vi "Omniax_mDrive_XYZR_MM_BR_RES_2_NC.vi"() -> ()   [LabVIEW 2009]
uses:
  <vilib>/Instr/_visa.llb/VISA Configure Serial Port (Instr).vi
panel:
  out "X Scan Duration":dbl
  out "Y Scan Duration":dbl
  out "Z Scan Duration":dbl
  out "R Scan Duration":dbl
  out "R Backlash steps/sec":i32
  out "R Backlash":i32
  out "R Holding Current %":i32
  out "R Run Current %":i32
  out "R offset deg":dbl
  out "R deg/rev":dbl
  out "R steps/rev":u32
  out "R velocity PV step/sec":i32
  out "R MINPOS":i32=-94296
  out "R MAXPOS":i32=-34296
  out "R COM PORT":refnum<visa-resource-name>="COM5"
  in  "R Scan set":bool
  in  "R Scan Velocity SP deg/sec":dbl
  in  "R Scan Length SP deg":dbl
  in  "R Move Set":bool
  out "Reset R Motor Steps":i32
  in  "Reset R Position deg":dbl
  out "R Velocity MVdeg/sec":dbl
  in  "R Velocity SP deg/sec":dbl
  in  "R Position SP deg":dbl
  out "R Position MV deg":dbl
  out "R Scan velocity MV deg/sec":dbl format="%#_6f"
  out "R Scan length MV deg":dbl
  in  "R Scan Length SP steps":i32 min=0 max=6144000 step=100
  in  "R Scan OK":bool
  in  "R Velocity SP step/sec":i32 min=1 max=102400
  in  "R Scan Velocity SP steps/sec":i32=1 min=1 max=102400 step=1
  in  "R Go":bool
  in  "R Step SP":i32=-20000 min=0 max=6144000 step=500
  out "R Position deg PV":dbl
  out "R Step PV":i32 max=2000
  out "R Backlash corr":bool
  out "R in Motion":bool
  out "R Scan":bool
  out "R in Range":bool
  out "Z COM PORT":refnum<visa-resource-name>="COM5"
  out "Z Backlash steps/sec":i32
  out "Z Backlash":i32
  out "Z Holding Current %":i32
  out "Z Run Current %":i32
  out "Z offset mm":dbl
  out "Z mm/rev":dbl
  out "Z steps/rev":u32
  out "Z  velocity PV step/sec":i32
  out "Z MINPOS":i32=-94296
  out "Z MAXPOS":i32=-34296
  in  "Z Scan set":bool
  in  "Z Scan Velocity SP mm/sec":dbl
  in  "Z Scan Length SP mm":dbl
  in  "Z Move Set":bool
  out "Reset Z Motor Steps":i32
  in  "Reset Z Position mm":dbl
  out "Z Velocity MV mm/sec":dbl
  in  "Z Velocity SP mm/sec":dbl
  in  "Z Position SP mm":dbl
  out "Z Position MV mm":dbl
  out "Z Scan velocity MV mm/sec":dbl format="%#_6f"
  out "Z Scan length MV mm":dbl
  in  "Z Scan Length SP steps":i32 min=0 max=2048000 step=100
  in  "Z Scan OK":bool
  in  "Z Velocity SP step/sec":i32 min=1 max=102400
  in  "Z Scan Velocity SP steps/sec":i32=1 min=1 max=102400 step=1
  in  "Z Go":bool
  in  "Z Step SP":i32=-20000 min=0 max=2048000 step=500
  out "Z Position mm PV":dbl
  out "Z Step PV":i32 max=2000
  out "Z Backlash corr":bool
  out "Z in Motion":bool
  out "Z Scan":bool
  out "Z in Range":bool
  out "Reset X Motor Steps":i32
  in  "Reset X Position mm":dbl
  out "X Backlash corr":bool
  out "X  in Motion":bool
  out "X Scan":bool
  out "X  in Range":bool
  out "X Step PV":i32 max=2000
  out "X Position mm PV":dbl
  out "X velocity PV step/sec":i32
  in  "X Scan set":bool
  in  "X Scan Velocity SP mm/sec":dbl
  in  "X Scan Length SP mm":dbl
  in  "X Move Set":bool
  out "X Velocity MV mm/sec":dbl
  in  "X Velocity SP mm/sec":dbl
  in  "X Position SP mm":dbl
  out "X Position MV mm":dbl
  out "X Scan velocity MV mm/sec":dbl format="%#_6f"
  out "X Scan length MV mm":dbl
  in  "X Scan Length SP steps":i32 min=-460800 max=460800 step=100
  in  "X Scan OK":bool
  in  "X Velocity SP step/sec":i32 min=1 max=102400
  in  "X Scan Velocity SP steps/sec":i32=1 min=1 max=102400 step=1
  in  "X Go":bool
  in  "X Step SP":i32=-20000 min=-460800 max=460800 step=500
  out "X Backlash steps/sec":i32
  out "X Backlash":i32
  out "X Holding Current %":i32
  out "X Run Current %":i32
  out "X offset mm":dbl
  out "X mm/rev":dbl
  out "X steps/rev":u32
  out "X MAXPOS":i32=-34296
  out "X MINPOS":i32=-94296
  out "X COM PORT":refnum<visa-resource-name>="COM5"
  out "Y Backlash corr":bool
  in  "Y Scan set":bool
  in  "Y Scan Velocity SP mm/sec":dbl
  in  "Y Scan Length SP mm":dbl
  in  "Y Move Set":bool
  out "Y Backlash steps/sec":i32
  out "Y Backlash":i32
  out "Y in Motion":bool
  in  "Reset":bool
  out "Reset Y Motor Steps":i32
  in  "Reset Y Position mm":dbl
  out "Y Velocity MV mm/sec":dbl
  in  "Y Velocity SP mm/sec":dbl
  in  "Y Position SP mm":dbl
  out "Y Position MV mm":dbl
  out "Y Holding Current %":i32
  out "Y Run Current %":i32
  out "Y Scan velocity MV mm/sec":dbl format="%#_6f"
  out "Y Scan length MV mm":dbl
  in  "Scan Cancel":bool
  out "Y Position mm PV":dbl
  out "Y offset mm":dbl
  out "Y mm/rev":dbl
  out "Y steps/rev":u32
  out "Y velocity PV step/sec":i32
  in  "Y Scan Length SP steps":i32 min=-460800 max=460800 step=100
  out "Y Scan":bool
  in  "Y Scan OK":bool
  in  "Scan Go":bool
  in  "Y Velocity SP step/sec":i32 min=1 max=102400
  in  "Y Scan Velocity SP steps/sec":i32=1 min=1 max=102400 step=1
  in  "Stop":bool
  out "Y in Range":bool
  out "Y Step PV":i32 max=2000
  in  "Y Go":bool
  in  "Y Step SP":i32=-20000 min=-460800 max=460800 step=500
  out "Y MINPOS":i32=-94296
  out "Y MAXPOS":i32=-34296
  out "Y COM PORT":refnum<visa-resource-name>="COM5"
  # "L"
  # "M"
  # "B"
  # "S"
  # "MX"
  # "MY"
  # "MZ"
  # "MR"
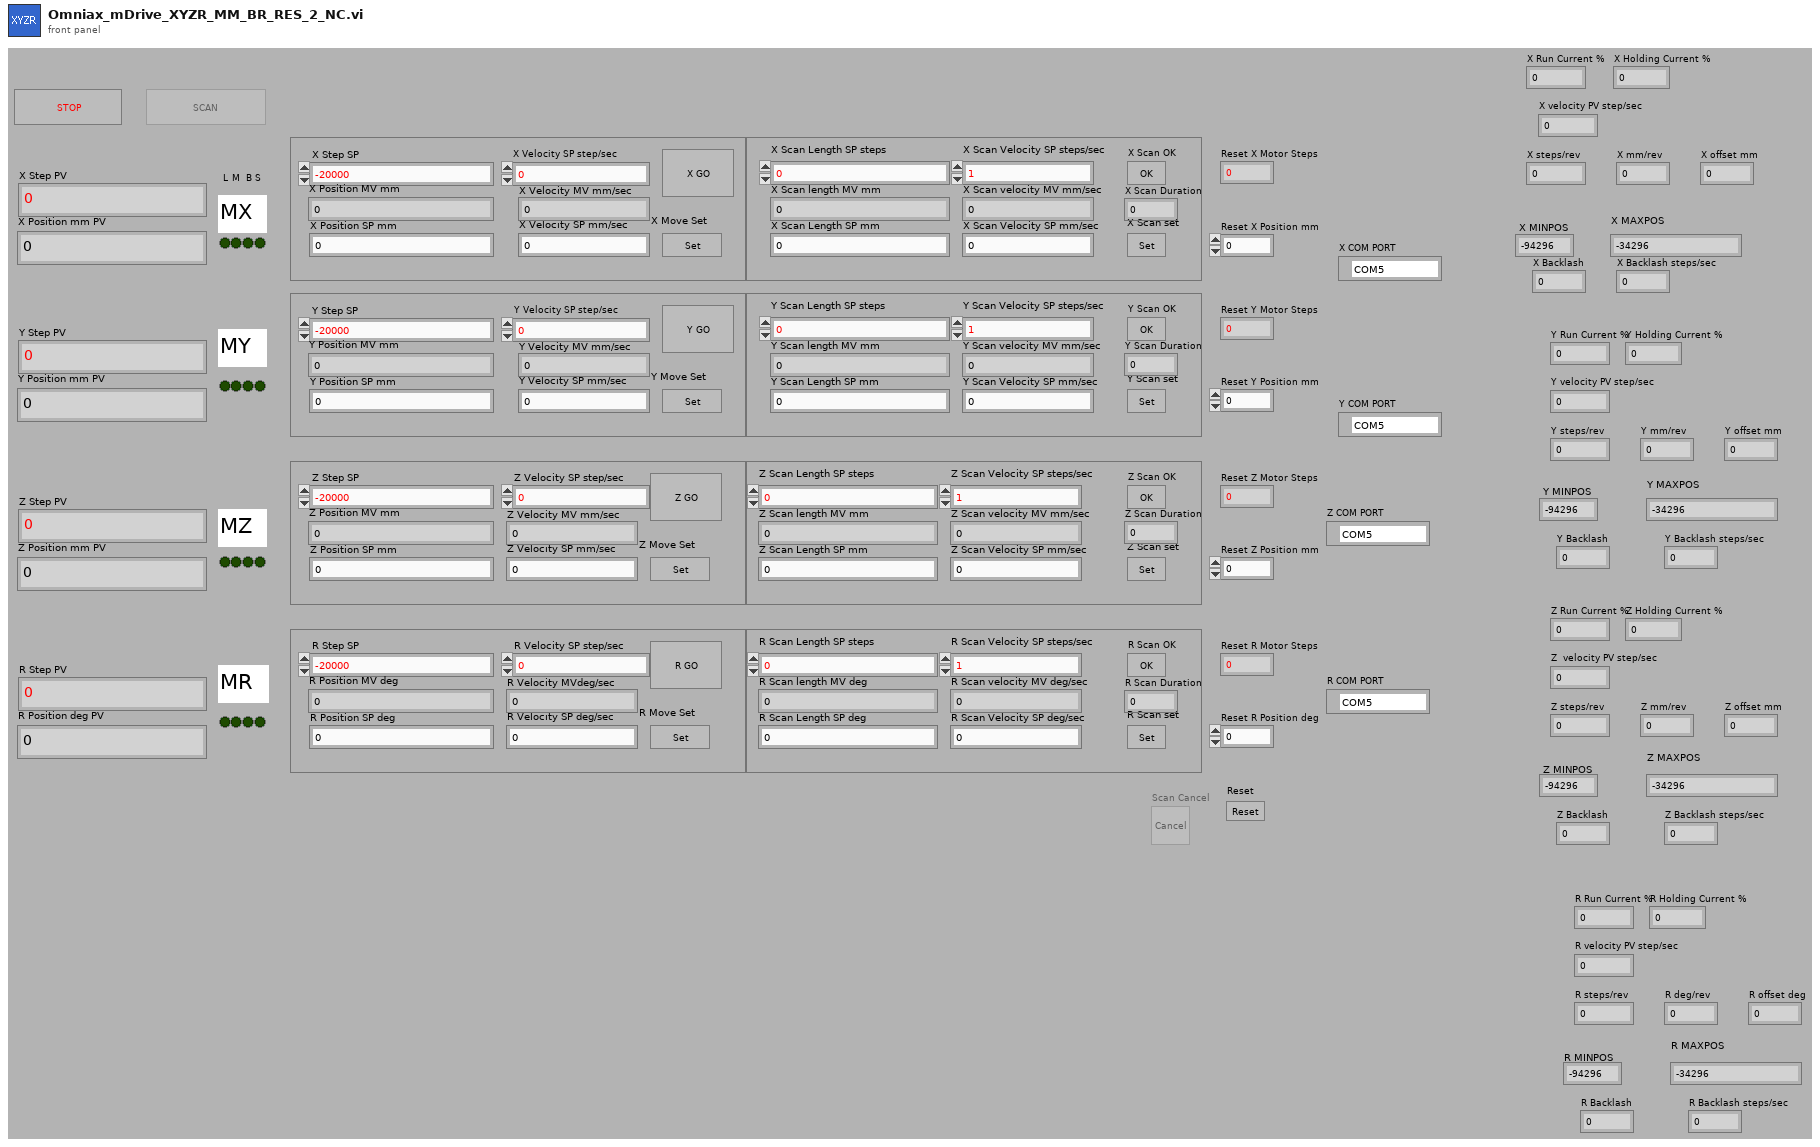
[diagram p1: front panel]
types:
  T1 = enum8{"Enabled", "Disabled", "Disabled and Grayed Out"}
  T2 = enum16{"Stop", "Reset", "Run Current", "Holding Current", "Accel Rate", "Decel Rate", "Move to Relative Position", "Move to Absolute Position", "Echo Mode", "Print Parameter", "Send String", "Microstep Resolution", "Set Current Position", "Max Velocity"}
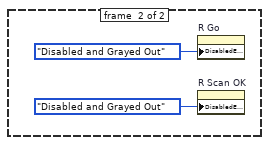
[diagram p2: hidden frame]
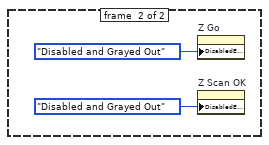
[diagram p5: hidden frame]
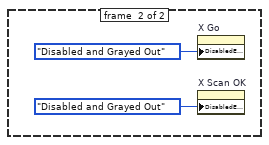
[diagram p8: hidden frame]
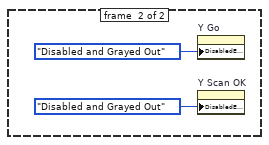
[diagram p11: hidden frame]
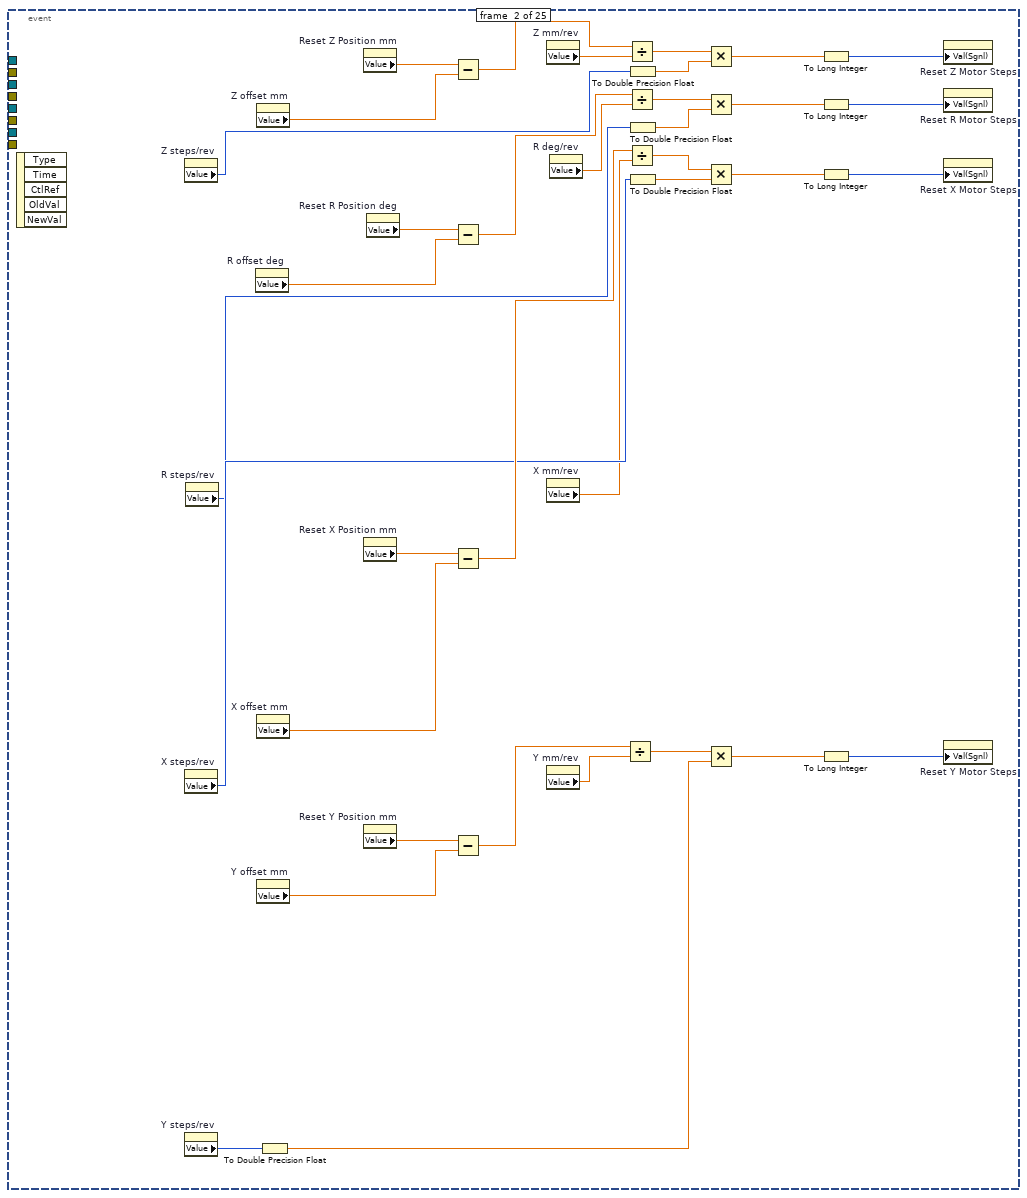
[diagram p14: hidden frame]
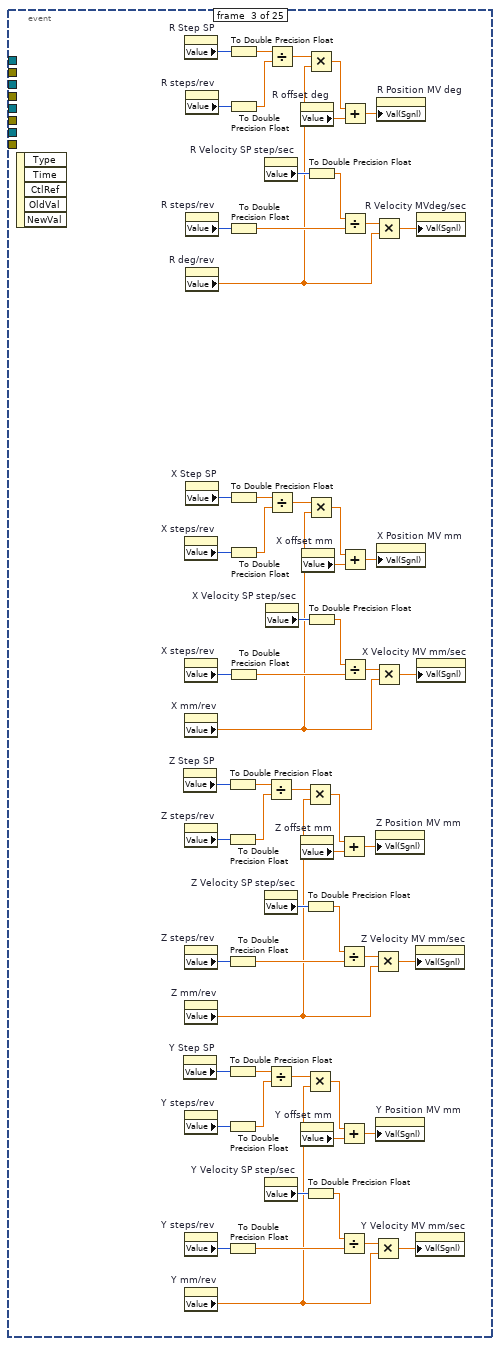
[diagram p15: hidden frame]
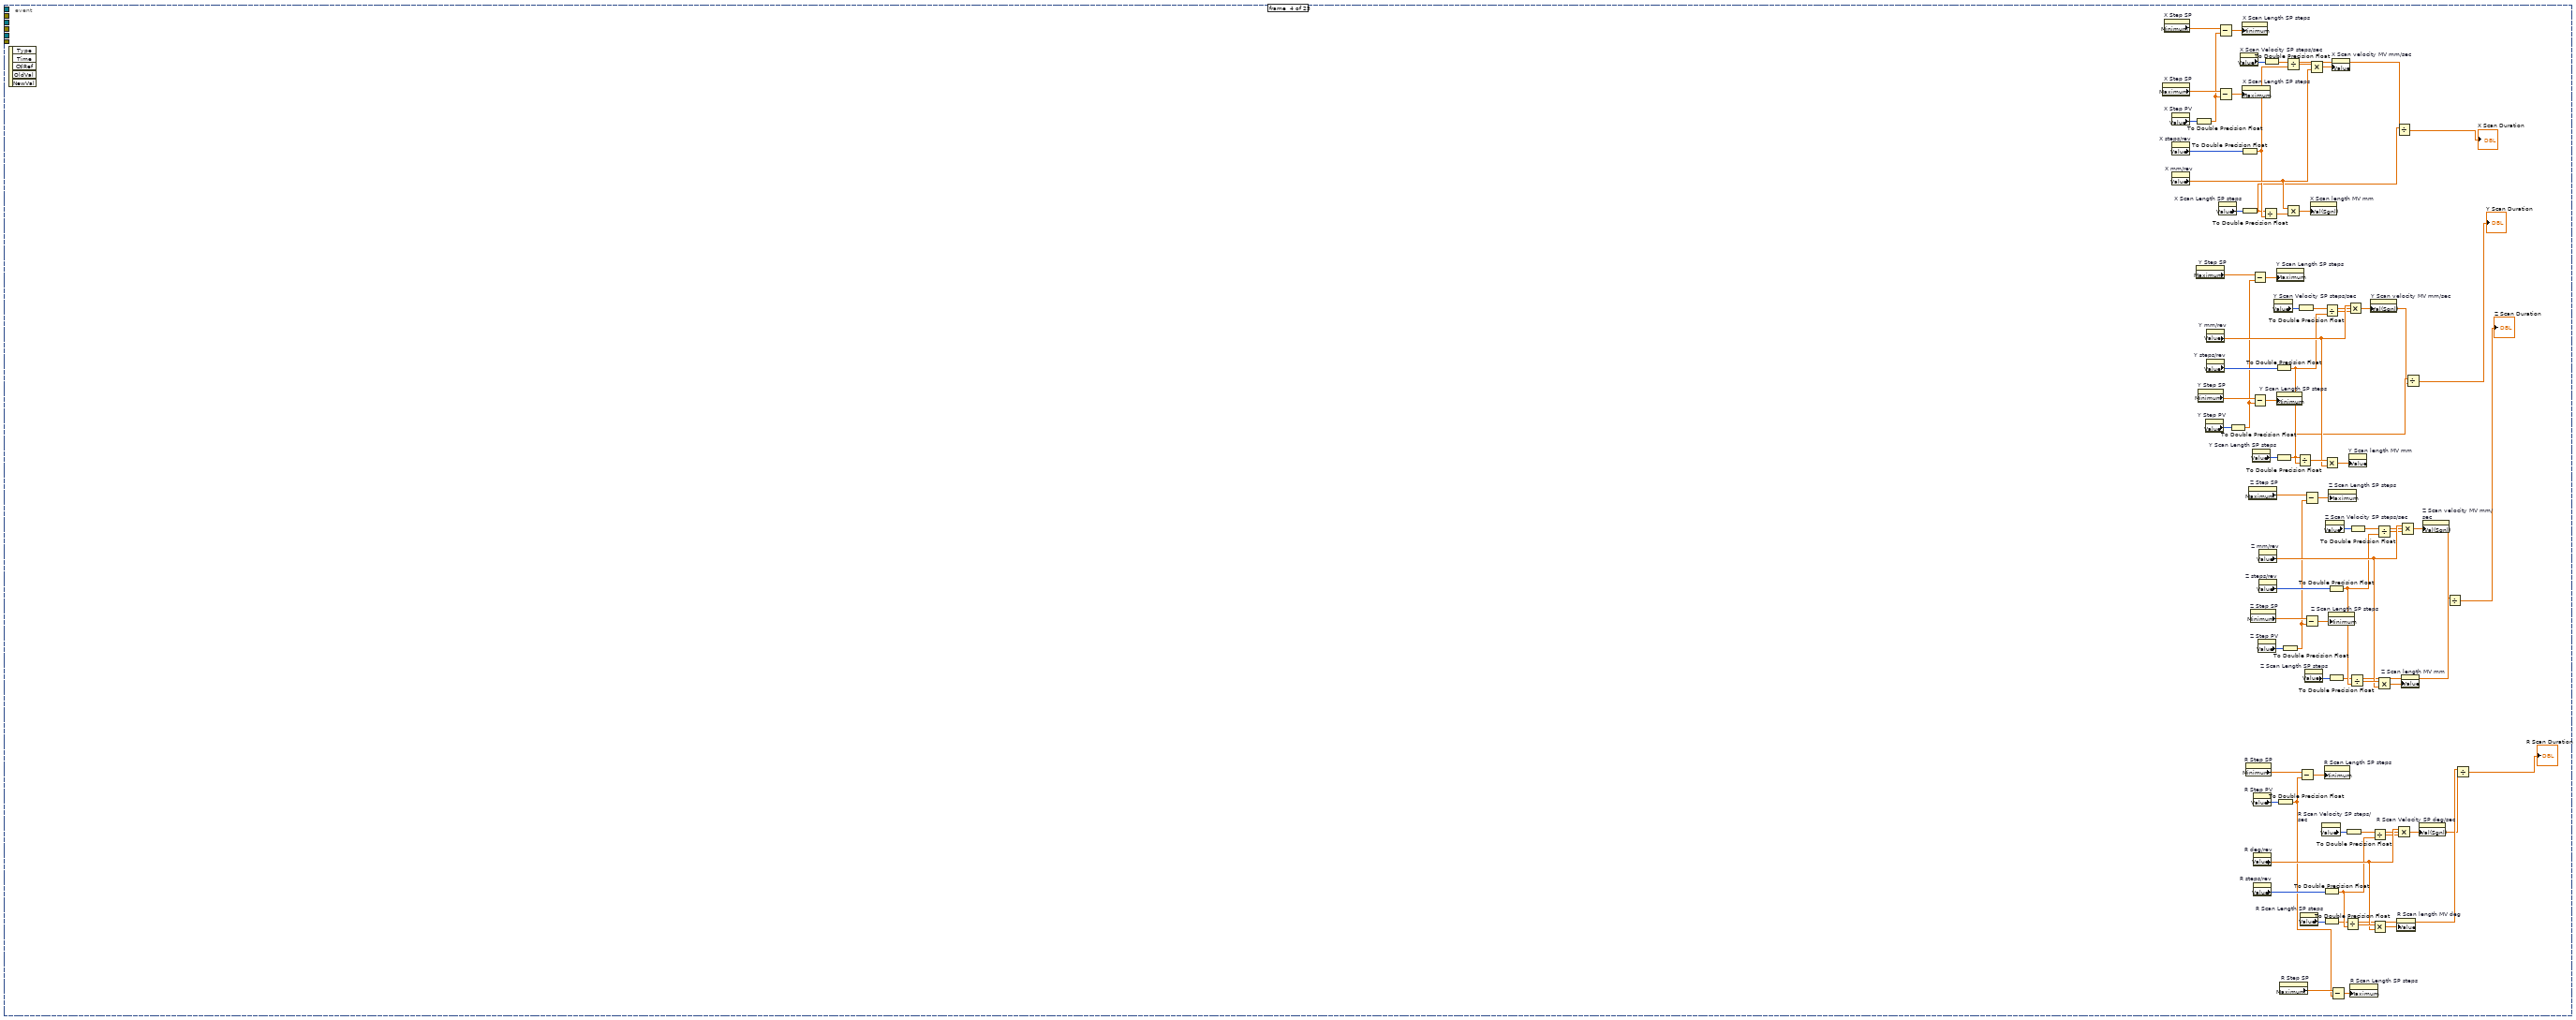
[diagram p16: hidden frame]
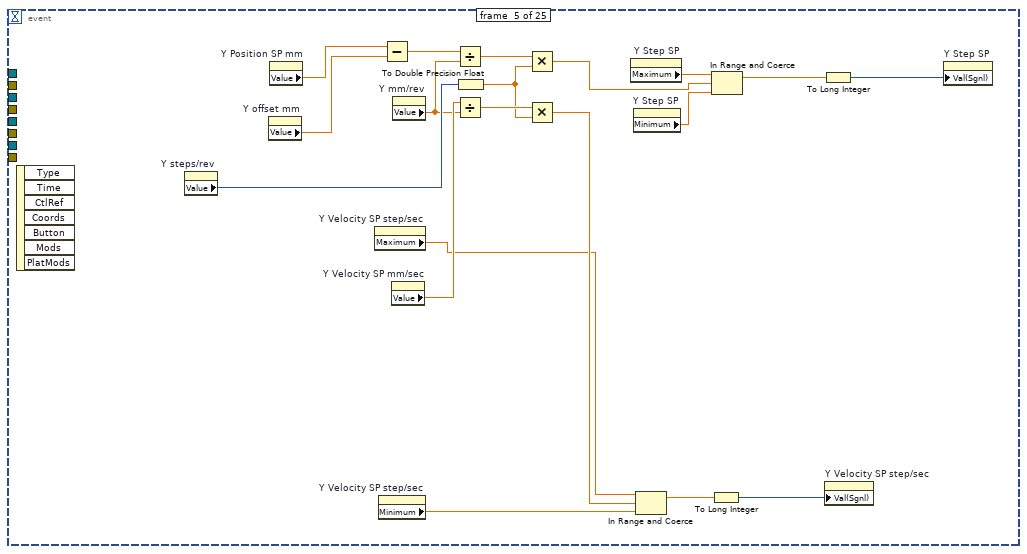
[diagram p17: hidden frame]
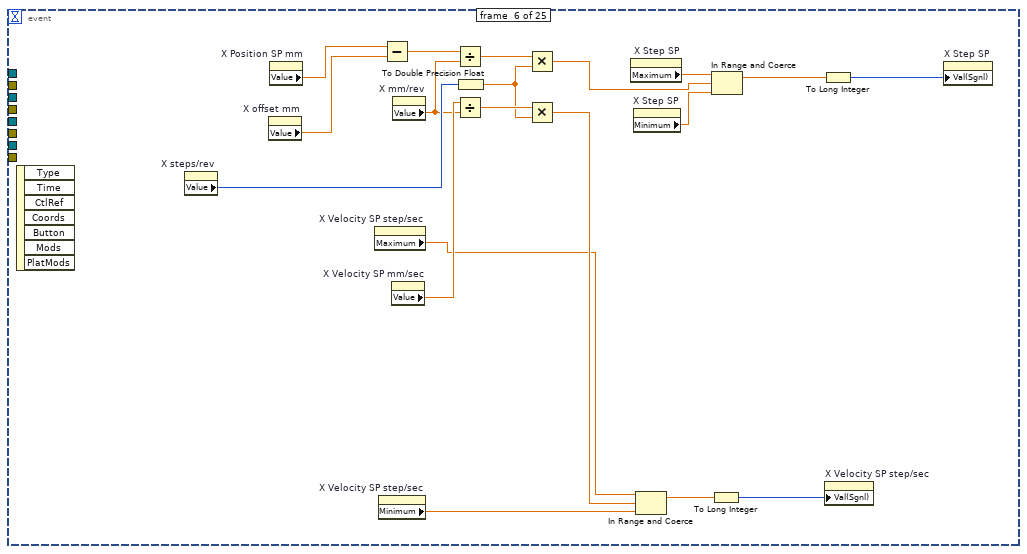
[diagram p18: hidden frame]
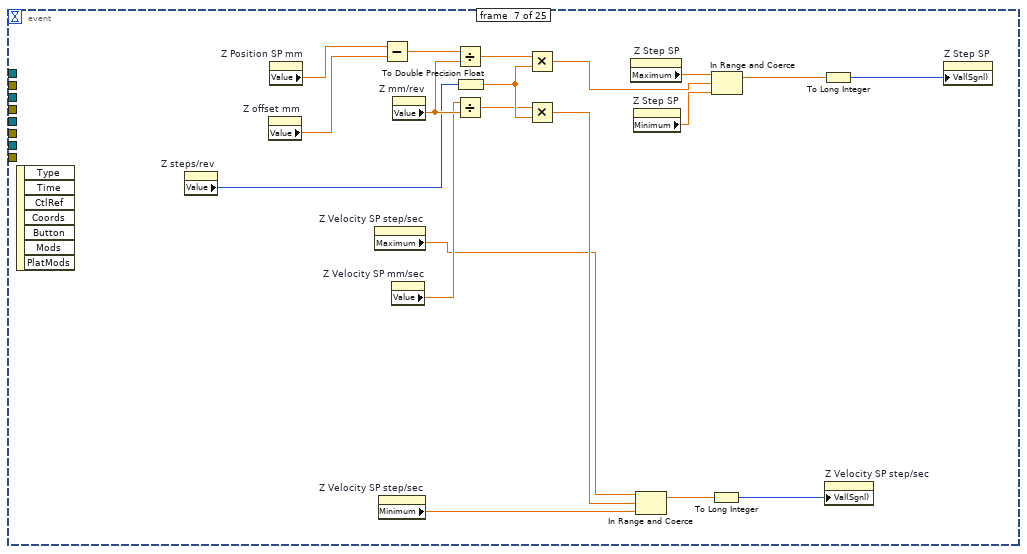
[diagram p19: hidden frame]
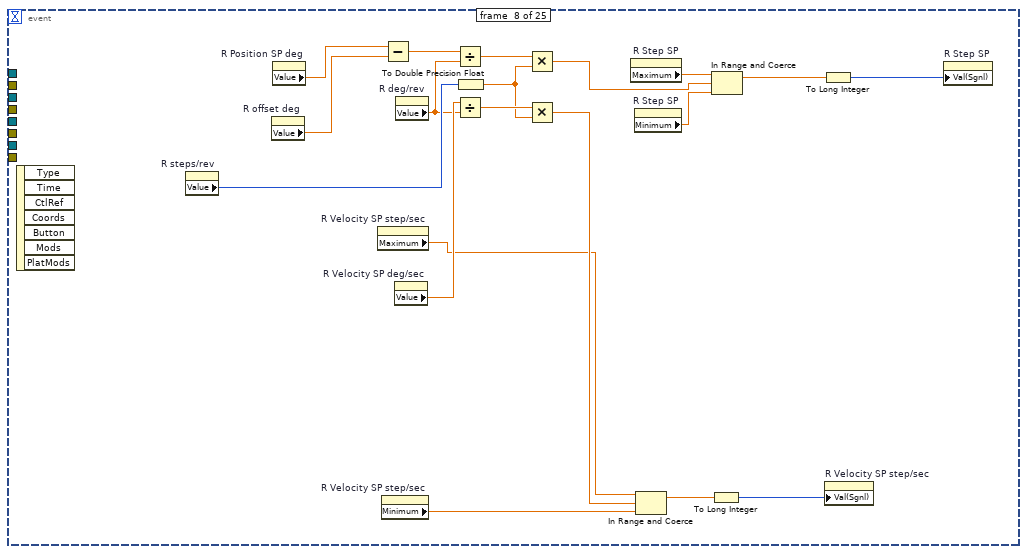
[diagram p20: hidden frame]
diagram:
  w19 = refnum<visa-resource-name> "COM11" ("COM PORT")
  w21 = u16 0 items=["None", "XON/XOFF", "RTS/CTS", "XON/XOFF & RTS/CTS", "DTR/DSR", "XON/XOFF & DTR/DSR"] ("flow control (0:none)")
  w22 = u16 10 items=["1.0"=10, "1.5"=15, "2.0"=20] ("stop bits (10: 1 bit)")
  w52 = refnum<visa-resource-name> "COM10" ("COM PORT")
  w54 = u16 0 items=["None", "XON/XOFF", "RTS/CTS", "XON/XOFF & RTS/CTS", "DTR/DSR", "XON/XOFF & DTR/DSR"] ("flow control (0:none)")
  w55 = u16 10 items=["1.0"=10, "1.5"=15, "2.0"=20] ("stop bits (10: 1 bit)")
  w65 = refnum<visa-resource-name> "COM8" ("COM PORT")
  w67 = u16 0 items=["None", "XON/XOFF", "RTS/CTS", "XON/XOFF & RTS/CTS", "DTR/DSR", "XON/XOFF & DTR/DSR"] ("flow control (0:none)")
  w68 = u16 10 items=["1.0"=10, "1.5"=15, "2.0"=20] ("stop bits (10: 1 bit)")
  w90 = refnum<visa-resource-name> "COM9" ("COM PORT")
  w92 = u16 0 items=["None", "XON/XOFF", "RTS/CTS", "XON/XOFF & RTS/CTS", "DTR/DSR", "XON/XOFF & DTR/DSR"] ("flow control (0:none)")
  w93 = u16 10 items=["1.0"=10, "1.5"=15, "2.0"=20] ("stop bits (10: 1 bit)")
  # "Stop bits"
  # "Stop bits"
  # "Stop bits"
  # "Stop bits"
  n1 = flat-sequence {
    frame #0 {
      w101 = 3.0 ("R deg/rev")
      w99 = u32 51200 ("step/rev")
      w103 = 102400 ("Value (Signaling)")
      n2 = property on="R Velocity SP step/sec" class="DigNum (strict)"("Val(Sgnl)"=w103) -> ()  [unwired: 2 in, 2 out]
      n3 = property on="R Velocity SP step/sec" class="DigNum (strict)"("Minimum"=1.0 ("Data Entry Limits:Minimum")) -> ()  [unwired: 2 in, 2 out]
      n4 = To Double Precision Float(number=w99) -> (double precision float=w100:dbl)
      n5 = To Double Precision Float(number=w103) -> (double precision float=w105:dbl)
      n6 = Divide(x=w105, y=w100) -> (x/y=w104:dbl)
      n7 = property on="R Velocity SP step/sec" class="DigNum (strict)"("Maximum"=w105) -> ()  [unwired: 2 in, 2 out]
      n8 = Multiply(x=w104, y=w101) -> (x*y=w102:dbl)
      n9 = property on="R Velocity SP deg/sec" class="DigNum (strict)"("Val(Sgnl)"=w102) -> ()  [unwired: 2 in, 2 out]
      "R offset deg" <- 0.0 ("R offset deg")
      "R deg/rev" <- w101
      "R steps/rev" <- w99
    }
  }
  n10 = flat-sequence {
    frame #0 {
      w108 = 1.0 ("MM/rev")
      w111 = u32 51200 ("step/rev")
      w106 = 102400 ("Value (Signaling)")
      n11 = property on="X Velocity SP step/sec" class="DigNum (strict)"("Minimum"=1.0 ("Data Entry Limits:Minimum")) -> ()  [unwired: 2 in, 2 out]
      n12 = property on="X Velocity SP step/sec" class="DigNum (strict)"("Val(Sgnl)"=w106) -> ()  [unwired: 2 in, 2 out]
      n13 = To Double Precision Float(number=w111) -> (double precision float=w110:dbl)
      n14 = To Double Precision Float(number=w106) -> (double precision float=w112:dbl)
      n15 = Divide(x=w112, y=w110) -> (x/y=w107:dbl)
      n16 = property on="X Velocity SP step/sec" class="DigNum (strict)"("Maximum"=w112) -> ()  [unwired: 2 in, 2 out]
      n17 = Multiply(x=w107, y=w108) -> (x*y=w109:dbl)
      n18 = property on="X Velocity SP mm/sec" class="DigNum (strict)"("Val(Sgnl)"=w109) -> ()  [unwired: 2 in, 2 out]
      "X offset mm" <- 0.0 ("offset")
      "X steps/rev" <- w111
      "X mm/rev" <- w108
    }
  }
  n19 = flat-sequence {
    frame #0 {
      w116 = 1.0 ("Z mm/rev")
      w115 = u32 51200 ("step/rev")
      w117 = 102400 ("Value (Signaling)")
      n20 = property on="Z Velocity SP step/sec" class="DigNum (strict)"("Val(Sgnl)"=w117) -> ()  [unwired: 2 in, 2 out]
      n21 = property on="Z Velocity SP step/sec" class="DigNum (strict)"("Minimum"=1.0 ("Data Entry Limits:Minimum")) -> ()  [unwired: 2 in, 2 out]
      n22 = To Double Precision Float(number=w115) -> (double precision float=w120:dbl)
      n23 = To Double Precision Float(number=w117) -> (double precision float=w121:dbl)
      n24 = Divide(x=w121, y=w120) -> (x/y=w118:dbl)
      n25 = property on="Z Velocity SP step/sec" class="DigNum (strict)"("Maximum"=w121) -> ()  [unwired: 2 in, 2 out]
      n26 = Multiply(x=w118, y=w116) -> (x*y=w119:dbl)
      n27 = property on="Z Velocity SP mm/sec" class="DigNum (strict)"("Val(Sgnl)"=w119) -> ()  [unwired: 2 in, 2 out]
      "Z offset mm" <- 0.0 ("Z offset mm")
      "Z mm/rev" <- w116
      "Z steps/rev" <- w115
    }
  }
  n28 = flat-sequence {
    frame #0 {
      n29 = property on="X Backlash corr" class="Bool (strict)"("Val(Sgnl)"=FALSE ("Value (Signaling)")) -> ()  [unwired: 2 in, 2 out]
      n30 = property on="Z Backlash corr" class="Bool (strict)"("Val(Sgnl)"=FALSE ("Value (Signaling)")) -> ()  [unwired: 2 in, 2 out]
      n31 = property on="Y Backlash corr" class="Bool (strict)"("Val(Sgnl)"=FALSE ("Value (Signaling)")) -> ()  [unwired: 2 in, 2 out]
      n32 = property on="R Backlash corr" class="Bool (strict)"("Val(Sgnl)"=FALSE ("Value (Signaling)")) -> ()  [unwired: 2 in, 2 out]
      "Z Backlash steps/sec" <- 25600 ("Z Backlash steps/sec")
      "Z Backlash" <- -12800 ("Z Backlash")
      "X Backlash steps/sec" <- 25600 ("Value (Signaling)")
      "X Backlash" <- -5120 ("Backlash2")
      "Y Backlash" <- -5120 ("Backlash2")
      "Y Backlash steps/sec" <- 25600 ("Value (Signaling)")
      "R Backlash steps/sec" <- 25600 ("R Backlash steps/sec")
      "R Backlash" <- -12800 ("R Backlash")
    }
  }
  n33 = flat-sequence {
    frame #0 {
      "Z Holding Current %" <- 20 ("Z Holding Current %")
      "Z Run Current %" <- 40 ("Z Run Current %")
      "X Run Current %" <- 40 ("Run Current %")
      "X Holding Current %" <- 20 ("Holding Current %")
      "Y Run Current %" <- 40 ("Run Current %")
      "Y Holding Current %" <- 20 ("Holding Current %")
      "R Holding Current %" <- 20 ("R Holding Current %")
      "R Run Current %" <- 40 ("R Run Current %")
    }
  }
  n34 = flat-sequence {
    frame #0 {
      n35 = property on="Y Scan" class="Bool (strict)"("Val(Sgnl)"=FALSE ("Value (Signaling)")) -> ()  [unwired: 2 in, 2 out]
      n36 = property on="Y Scan Velocity SP mm/sec" class="DigNum (strict)"("Val(Sgnl)"=0.1 ("Value (Signaling)")) -> ()  [unwired: 2 in, 2 out]
      n37 = property on="Z Scan Velocity SP mm/sec" class="DigNum (strict)"("Val(Sgnl)"=0.1 ("Value (Signaling)")) -> ()  [unwired: 2 in, 2 out]
      n38 = property on="R Scan" class="Bool (strict)"("Val(Sgnl)"=FALSE ("Value (Signaling)")) -> ()  [unwired: 2 in, 2 out]
      n39 = property on="Z Scan" class="Bool (strict)"("Val(Sgnl)"=FALSE ("Value (Signaling)")) -> ()  [unwired: 2 in, 2 out]
      n40 = property on="R Velocity SP deg/sec" class="DigNum (strict)"("Val(Sgnl)"=0.1 ("Value (Signaling)")) -> ()  [unwired: 2 in, 2 out]
      n41 = property on="X Scan" class="Bool (strict)"("Val(Sgnl)"=FALSE ("Value (Signaling)")) -> ()  [unwired: 2 in, 2 out]
      n42 = property on="X Scan Velocity SP mm/sec" class="DigNum (strict)"("Val(Sgnl)"=0.1 ("Value (Signaling)")) -> ()  [unwired: 2 in, 2 out]
      n43 = property on="Scan Go" class="Bool"("DisabledEnum"=T1."Disabled and Grayed Out" ("Disabled")) -> ()  [unwired: 2 in, 2 out]
      n44 = property on="Scan Cancel" class="Bool"("DisabledEnum"=T1."Disabled and Grayed Out" ("Disabled")) -> ()  [unwired: 2 in, 2 out]
    }
  }
  n45 = flat-sequence {
    frame #0 {
      w156 = 1.0 ("MM/rev")
      w159 = u32 51200 ("step/rev")
      w154 = 102400 ("Value (Signaling)")
      n46 = property on="Y Velocity SP step/sec" class="DigNum (strict)"("Minimum"=1.0 ("Data Entry Limits:Minimum")) -> ()  [unwired: 2 in, 2 out]
      n47 = property on="Y Velocity SP step/sec" class="DigNum (strict)"("Val(Sgnl)"=w154) -> ()  [unwired: 2 in, 2 out]
      n48 = To Double Precision Float(number=w159) -> (double precision float=w158:dbl)
      n49 = To Double Precision Float(number=w154) -> (double precision float=w160:dbl)
      n50 = Divide(x=w160, y=w158) -> (x/y=w155:dbl)
      n51 = property on="Y Velocity SP step/sec" class="DigNum (strict)"("Maximum"=w160) -> ()  [unwired: 2 in, 2 out]
      n52 = Multiply(x=w155, y=w156) -> (x*y=w157:dbl)
      n53 = property on="Y Velocity SP mm/sec" class="DigNum (strict)"("Val(Sgnl)"=w157) -> ()  [unwired: 2 in, 2 out]
      "Y offset mm" <- 0.0 ("offset")
      "Y steps/rev" <- w159
      "Y mm/rev" <- w156
    }
  }
  n54 = call-poly "VISA Configure Serial Port"("VISA resource name"=w90, "timeout (10sec)"=u32 10000, "baud rate (9600)"=u32 9600, "data bits (8)"=u16 8, "parity (0:none)"=enum16{"None", "Odd", "Even", "Mark", "Space"}."None", "stop bits (10: 1 bit)"=w93, "flow control (0:none)"=w92) -> ("VISA resource name out"=w83:refnum<visa-resource-name>, "error out"=w82:errorcluster)  [unwired: 7 in]
  n55 = flat-sequence {
    tunnel: w82 -> [w164]
    tunnel: w83 -> [w166]
    tunnel: [w165] -> w4
    tunnel: [w163] -> w3
    tunnel: [w172] -> w81
    tunnel: [w174] -> w79
    tunnel: w4 -> [w173]
    tunnel: w3 -> [w175]
    tunnel: w81 -> [w182]
    tunnel: [w181] -> w80
    tunnel: w79 -> [w179]
    tunnel: [w180] -> w78
    tunnel: [w192] -> w85
    tunnel: [w193] -> w84
    tunnel: w80 -> [w191]
    tunnel: w78 -> [w190]
    tunnel: w85 -> [w203]
    tunnel: w84 -> [w202]
    tunnel: [w205] -> w51
    tunnel: [w204] -> w50
    tunnel: [w199] -> w49
    tunnel: [w210] -> w88
    tunnel: [w211] -> w89
    tunnel: w51 -> [w211]
    tunnel: w50 -> [w210]
    tunnel: w49 -> [w206]
    frame #0 {
      n56 = call "mDrive Send Command.vi"("error in (no error)"=w164, "Extra"="EM=2", "Command"=T2."Send String", "VISA resource name"=w166) -> ("error out"=w163:errorcluster, "VISA resource name out"=w165:refnum<visa-resource-name>)  [unwired: 3 in, 1 out]
    }
    frame #1 {
      # "Run Current %"
      n57 = property on="Y Run Current %" class="DigNum (strict)"() -> ("Value"=w170:i32)  [unwired: 2 in, 2 out]
      n58 = Number To Decimal String(number=w170) -> (decimal integer string=w171:string)  [unwired: 1 in]
      n59 = call "mDrive Send Command.vi"("error in (no error)"=w175, "Extra"=w171, "Command"=T2."Run Current", "VISA resource name"=w173) -> ("error out"=w174:errorcluster, "VISA resource name out"=w172:refnum<visa-resource-name>)  [unwired: 3 in, 1 out]
    }
    frame #2 {
      # "Holding Current %"
      n60 = property on="Y Holding Current %" class="DigNum (strict)"() -> ("Value"=w177:i32)  [unwired: 2 in, 2 out]
      n61 = Number To Decimal String(number=w177) -> (decimal integer string=w178:string)  [unwired: 1 in]
      n62 = call "mDrive Send Command.vi"("error in (no error)"=w179, "Extra"=w178, "Command"=T2."Holding Current", "VISA resource name"=w182) -> ("error out"=w180:errorcluster, "VISA resource name out"=w181:refnum<visa-resource-name>)  [unwired: 3 in, 1 out]
    }
    frame #3 {
      # "Print Velocity Ma"
      # "Velocity Max"
      n63 = property on="Y Velocity SP step/sec" class="DigNum (strict)"() -> ("Value"=w189:i32)  [unwired: 2 in, 2 out]
      n64 = Number To Decimal String(number=w189) -> (decimal integer string=w188:string)  [unwired: 1 in]
      n65 = call "mDrive Send Command.vi"("error in (no error)"=w190, "Extra"=w188, "Command"=T2."Max Velocity", "VISA resource name"=w191) -> ("error out"=w186:errorcluster, "VISA resource name out"=w196:refnum<visa-resource-name>)  [unwired: 3 in, 1 out]
      n66 = call "mDrive Send Command.vi"("error in (no error)"=w186, "Extra"="VM", "Command"=T2."Print Parameter", "VISA resource name"=w196) -> ("error out"=w193:errorcluster, "read buffer"=w194:string, "VISA resource name out"=w192:refnum<visa-resource-name>)  [unwired: 3 in]
      n67 = Decimal String To Number(string=w194, offset=0) -> (number=w187:i32)  [unwired: 1 in, 1 out]
      n68 = property on="Y scan velocity MV step/sec" class="DigNum (strict)"("Val(Sgnl)"=w187) -> ()  [unwired: 2 in, 2 out]
    }
    frame #4 {
      # "PRINT POSITION"
      n69 = call "mDrive Send Command.vi"("error in (no error)"=w202, "Extra"="P", "Command"=T2."Print Parameter", "VISA resource name"=w203) -> ("error out"=w204:errorcluster, "read buffer"=w201:string, "VISA resource name out"=w205:refnum<visa-resource-name>)  [unwired: 3 in]
      n70 = Decimal String To Number(string=w201, offset=0) -> (number=w199:i32)  [unwired: 1 in, 1 out]
    }
    frame #5 {
      w208 = -460800 ("lower limit")
      w209 = 460800 ("upper limit")
      n71 = property on="Y Step SP" class="DigNum (strict)"("Val(Sgnl)"=w206) -> ()  [unwired: 2 in, 2 out]
      n72 = property on="Y Step SP" class="DigNum (strict)"("Maximum"=w209) -> ()  [unwired: 2 in, 2 out]
      n73 = property on="Y Step SP" class="DigNum (strict)"("Minimum"=w208) -> ()  [unwired: 2 in, 2 out]
      n74 = In Range and Coerce(upper limit=w209, x=w206, lower limit=w208) -> (In Range?=w207:bool)  [unwired: 1 out]
      n75 = property on="Y in Range" class="Bool (strict)"("Val(Sgnl)"=w207) -> ()  [unwired: 2 in, 2 out]
      "Y MINPOS" <- w208
      "Y MAXPOS" <- w209
    }
  }
  n76 = call-poly "VISA Configure Serial Port"("VISA resource name"=w65, "timeout (10sec)"=u32 10000, "baud rate (9600)"=u32 9600, "data bits (8)"=u16 8, "parity (0:none)"=enum16{"None", "Odd", "Even", "Mark", "Space"}."None", "stop bits (10: 1 bit)"=w68, "flow control (0:none)"=w67) -> ("VISA resource name out"=w64:refnum<visa-resource-name>, "error out"=w63:errorcluster)  [unwired: 7 in]
  n77 = call-poly "VISA Configure Serial Port"("VISA resource name"=w19, "timeout (10sec)"=u32 10000, "baud rate (9600)"=u32 9600, "data bits (8)"=u16 8, "parity (0:none)"=enum16{"None", "Odd", "Even", "Mark", "Space"}."None", "stop bits (10: 1 bit)"=w22, "flow control (0:none)"=w21) -> ("VISA resource name out"=w18:refnum<visa-resource-name>, "error out"=w17:errorcluster)  [unwired: 7 in]
  n78 = call-poly "VISA Configure Serial Port"("VISA resource name"=w52, "timeout (10sec)"=u32 10000, "baud rate (9600)"=u32 9600, "data bits (8)"=u16 8, "parity (0:none)"=enum16{"None", "Odd", "Even", "Mark", "Space"}."None", "stop bits (10: 1 bit)"=w55, "flow control (0:none)"=w54) -> ("VISA resource name out"=w36:refnum<visa-resource-name>, "error out"=w35:errorcluster)  [unwired: 7 in]
  n79 = flat-sequence {
    tunnel: w63 -> [w213]
    tunnel: w64 -> [w215]
    tunnel: [w214] -> w2
    tunnel: [w212] -> w1
    tunnel: [w221] -> w77
    tunnel: [w223] -> w76
    tunnel: w2 -> [w222]
    tunnel: w1 -> [w224]
    tunnel: w77 -> [w231]
    tunnel: [w230] -> w75
    tunnel: w76 -> [w228]
    tunnel: [w229] -> w74
    tunnel: [w241] -> w73
    tunnel: [w242] -> w72
    tunnel: w75 -> [w240]
    tunnel: w74 -> [w239]
    tunnel: w73 -> [w252]
    tunnel: w72 -> [w251]
    tunnel: [w254] -> w48
    tunnel: [w253] -> w47
    tunnel: [w248] -> w46
    tunnel: [w259] -> w61
    tunnel: [w260] -> w62
    tunnel: w48 -> [w260]
    tunnel: w47 -> [w259]
    tunnel: w46 -> [w255]
    frame #0 {
      n80 = call "mDrive Send Command.vi"("error in (no error)"=w213, "Extra"="EM=2", "Command"=T2."Send String", "VISA resource name"=w215) -> ("error out"=w212:errorcluster, "VISA resource name out"=w214:refnum<visa-resource-name>)  [unwired: 3 in, 1 out]
    }
    frame #1 {
      # "Run Current %"
      n81 = property on="X Run Current %" class="DigNum (strict)"() -> ("Value"=w219:i32)  [unwired: 2 in, 2 out]
      n82 = Number To Decimal String(number=w219) -> (decimal integer string=w220:string)  [unwired: 1 in]
      n83 = call "mDrive Send Command.vi"("error in (no error)"=w224, "Extra"=w220, "Command"=T2."Run Current", "VISA resource name"=w222) -> ("error out"=w223:errorcluster, "VISA resource name out"=w221:refnum<visa-resource-name>)  [unwired: 3 in, 1 out]
    }
    frame #2 {
      # "Holding Current %"
      n84 = property on="X Holding Current %" class="DigNum (strict)"() -> ("Value"=w226:i32)  [unwired: 2 in, 2 out]
      n85 = Number To Decimal String(number=w226) -> (decimal integer string=w227:string)  [unwired: 1 in]
      n86 = call "mDrive Send Command.vi"("error in (no error)"=w228, "Extra"=w227, "Command"=T2."Holding Current", "VISA resource name"=w231) -> ("error out"=w229:errorcluster, "VISA resource name out"=w230:refnum<visa-resource-name>)  [unwired: 3 in, 1 out]
    }
    frame #3 {
      # "Print Velocity Ma"
      # "Velocity Max"
      n87 = property on="X Velocity SP step/sec" class="DigNum (strict)"() -> ("Value"=w238:i32)  [unwired: 2 in, 2 out]
      n88 = Number To Decimal String(number=w238) -> (decimal integer string=w237:string)  [unwired: 1 in]
      n89 = call "mDrive Send Command.vi"("error in (no error)"=w239, "Extra"=w237, "Command"=T2."Max Velocity", "VISA resource name"=w240) -> ("error out"=w235:errorcluster, "VISA resource name out"=w245:refnum<visa-resource-name>)  [unwired: 3 in, 1 out]
      n90 = call "mDrive Send Command.vi"("error in (no error)"=w235, "Extra"="VM", "Command"=T2."Print Parameter", "VISA resource name"=w245) -> ("error out"=w242:errorcluster, "read buffer"=w243:string, "VISA resource name out"=w241:refnum<visa-resource-name>)  [unwired: 3 in]
      n91 = Decimal String To Number(string=w243, offset=0) -> (number=w236:i32)  [unwired: 1 in, 1 out]
      n92 = property on="X velocity PV step/sec" class="DigNum (strict)"("Val(Sgnl)"=w236) -> ()  [unwired: 2 in, 2 out]
    }
    frame #4 {
      # "PRINT POSITION"
      n93 = call "mDrive Send Command.vi"("error in (no error)"=w251, "Extra"="P", "Command"=T2."Print Parameter", "VISA resource name"=w252) -> ("error out"=w253:errorcluster, "read buffer"=w250:string, "VISA resource name out"=w254:refnum<visa-resource-name>)  [unwired: 3 in]
      n94 = Decimal String To Number(string=w250, offset=0) -> (number=w248:i32)  [unwired: 1 in, 1 out]
    }
    frame #5 {
      w257 = -460800 ("lower limit")
      w258 = 460800 ("upper limit")
      n95 = property on="X Step SP" class="DigNum (strict)"("Val(Sgnl)"=w255) -> ()  [unwired: 2 in, 2 out]
      n96 = property on="X Step SP" class="DigNum (strict)"("Maximum"=w258) -> ()  [unwired: 2 in, 2 out]
      n97 = property on="X Step SP" class="DigNum (strict)"("Minimum"=w257) -> ()  [unwired: 2 in, 2 out]
      n98 = In Range and Coerce(upper limit=w258, x=w255, lower limit=w257) -> (In Range?=w256:bool)  [unwired: 1 out]
      n99 = property on="X  in Range" class="Bool (strict)"("Val(Sgnl)"=w256) -> ()  [unwired: 2 in, 2 out]
      "X MINPOS" <- w257
      "X MAXPOS" <- w258
    }
  }
  n100 = flat-sequence {
    tunnel: w17 -> [w264]
    tunnel: w18 -> [w262]
    tunnel: [w261] -> w8
    tunnel: [w263] -> w7
    tunnel: [w271] -> w34
    tunnel: [w273] -> w33
    tunnel: w8 -> [w272]
    tunnel: w7 -> [w267]
    tunnel: w34 -> [w280]
    tunnel: [w279] -> w32
    tunnel: w33 -> [w277]
    tunnel: [w278] -> w31
    tunnel: [w290] -> w30
    tunnel: [w291] -> w29
    tunnel: w32 -> [w289]
    tunnel: w31 -> [w288]
    tunnel: w30 -> [w301]
    tunnel: w29 -> [w300]
    tunnel: [w303] -> w28
    tunnel: [w302] -> w27
    tunnel: [w297] -> w26
    tunnel: [w308] -> w11
    tunnel: [w309] -> w12
    tunnel: w28 -> [w309]
    tunnel: w27 -> [w308]
    tunnel: w26 -> [w306]
    frame #0 {
      n101 = call "mDrive Send Command.vi"("error in (no error)"=w264, "Extra"="EM=2", "Command"=T2."Send String", "VISA resource name"=w262) -> ("error out"=w263:errorcluster, "VISA resource name out"=w261:refnum<visa-resource-name>)  [unwired: 3 in, 1 out]
    }
    frame #1 {
      # "Run Current %"
      n102 = property on="R Run Current %" class="DigNum (strict)"() -> ("Value"=w269:i32)  [unwired: 2 in, 2 out]
      n103 = Number To Decimal String(number=w269) -> (decimal integer string=w270:string)  [unwired: 1 in]
      n104 = call "mDrive Send Command.vi"("error in (no error)"=w267, "Extra"=w270, "Command"=T2."Run Current", "VISA resource name"=w272) -> ("error out"=w273:errorcluster, "VISA resource name out"=w271:refnum<visa-resource-name>)  [unwired: 3 in, 1 out]
    }
    frame #2 {
      # "Holding Current %"
      n105 = property on="R Holding Current %" class="DigNum (strict)"() -> ("Value"=w275:i32)  [unwired: 2 in, 2 out]
      n106 = Number To Decimal String(number=w275) -> (decimal integer string=w276:string)  [unwired: 1 in]
      n107 = call "mDrive Send Command.vi"("error in (no error)"=w277, "Extra"=w276, "Command"=T2."Holding Current", "VISA resource name"=w280) -> ("error out"=w278:errorcluster, "VISA resource name out"=w279:refnum<visa-resource-name>)  [unwired: 3 in, 1 out]
    }
    frame #3 {
      # "Print Velocity Ma"
      # "Velocity Max"
      n108 = property on="R Velocity SP step/sec" class="DigNum (strict)"() -> ("Value"=w287:i32)  [unwired: 2 in, 2 out]
      n109 = Number To Decimal String(number=w287) -> (decimal integer string=w286:string)  [unwired: 1 in]
      n110 = call "mDrive Send Command.vi"("error in (no error)"=w288, "Extra"=w286, "Command"=T2."Max Velocity", "VISA resource name"=w289) -> ("error out"=w284:errorcluster, "VISA resource name out"=w294:refnum<visa-resource-name>)  [unwired: 3 in, 1 out]
      n111 = call "mDrive Send Command.vi"("error in (no error)"=w284, "Extra"="VM", "Command"=T2."Print Parameter", "VISA resource name"=w294) -> ("error out"=w291:errorcluster, "read buffer"=w292:string, "VISA resource name out"=w290:refnum<visa-resource-name>)  [unwired: 3 in]
      n112 = Decimal String To Number(string=w292, offset=0) -> (number=w285:i32)  [unwired: 1 in, 1 out]
      n113 = property on="R velocity PV step/sec" class="DigNum (strict)"("Val(Sgnl)"=w285) -> ()  [unwired: 2 in, 2 out]
    }
    frame #4 {
      # "PRINT POSITION"
      n114 = call "mDrive Send Command.vi"("error in (no error)"=w300, "Extra"="P", "Command"=T2."Print Parameter", "VISA resource name"=w301) -> ("error out"=w302:errorcluster, "read buffer"=w299:string, "VISA resource name out"=w303:refnum<visa-resource-name>)  [unwired: 3 in]
      n115 = Decimal String To Number(string=w299, offset=0) -> (number=w297:i32)  [unwired: 1 in, 1 out]
    }
    frame #5 {
      w305 = 0 ("lower limit")
      w304 = 6144000 ("upper limit")
      n116 = property on="R Step SP" class="DigNum (strict)"("Val(Sgnl)"=w306) -> ()  [unwired: 2 in, 2 out]
      n117 = property on="R Step SP" class="DigNum (strict)"("Maximum"=w304) -> ()  [unwired: 2 in, 2 out]
      n118 = property on="R Step SP" class="DigNum (strict)"("Minimum"=w305) -> ()  [unwired: 2 in, 2 out]
      n119 = In Range and Coerce(upper limit=w304, x=w306, lower limit=w305) -> (In Range?=w307:bool)  [unwired: 1 out]
      n120 = property on="R in Range" class="Bool (strict)"("Val(Sgnl)"=w307) -> ()  [unwired: 2 in, 2 out]
      "R MINPOS" <- w305
      "R MAXPOS" <- w304
    }
  }
  n121 = flat-sequence {
    tunnel: w35 -> [w310]
    tunnel: w36 -> [w313]
    tunnel: [w312] -> w6
    tunnel: [w311] -> w5
    tunnel: [w319] -> w45
    tunnel: [w321] -> w44
    tunnel: w6 -> [w320]
    tunnel: w5 -> [w322]
    tunnel: w45 -> [w329]
    tunnel: [w328] -> w43
    tunnel: w44 -> [w326]
    tunnel: [w327] -> w42
    tunnel: [w339] -> w41
    tunnel: [w340] -> w40
    tunnel: w43 -> [w338]
    tunnel: w42 -> [w337]
    tunnel: w41 -> [w350]
    tunnel: w40 -> [w349]
    tunnel: [w352] -> w39
    tunnel: [w351] -> w38
    tunnel: [w346] -> w37
    tunnel: [w357] -> w15
    tunnel: [w358] -> w16
    tunnel: w39 -> [w358]
    tunnel: w38 -> [w357]
    tunnel: w37 -> [w355]
    frame #0 {
      n122 = call "mDrive Send Command.vi"("error in (no error)"=w310, "Extra"="EM=2", "Command"=T2."Send String", "VISA resource name"=w313) -> ("error out"=w311:errorcluster, "VISA resource name out"=w312:refnum<visa-resource-name>)  [unwired: 3 in, 1 out]
    }
    frame #1 {
      # "Run Current %"
      n123 = property on="Z Run Current %" class="DigNum (strict)"() -> ("Value"=w317:i32)  [unwired: 2 in, 2 out]
      n124 = Number To Decimal String(number=w317) -> (decimal integer string=w318:string)  [unwired: 1 in]
      n125 = call "mDrive Send Command.vi"("error in (no error)"=w322, "Extra"=w318, "Command"=T2."Run Current", "VISA resource name"=w320) -> ("error out"=w321:errorcluster, "VISA resource name out"=w319:refnum<visa-resource-name>)  [unwired: 3 in, 1 out]
    }
    frame #2 {
      # "Holding Current %"
      n126 = property on="Z Run Current %" class="DigNum (strict)"() -> ("Value"=w324:i32)  [unwired: 2 in, 2 out]
      n127 = Number To Decimal String(number=w324) -> (decimal integer string=w325:string)  [unwired: 1 in]
      n128 = call "mDrive Send Command.vi"("error in (no error)"=w326, "Extra"=w325, "Command"=T2."Holding Current", "VISA resource name"=w329) -> ("error out"=w327:errorcluster, "VISA resource name out"=w328:refnum<visa-resource-name>)  [unwired: 3 in, 1 out]
    }
    frame #3 {
      # "Print Velocity Ma"
      # "Velocity Max"
      n129 = property on="Z Velocity SP step/sec" class="DigNum (strict)"() -> ("Value"=w336:i32)  [unwired: 2 in, 2 out]
      n130 = Number To Decimal String(number=w336) -> (decimal integer string=w335:string)  [unwired: 1 in]
      n131 = call "mDrive Send Command.vi"("error in (no error)"=w337, "Extra"=w335, "Command"=T2."Max Velocity", "VISA resource name"=w338) -> ("error out"=w333:errorcluster, "VISA resource name out"=w343:refnum<visa-resource-name>)  [unwired: 3 in, 1 out]
      n132 = call "mDrive Send Command.vi"("error in (no error)"=w333, "Extra"="VM", "Command"=T2."Print Parameter", "VISA resource name"=w343) -> ("error out"=w340:errorcluster, "read buffer"=w341:string, "VISA resource name out"=w339:refnum<visa-resource-name>)  [unwired: 3 in]
      n133 = Decimal String To Number(string=w341, offset=0) -> (number=w334:i32)  [unwired: 1 in, 1 out]
      n134 = property on="Z  velocity PV step/sec" class="DigNum (strict)"("Val(Sgnl)"=w334) -> ()  [unwired: 2 in, 2 out]
    }
    frame #4 {
      # "PRINT POSITION"
      n135 = call "mDrive Send Command.vi"("error in (no error)"=w349, "Extra"="P", "Command"=T2."Print Parameter", "VISA resource name"=w350) -> ("error out"=w351:errorcluster, "read buffer"=w348:string, "VISA resource name out"=w352:refnum<visa-resource-name>)  [unwired: 3 in]
      n136 = Decimal String To Number(string=w348, offset=0) -> (number=w346:i32)  [unwired: 1 in, 1 out]
    }
    frame #5 {
      w353 = 0 ("lower limit")
      w354 = 2048000 ("upper limit")
      n137 = property on="Z Step SP" class="DigNum (strict)"("Val(Sgnl)"=w355) -> ()  [unwired: 2 in, 2 out]
      n138 = property on="Z Step SP" class="DigNum (strict)"("Maximum"=w354) -> ()  [unwired: 2 in, 2 out]
      n139 = property on="Z Step SP" class="DigNum (strict)"("Minimum"=w353) -> ()  [unwired: 2 in, 2 out]
      n140 = In Range and Coerce(upper limit=w354, x=w355, lower limit=w353) -> (In Range?=w356:bool)  [unwired: 1 out]
      n141 = property on="Z in Range" class="Bool (strict)"("Val(Sgnl)"=w356) -> ()  [unwired: 2 in, 2 out]
      "Z MINPOS" <- w353
      "Z MAXPOS" <- w354
    }
  }
  n142 = while {
    tunnel: w89 -> [w372]
    tunnel: w88 -> [w375]
    tunnel: [w376] -> w86
    tunnel: [w374] -> w87
    tunnel: w62 -> [w370]
    tunnel: w61 -> [w369]
    tunnel: [w368] -> w60
    tunnel: [w367] -> w59
    tunnel: w16 -> [w366]
    tunnel: w15 -> [w365]
    tunnel: [w364] -> w14
    tunnel: [w363] -> w13
    tunnel: w12 -> [w362]
    tunnel: w11 -> [w361]
    tunnel: [w360] -> w10
    tunnel: [w359] -> w9
    stop <- w371 stop-if-true
    n143 = flat-sequence {
      frame #0 {
      }
    }
    n144 = flat-sequence {
      frame #0 {
      }
    }
    n145 = flat-sequence {
      frame #0 {
      }
    }
    n146 = flat-sequence {
      frame #0 {
      }
    }
    n147 = flat-sequence {
      frame #0 {
      }
    }
    n148 = event shown="[16] \"X Scan OK\": Mouse Up" {
      selector: _ -> [_ _ _ _ _ _ _ _ _ _ _ _ _ _ _ _ _ _ _ _ _ _ _ _ _]
      dyn-events: _ -> [_ _ _ _ _ _ _ _ _ _ _ _ _ _ _ _ _ _ _ _ _ _ _ _ _]
      timeout: 200 -> [_ _ _ _ _ _ _ _ _ _ _ _ _ _ _ _ _ _ _ _ _ _ _ _ _]
      tunnel: w375 -> [w436 _ _ _ _ _ _ _ _ _ _ _ w1261 _ _ _ _ w1510 _ _ w1606 w1622 w1666 w1743 w1987]
      tunnel: [w435 _ _ _ _ _ _ _ _ _ _ _ w1267 _ _ _ _ w1508 _ _ w1606 w1620 w1668 w1732 w1985] -> w376
      tunnel: w372 -> [w433 _ _ _ _ _ _ _ _ _ _ _ w1262 _ _ _ _ w1509 _ _ w1607 w1623 w1667 w1745 w1988]
      tunnel: [w434 _ _ _ _ _ _ _ _ _ _ _ w1268 _ _ _ _ w1505 _ _ w1607 w1621 w1669 w1733 w1986] -> w374
      tunnel: [_ _ _ _ _ _ _ _ _ _ _ _ _ _ _ _ _ _ _ _ TRUE _ _ _ _] -> w371
      tunnel: w370 -> [w410 _ _ _ _ _ _ _ _ _ _ _ _ _ _ w1419 w1474 _ _ _ _ w1617 w1659 w1749 w1984]
      tunnel: w369 -> [w409 _ _ _ _ _ _ _ _ _ _ _ _ _ _ w1418 w1473 _ _ _ _ w1616 w1658 w1747 w1983]
      tunnel: [w408 _ _ _ _ _ _ _ _ _ _ _ _ _ _ w1417 w1472 _ _ _ _ w1619 w1657 w1725 w1982] -> w368
      tunnel: [w407 _ _ _ _ _ _ _ _ _ _ _ _ _ _ w1416 w1471 _ _ _ _ w1618 w1656 w1723 w1981] -> w367
      tunnel: w366 -> [w381 _ _ _ _ _ _ _ _ _ _ _ _ w1313 _ _ _ _ w1540 _ _ w1615 w1653 w1741 w1980]
      tunnel: w365 -> [w384 _ _ _ _ _ _ _ _ _ _ _ _ w1312 _ _ _ _ w1539 _ _ w1614 w1652 w1739 w1979]
      tunnel: [w383 _ _ _ _ _ _ _ _ _ _ _ _ w1310 _ _ _ _ w1537 _ _ w1613 w1651 w1731 w1976] -> w364
      tunnel: [w382 _ _ _ _ _ _ _ _ _ _ _ _ w1311 _ _ _ _ w1538 _ _ w1612 w1650 w1730 w1975] -> w363
      tunnel: w362 -> [w380 _ _ _ _ _ _ _ _ _ _ _ _ _ w1366 _ _ _ _ w1574 _ w1611 w1647 w1736 w1978]
      tunnel: w361 -> [w379 _ _ _ _ _ _ _ _ _ _ _ _ _ w1365 _ _ _ _ w1573 _ w1610 w1646 w1734 w1977]
      tunnel: [w378 _ _ _ _ _ _ _ _ _ _ _ _ _ w1363 _ _ _ _ w1572 _ w1609 w1645 w1728 w1974] -> w360
      tunnel: [w377 _ _ _ _ _ _ _ _ _ _ _ _ _ w1364 _ _ _ _ w1571 _ w1608 w1644 w1727 w1973] -> w359
      event #0 {
        n149 = event-data() -> ()  [unwired: 1 in, 2 out]
        n150 = flat-sequence {
          tunnel: [w726] -> w421
          tunnel: [w702] -> w420
          tunnel: [w715] -> w419
          tunnel: [w693] -> w418
          tunnel: w410 -> [w692]
          tunnel: w409 -> [w691]
          tunnel: w421 -> [w732]
          tunnel: [w732] -> w417
          tunnel: w420 -> [w731]
          tunnel: [w731] -> w416
          tunnel: w419 -> [w730]
          tunnel: [w730] -> w415
          tunnel: w418 -> [w727]
          tunnel: [w727] -> w414
          tunnel: w417 -> [w739]
          tunnel: [w740] -> w413
          tunnel: w416 -> [w742]
          tunnel: [w741] -> w412
          tunnel: w415 -> [w738]
          tunnel: [w737] -> w411
          tunnel: w414 -> [w737]
          tunnel: w413 -> [w752]
          tunnel: w412 -> [w753]
          tunnel: w411 -> [w755]
          tunnel: [w751] -> w407
          tunnel: [w750] -> w408
          frame #0 {
            w697 = 0.05 ("Delay Time (s)")
            n151 = property on="X Step SP" class="DigNum (strict)"() -> ("Maximum"=w717:dbl)  [unwired: 2 in, 2 out]
            n152 = property on="X Step SP" class="DigNum (strict)"() -> ("Minimum"=w719:dbl)  [unwired: 2 in, 2 out]
            n153 = property on="X steps/rev" class="DigNum (strict)"() -> ("Value"=w713:u32)  [unwired: 2 in, 2 out]
            n154 = property on="X offset mm" class="DigNum (strict)"() -> ("Value"=w709:dbl)  [unwired: 2 in, 2 out]
            n155 = To Long Integer(number=w717) -> (32bit integer=w716:i32)
            n156 = To Long Integer(number=w719) -> (32bit integer=w718:i32)
            n157 = To Double Precision Float(number=w713) -> (double precision float=w714:dbl)
            n158 = call "mDrive Send Command.vi"("error in (no error)"=w691, "Extra"="P", "Command"=T2."Print Parameter", "VISA resource name"=w692) -> ("error out"=w721:errorcluster, "read buffer"=w725:string, "VISA resource name out"=w723:refnum<visa-resource-name>)  [unwired: 3 in]
            n159 = call "Time Delay12"("error in (no error)"=w721, "Delay Time (s)"=w697) -> ("error out"=w720:errorcluster)  [unwired: 9 in]
            n160 = Decimal String To Number(string=w725, offset=0) -> (number=w705:i32)  [unwired: 1 in, 1 out]
            n161 = To Long Integer(number=w705) -> (32bit integer=w707:i32)
            n162 = property on="X Step PV" class="DigNum (strict)"("Val(Sgnl)"=w707) -> ()  [unwired: 2 in, 2 out]
            n163 = call "mDrive Send Command.vi"("error in (no error)"=w720, "Extra"="MV", "Command"=T2."Print Parameter", "VISA resource name"=w723) -> ("error out"=w722:errorcluster, "read buffer"=w703:string, "VISA resource name out"=w726:refnum<visa-resource-name>)  [unwired: 3 in]
            n164 = call "Time Delay11"("error in (no error)"=w722, "Delay Time (s)"=w697) -> ("error out"=w702:errorcluster)  [unwired: 9 in]
            n165 = In Range and Coerce(upper limit=w716, x=w707, lower limit=w718) -> (In Range?=w715:bool)  [unwired: 1 out]
            n166 = To Double Precision Float(number=w707) -> (double precision float=w708:dbl)
            n167 = Decimal String To Number(string=w703, offset=0 ("offset (0)")) -> (number=w696:i32)  [unwired: 1 in, 1 out]
            n168 = property on="X  in Range" class="Bool (strict)"("Val(Sgnl)"=w715) -> ()  [unwired: 2 in, 2 out]
            n169 = Divide(x=w708, y=w714) -> (x/y=w712:dbl)
            n170 = Number To Boolean Array(number=w696) -> (Boolean array=w695:bool[])
            n171 = property on="X mm/rev" class="DigNum (strict)"() -> ("Value"=w711:dbl)  [unwired: 2 in, 2 out]
            n172 = Index Array(array=w695, index=0) -> (element=w693:bool)
            n173 = property on="X  in Motion" class="Bool (strict)"("Val(Sgnl)"=w693) -> ()  [unwired: 2 in, 2 out]
            n174 = Multiply(x=w712, y=w711) -> (x*y=w710:dbl)
            n175 = Add(x=w710, y=w709) -> (x+y=w706:dbl)
            n176 = property on="X Position mm PV" class="DigNum (strict)"("Val(Sgnl)"=w706) -> ()  [unwired: 2 in, 2 out]
          }
          frame #1 {
            n177 = property on="X Scan" class="Bool (strict)"() -> ("Value"=w728:bool)  [unwired: 2 in, 2 out]
            n178 = Or(x=w727, y=w728) -> (x .or. y?=w729:bool)
            n179 = case shown="True" w729 {
              frame #0 {
                n180 = property on="X Go" class="Bool"("DisabledEnum"=T1."Enabled" ("Disabled")) -> ()  [unwired: 2 in, 2 out]
                n181 = property on="X Scan OK" class="Bool"("DisabledEnum"=T1."Enabled" ("Disabled")) -> ()  [unwired: 2 in, 2 out]
              }
              frame #1 {
                n182 = property on="X Go" class="Bool"("DisabledEnum"=T1."Disabled and Grayed Out" ("Disabled")) -> ()  [unwired: 2 in, 2 out]
                n183 = property on="X Scan OK" class="Bool"("DisabledEnum"=T1."Disabled and Grayed Out" ("Disabled")) -> ()  [unwired: 2 in, 2 out]
              }
            }
          }
          frame #2 {
            n184 = case shown="False" w738 {
              tunnel: w739 -> [w745 w749]
              tunnel: [w746 w749] -> w740
              tunnel: [w747 w748] -> w741
              tunnel: w742 -> [w744 w748]
              frame #0 {
                n185 = call "mDrive Send Command.vi"("error in (no error)"=w744, "Command"=T2."Stop", "VISA resource name"=w745) -> ("error out"=w747:errorcluster, "VISA resource name out"=w746:refnum<visa-resource-name>)  [unwired: 4 in, 1 out]
              }
              frame #1 {
              }
            }
          }
          frame #3 {
            n186 = property on="X Backlash corr" class="Bool (strict)"() -> ("Value"=w756:bool)  [unwired: 2 in, 2 out]
            n187 = Implies(1:w755, 2:w756) -> (0:w754:bool)
            n188 = case shown="False" w754 {
              tunnel: w753 -> [w763 w816]
              tunnel: w752 -> [w762 w817]
              tunnel: [w761 w816] -> w751
              tunnel: [w760 w817] -> w750
              frame #0 {
                # "Backlash"
                n189 = flat-sequence {
                  tunnel: [w778] -> w775
                  tunnel: [w780] -> w774
                  tunnel: [w779] -> w773
                  tunnel: w763 -> [w777]
                  tunnel: w762 -> [w776]
                  tunnel: w775 -> [w788]
                  tunnel: [w788] -> w772
                  tunnel: w774 -> [w787]
                  tunnel: w773 -> [w786]
                  tunnel: [w785] -> w771
                  tunnel: [w784] -> w770
                  tunnel: [w783] -> w759
                  tunnel: w772 -> [w798]
                  tunnel: w771 -> [w797]
                  tunnel: w770 -> [w795]
                  tunnel: [w796] -> w769
                  tunnel: [w795] -> w768
                  tunnel: [w794] -> w765
                  tunnel: [w793] -> w764
                  tunnel: w759 -> [w793]
                  tunnel: w769 -> [w809]
                  tunnel: w768 -> [w802]
                  tunnel: [w809] -> w767
                  tunnel: [w808] -> w766
                  tunnel: w765 -> [w808]
                  tunnel: w764 -> [w804]
                  tunnel: [w803] -> w757
                  tunnel: w767 -> [w813]
                  tunnel: w766 -> [w812]
                  tunnel: [w811] -> w761
                  tunnel: [w810] -> w758
                  tunnel: w757 -> [w810]
                  tunnel: [w815] -> w760
                  tunnel: w758 -> [w815]
                  frame #0 {
                    n190 = property on="X Backlash steps/sec" class="DigNum (strict)"() -> ("Value"=w778:i32)  [unwired: 2 in, 2 out]
                    n191 = Number To Decimal String(number=w778) -> (decimal integer string=w781:string)  [unwired: 1 in]
                    n192 = call "mDrive Send Command.vi"("error in (no error)"=w777, "Extra"=w781, "Command"=T2."Max Velocity", "VISA resource name"=w776) -> ("error out"=w779:errorcluster, "VISA resource name out"=w780:refnum<visa-resource-name>)  [unwired: 3 in, 1 out]
                  }
                  frame #1 {
                    n193 = property on="X Backlash" class="DigNum (strict)"() -> ("Value"=w783:i32)  [unwired: 2 in, 2 out]
                    n194 = Number To Decimal String(number=w783) -> (decimal integer string=w789:string)  [unwired: 1 in]
                    n195 = call "mDrive Send Command.vi"("error in (no error)"=w786, "Extra"=w789, "Command"=T2."Move to Relative Position", "VISA resource name"=w787) -> ("error out"=w785:errorcluster, "VISA resource name out"=w784:refnum<visa-resource-name>)  [unwired: 3 in, 1 out]
                  }
                  frame #2 {
                    n196 = To Double Precision Float(number=w793) -> (double precision float=w791:dbl)
                    n197 = To Double Precision Float(number=w798) -> (double precision float=w800:dbl)
                    n198 = Absolute Value(x=w791) -> (abs(x)=w792:dbl)
                    n199 = Divide(x=w792, y=w800) -> (x/y=w801:dbl)
                    n200 = Add(x=w801, y=0.3) -> (x+y=w794:dbl)
                    n201 = call "Time Delay13"("error in (no error)"=w797, "Delay Time (s)"=w794) -> ("error out"=w796:errorcluster)  [unwired: 9 in]
                  }
                  frame #3 {
                    n202 = Negate(x=w804) -> (-x=w805:i32)
                    n203 = Number To Decimal String(number=w805) -> (decimal integer string=w806:string)  [unwired: 1 in]
                    n204 = call "mDrive Send Command.vi"("Extra"=w806, "Command"=T2."Move to Relative Position", "VISA resource name"=w802) -> ("VISA resource name out"=w803:refnum<visa-resource-name>)  [unwired: 4 in, 2 out]
                  }
                  frame #4 {
                    n205 = call "Time Delay14"("error in (no error)"=w813, "Delay Time (s)"=w812) -> ("error out"=w811:errorcluster)  [unwired: 9 in]
                  }
                  frame #5 {
                    n206 = property on="X Backlash corr" class="Bool (strict)"("Val(Sgnl)"=FALSE ("Value (Signaling)")) -> ()  [unwired: 2 in, 2 out]
                  }
                }
              }
              frame #1 {
              }
            }
          }
        }
        n207 = flat-sequence {
          tunnel: w436 -> [w848]
          tunnel: w433 -> [w847]
          tunnel: [w853] -> w432
          tunnel: [w827] -> w430
          tunnel: [w840] -> w428
          tunnel: [w818] -> w426
          tunnel: w432 -> [w859]
          tunnel: [w859] -> w431
          tunnel: w430 -> [w858]
          tunnel: [w858] -> w429
          tunnel: w428 -> [w857]
          tunnel: [w857] -> w427
          tunnel: w426 -> [w854]
          tunnel: [w854] -> w422
          tunnel: w431 -> [w866]
          tunnel: [w867] -> w425
          tunnel: w429 -> [w869]
          tunnel: [w868] -> w424
          tunnel: w427 -> [w865]
          tunnel: [w864] -> w423
          tunnel: w422 -> [w864]
          tunnel: w425 -> [w879]
          tunnel: w424 -> [w880]
          tunnel: w423 -> [w882]
          tunnel: [w878] -> w435
          tunnel: [w877] -> w434
          frame #0 {
            w822 = 0.05 ("Delay Time (s)")
            n208 = property on="Y Step SP" class="DigNum (strict)"() -> ("Maximum"=w842:dbl)  [unwired: 2 in, 2 out]
            n209 = property on="Y Step SP" class="DigNum (strict)"() -> ("Minimum"=w844:dbl)  [unwired: 2 in, 2 out]
            n210 = property on="Y steps/rev" class="DigNum (strict)"() -> ("Value"=w838:u32)  [unwired: 2 in, 2 out]
            n211 = property on="Y offset mm" class="DigNum (strict)"() -> ("Value"=w834:dbl)  [unwired: 2 in, 2 out]
            n212 = To Long Integer(number=w842) -> (32bit integer=w841:i32)
            n213 = To Long Integer(number=w844) -> (32bit integer=w843:i32)
            n214 = To Double Precision Float(number=w838) -> (double precision float=w839:dbl)
            n215 = call "mDrive Send Command.vi"("error in (no error)"=w848, "Extra"="P", "Command"=T2."Print Parameter", "VISA resource name"=w847) -> ("error out"=w846:errorcluster, "read buffer"=w852:string, "VISA resource name out"=w850:refnum<visa-resource-name>)  [unwired: 3 in]
            n216 = call "Time Delay4"("error in (no error)"=w846, "Delay Time (s)"=w822) -> ("error out"=w845:errorcluster)  [unwired: 9 in]
            n217 = Decimal String To Number(string=w852, offset=0) -> (number=w830:i32)  [unwired: 1 in, 1 out]
            n218 = To Long Integer(number=w830) -> (32bit integer=w832:i32)
            n219 = property on="Y Step PV" class="DigNum (strict)"("Val(Sgnl)"=w832) -> ()  [unwired: 2 in, 2 out]
            n220 = call "mDrive Send Command.vi"("error in (no error)"=w845, "Extra"="MV", "Command"=T2."Print Parameter", "VISA resource name"=w850) -> ("error out"=w849:errorcluster, "read buffer"=w828:string, "VISA resource name out"=w853:refnum<visa-resource-name>)  [unwired: 3 in]
            n221 = call "Time Delay3"("error in (no error)"=w849, "Delay Time (s)"=w822) -> ("error out"=w827:errorcluster)  [unwired: 9 in]
            n222 = In Range and Coerce(upper limit=w841, x=w832, lower limit=w843) -> (In Range?=w840:bool)  [unwired: 1 out]
            n223 = To Double Precision Float(number=w832) -> (double precision float=w833:dbl)
            n224 = Decimal String To Number(string=w828, offset=0 ("offset (0)")) -> (number=w821:i32)  [unwired: 1 in, 1 out]
            n225 = property on="Y in Range" class="Bool (strict)"("Val(Sgnl)"=w840) -> ()  [unwired: 2 in, 2 out]
            n226 = Divide(x=w833, y=w839) -> (x/y=w837:dbl)
            n227 = Number To Boolean Array(number=w821) -> (Boolean array=w820:bool[])
            n228 = property on="Y mm/rev" class="DigNum (strict)"() -> ("Value"=w836:dbl)  [unwired: 2 in, 2 out]
            n229 = Index Array(array=w820, index=0) -> (element=w818:bool)
            n230 = property on="Y in Motion" class="Bool (strict)"("Val(Sgnl)"=w818) -> ()  [unwired: 2 in, 2 out]
            n231 = Multiply(x=w837, y=w836) -> (x*y=w835:dbl)
            n232 = Add(x=w835, y=w834) -> (x+y=w831:dbl)
            n233 = property on="Y Position mm PV" class="DigNum (strict)"("Val(Sgnl)"=w831) -> ()  [unwired: 2 in, 2 out]
          }
          frame #1 {
            n234 = property on="Y Scan" class="Bool (strict)"() -> ("Value"=w855:bool)  [unwired: 2 in, 2 out]
            n235 = Or(x=w854, y=w855) -> (x .or. y?=w856:bool)
            n236 = case shown="True" w856 {
              frame #0 {
                n237 = property on="Y Go" class="Bool"("DisabledEnum"=T1."Enabled" ("Disabled")) -> ()  [unwired: 2 in, 2 out]
                n238 = property on="Y Scan OK" class="Bool"("DisabledEnum"=T1."Enabled" ("Disabled")) -> ()  [unwired: 2 in, 2 out]
              }
              frame #1 {
                n239 = property on="Y Go" class="Bool"("DisabledEnum"=T1."Disabled and Grayed Out" ("Disabled")) -> ()  [unwired: 2 in, 2 out]
                n240 = property on="Y Scan OK" class="Bool"("DisabledEnum"=T1."Disabled and Grayed Out" ("Disabled")) -> ()  [unwired: 2 in, 2 out]
              }
            }
          }
          frame #2 {
            n241 = case shown="False" w865 {
              tunnel: w866 -> [w872 w876]
              tunnel: [w873 w876] -> w867
              tunnel: [w874 w875] -> w868
              tunnel: w869 -> [w871 w875]
              frame #0 {
                n242 = call "mDrive Send Command.vi"("error in (no error)"=w871, "Command"=T2."Stop", "VISA resource name"=w872) -> ("error out"=w874:errorcluster, "VISA resource name out"=w873:refnum<visa-resource-name>)  [unwired: 4 in, 1 out]
              }
              frame #1 {
              }
            }
          }
          frame #3 {
            n243 = property on="Y Backlash corr" class="Bool (strict)"() -> ("Value"=w883:bool)  [unwired: 2 in, 2 out]
            n244 = Implies(1:w882, 2:w883) -> (0:w881:bool)
            n245 = case shown="False" w881 {
              tunnel: w880 -> [w890 w943]
              tunnel: w879 -> [w889 w944]
              tunnel: [w888 w943] -> w878
              tunnel: [w887 w944] -> w877
              frame #0 {
                # "Backlash"
                n246 = flat-sequence {
                  tunnel: [w905] -> w902
                  tunnel: [w907] -> w901
                  tunnel: [w906] -> w900
                  tunnel: w890 -> [w904]
                  tunnel: w889 -> [w903]
                  tunnel: w902 -> [w915]
                  tunnel: [w915] -> w899
                  tunnel: w901 -> [w914]
                  tunnel: w900 -> [w913]
                  tunnel: [w912] -> w898
                  tunnel: [w911] -> w897
                  tunnel: [w910] -> w886
                  tunnel: w899 -> [w925]
                  tunnel: w898 -> [w924]
                  tunnel: w897 -> [w922]
                  tunnel: [w923] -> w896
                  tunnel: [w922] -> w895
                  tunnel: [w921] -> w892
                  tunnel: [w920] -> w891
                  tunnel: w886 -> [w920]
                  tunnel: w896 -> [w936]
                  tunnel: w895 -> [w929]
                  tunnel: [w936] -> w894
                  tunnel: [w935] -> w893
                  tunnel: w892 -> [w935]
                  tunnel: w891 -> [w931]
                  tunnel: [w930] -> w884
                  tunnel: w894 -> [w940]
                  tunnel: w893 -> [w939]
                  tunnel: [w938] -> w888
                  tunnel: [w937] -> w885
                  tunnel: w884 -> [w937]
                  tunnel: [w942] -> w887
                  tunnel: w885 -> [w942]
                  frame #0 {
                    n247 = property on="Y Backlash steps/sec" class="DigNum (strict)"() -> ("Value"=w905:i32)  [unwired: 2 in, 2 out]
                    n248 = Number To Decimal String(number=w905) -> (decimal integer string=w908:string)  [unwired: 1 in]
                    n249 = call "mDrive Send Command.vi"("error in (no error)"=w904, "Extra"=w908, "Command"=T2."Max Velocity", "VISA resource name"=w903) -> ("error out"=w906:errorcluster, "VISA resource name out"=w907:refnum<visa-resource-name>)  [unwired: 3 in, 1 out]
                  }
                  frame #1 {
                    n250 = property on="Y Backlash" class="DigNum (strict)"() -> ("Value"=w910:i32)  [unwired: 2 in, 2 out]
                    n251 = Number To Decimal String(number=w910) -> (decimal integer string=w916:string)  [unwired: 1 in]
                    n252 = call "mDrive Send Command.vi"("error in (no error)"=w913, "Extra"=w916, "Command"=T2."Move to Relative Position", "VISA resource name"=w914) -> ("error out"=w912:errorcluster, "VISA resource name out"=w911:refnum<visa-resource-name>)  [unwired: 3 in, 1 out]
                  }
                  frame #2 {
                    n253 = To Double Precision Float(number=w920) -> (double precision float=w918:dbl)
                    n254 = To Double Precision Float(number=w925) -> (double precision float=w927:dbl)
                    n255 = Absolute Value(x=w918) -> (abs(x)=w919:dbl)
                    n256 = Divide(x=w919, y=w927) -> (x/y=w928:dbl)
                    n257 = Add(x=w928, y=0.3) -> (x+y=w921:dbl)
                    n258 = call "Time Delay8"("error in (no error)"=w924, "Delay Time (s)"=w921) -> ("error out"=w923:errorcluster)  [unwired: 9 in]
                  }
                  frame #3 {
                    n259 = Negate(x=w931) -> (-x=w932:i32)
                    n260 = Number To Decimal String(number=w932) -> (decimal integer string=w933:string)  [unwired: 1 in]
                    n261 = call "mDrive Send Command.vi"("Extra"=w933, "Command"=T2."Move to Relative Position", "VISA resource name"=w929) -> ("VISA resource name out"=w930:refnum<visa-resource-name>)  [unwired: 4 in, 2 out]
                  }
                  frame #4 {
                    n262 = call "Time Delay2"("error in (no error)"=w940, "Delay Time (s)"=w939) -> ("error out"=w938:errorcluster)  [unwired: 9 in]
                  }
                  frame #5 {
                    n263 = property on="Y Backlash corr" class="Bool (strict)"("Val(Sgnl)"=FALSE ("Value (Signaling)")) -> ()  [unwired: 2 in, 2 out]
                  }
                }
              }
              frame #1 {
              }
            }
          }
        }
        n264 = flat-sequence {
          tunnel: [w599] -> w406
          tunnel: [w575] -> w405
          tunnel: [w588] -> w404
          tunnel: [w566] -> w403
          tunnel: w381 -> [w565]
          tunnel: w384 -> [w564]
          tunnel: w406 -> [w605]
          tunnel: [w605] -> w402
          tunnel: w405 -> [w604]
          tunnel: [w604] -> w401
          tunnel: w404 -> [w603]
          tunnel: [w603] -> w400
          tunnel: w403 -> [w600]
          tunnel: [w600] -> w399
          tunnel: w402 -> [w612]
          tunnel: [w613] -> w398
          tunnel: w401 -> [w615]
          tunnel: [w614] -> w397
          tunnel: w400 -> [w611]
          tunnel: [w610] -> w396
          tunnel: w399 -> [w610]
          tunnel: w398 -> [w625]
          tunnel: w397 -> [w626]
          tunnel: w396 -> [w628]
          tunnel: [w624] -> w382
          tunnel: [w623] -> w383
          frame #0 {
            w570 = 0.05 ("Delay Time (s)")
            n265 = property on="Z Step SP" class="DigNum (strict)"() -> ("Maximum"=w590:dbl)  [unwired: 2 in, 2 out]
            n266 = property on="Z Step SP" class="DigNum (strict)"() -> ("Minimum"=w592:dbl)  [unwired: 2 in, 2 out]
            n267 = property on="Z steps/rev" class="DigNum (strict)"() -> ("Value"=w586:u32)  [unwired: 2 in, 2 out]
            n268 = property on="Z offset mm" class="DigNum (strict)"() -> ("Value"=w582:dbl)  [unwired: 2 in, 2 out]
            n269 = To Long Integer(number=w590) -> (32bit integer=w589:i32)
            n270 = To Long Integer(number=w592) -> (32bit integer=w591:i32)
            n271 = To Double Precision Float(number=w586) -> (double precision float=w587:dbl)
            n272 = call "mDrive Send Command.vi"("error in (no error)"=w564, "Extra"="P", "Command"=T2."Print Parameter", "VISA resource name"=w565) -> ("error out"=w594:errorcluster, "read buffer"=w598:string, "VISA resource name out"=w596:refnum<visa-resource-name>)  [unwired: 3 in]
            n273 = call "Time Delay17"("error in (no error)"=w594, "Delay Time (s)"=w570) -> ("error out"=w593:errorcluster)  [unwired: 9 in]
            n274 = Decimal String To Number(string=w598, offset=0) -> (number=w578:i32)  [unwired: 1 in, 1 out]
            n275 = To Long Integer(number=w578) -> (32bit integer=w580:i32)
            n276 = property on="Z Step PV" class="DigNum (strict)"("Val(Sgnl)"=w580) -> ()  [unwired: 2 in, 2 out]
            n277 = call "mDrive Send Command.vi"("error in (no error)"=w593, "Extra"="MV", "Command"=T2."Print Parameter", "VISA resource name"=w596) -> ("error out"=w595:errorcluster, "read buffer"=w576:string, "VISA resource name out"=w599:refnum<visa-resource-name>)  [unwired: 3 in]
            n278 = call "Time Delay16"("error in (no error)"=w595, "Delay Time (s)"=w570) -> ("error out"=w575:errorcluster)  [unwired: 9 in]
            n279 = In Range and Coerce(upper limit=w589, x=w580, lower limit=w591) -> (In Range?=w588:bool)  [unwired: 1 out]
            n280 = To Double Precision Float(number=w580) -> (double precision float=w581:dbl)
            n281 = Decimal String To Number(string=w576, offset=0 ("offset (0)")) -> (number=w569:i32)  [unwired: 1 in, 1 out]
            n282 = property on="Z in Range" class="Bool (strict)"("Val(Sgnl)"=w588) -> ()  [unwired: 2 in, 2 out]
            n283 = Divide(x=w581, y=w587) -> (x/y=w585:dbl)
            n284 = Number To Boolean Array(number=w569) -> (Boolean array=w568:bool[])
            n285 = property on="Z mm/rev" class="DigNum (strict)"() -> ("Value"=w584:dbl)  [unwired: 2 in, 2 out]
            n286 = Index Array(array=w568, index=0) -> (element=w566:bool)
            n287 = property on="Z in Motion" class="Bool (strict)"("Val(Sgnl)"=w566) -> ()  [unwired: 2 in, 2 out]
            n288 = Multiply(x=w585, y=w584) -> (x*y=w583:dbl)
            n289 = Add(x=w583, y=w582) -> (x+y=w579:dbl)
            n290 = property on="Z Position mm PV" class="DigNum (strict)"("Val(Sgnl)"=w579) -> ()  [unwired: 2 in, 2 out]
          }
          frame #1 {
            n291 = property on="Z Scan" class="Bool (strict)"() -> ("Value"=w601:bool)  [unwired: 2 in, 2 out]
            n292 = Or(x=w600, y=w601) -> (x .or. y?=w602:bool)
            n293 = case shown="True" w602 {
              frame #0 {
                n294 = property on="Z Go" class="Bool"("DisabledEnum"=T1."Enabled" ("Disabled")) -> ()  [unwired: 2 in, 2 out]
                n295 = property on="Z Scan OK" class="Bool"("DisabledEnum"=T1."Enabled" ("Disabled")) -> ()  [unwired: 2 in, 2 out]
              }
              frame #1 {
                n296 = property on="Z Go" class="Bool"("DisabledEnum"=T1."Disabled and Grayed Out" ("Disabled")) -> ()  [unwired: 2 in, 2 out]
                n297 = property on="Z Scan OK" class="Bool"("DisabledEnum"=T1."Disabled and Grayed Out" ("Disabled")) -> ()  [unwired: 2 in, 2 out]
              }
            }
          }
          frame #2 {
            n298 = case shown="False" w611 {
              tunnel: w612 -> [w618 w622]
              tunnel: [w619 w622] -> w613
              tunnel: [w620 w621] -> w614
              tunnel: w615 -> [w617 w621]
              frame #0 {
                n299 = call "mDrive Send Command.vi"("error in (no error)"=w617, "Command"=T2."Stop", "VISA resource name"=w618) -> ("error out"=w620:errorcluster, "VISA resource name out"=w619:refnum<visa-resource-name>)  [unwired: 4 in, 1 out]
              }
              frame #1 {
              }
            }
          }
          frame #3 {
            n300 = property on="Z Backlash corr" class="Bool (strict)"() -> ("Value"=w629:bool)  [unwired: 2 in, 2 out]
            n301 = Implies(1:w628, 2:w629) -> (0:w627:bool)
            n302 = case shown="False" w627 {
              tunnel: w626 -> [w636 w689]
              tunnel: w625 -> [w635 w690]
              tunnel: [w634 w689] -> w624
              tunnel: [w633 w690] -> w623
              frame #0 {
                # "Backlash"
                n303 = flat-sequence {
                  tunnel: [w651] -> w648
                  tunnel: [w653] -> w647
                  tunnel: [w652] -> w646
                  tunnel: w636 -> [w650]
                  tunnel: w635 -> [w649]
                  tunnel: w648 -> [w661]
                  tunnel: [w661] -> w645
                  tunnel: w647 -> [w660]
                  tunnel: w646 -> [w659]
                  tunnel: [w658] -> w644
                  tunnel: [w657] -> w643
                  tunnel: [w656] -> w632
                  tunnel: w645 -> [w671]
                  tunnel: w644 -> [w670]
                  tunnel: w643 -> [w668]
                  tunnel: [w669] -> w642
                  tunnel: [w668] -> w641
                  tunnel: [w667] -> w638
                  tunnel: [w666] -> w637
                  tunnel: w632 -> [w666]
                  tunnel: w642 -> [w682]
                  tunnel: w641 -> [w675]
                  tunnel: [w682] -> w640
                  tunnel: [w681] -> w639
                  tunnel: w638 -> [w681]
                  tunnel: w637 -> [w677]
                  tunnel: [w676] -> w630
                  tunnel: w640 -> [w686]
                  tunnel: w639 -> [w685]
                  tunnel: [w684] -> w634
                  tunnel: [w683] -> w631
                  tunnel: w630 -> [w683]
                  tunnel: [w688] -> w633
                  tunnel: w631 -> [w688]
                  frame #0 {
                    n304 = property on="Z Backlash steps/sec" class="DigNum (strict)"() -> ("Value"=w651:i32)  [unwired: 2 in, 2 out]
                    n305 = Number To Decimal String(number=w651) -> (decimal integer string=w654:string)  [unwired: 1 in]
                    n306 = call "mDrive Send Command.vi"("error in (no error)"=w650, "Extra"=w654, "Command"=T2."Max Velocity", "VISA resource name"=w649) -> ("error out"=w652:errorcluster, "VISA resource name out"=w653:refnum<visa-resource-name>)  [unwired: 3 in, 1 out]
                  }
                  frame #1 {
                    n307 = property on="Z Backlash" class="DigNum (strict)"() -> ("Value"=w656:i32)  [unwired: 2 in, 2 out]
                    n308 = Number To Decimal String(number=w656) -> (decimal integer string=w662:string)  [unwired: 1 in]
                    n309 = call "mDrive Send Command.vi"("error in (no error)"=w659, "Extra"=w662, "Command"=T2."Move to Relative Position", "VISA resource name"=w660) -> ("error out"=w658:errorcluster, "VISA resource name out"=w657:refnum<visa-resource-name>)  [unwired: 3 in, 1 out]
                  }
                  frame #2 {
                    n310 = To Double Precision Float(number=w666) -> (double precision float=w664:dbl)
                    n311 = To Double Precision Float(number=w671) -> (double precision float=w673:dbl)
                    n312 = Absolute Value(x=w664) -> (abs(x)=w665:dbl)
                    n313 = Divide(x=w665, y=w673) -> (x/y=w674:dbl)
                    n314 = Add(x=w674, y=0.3) -> (x+y=w667:dbl)
                    n315 = call "Time Delay18"("error in (no error)"=w670, "Delay Time (s)"=w667) -> ("error out"=w669:errorcluster)  [unwired: 9 in]
                  }
                  frame #3 {
                    n316 = Negate(x=w677) -> (-x=w678:i32)
                    n317 = Number To Decimal String(number=w678) -> (decimal integer string=w679:string)  [unwired: 1 in]
                    n318 = call "mDrive Send Command.vi"("Extra"=w679, "Command"=T2."Move to Relative Position", "VISA resource name"=w675) -> ("VISA resource name out"=w676:refnum<visa-resource-name>)  [unwired: 4 in, 2 out]
                  }
                  frame #4 {
                    n319 = call "Time Delay19"("error in (no error)"=w686, "Delay Time (s)"=w685) -> ("error out"=w684:errorcluster)  [unwired: 9 in]
                  }
                  frame #5 {
                    n320 = property on="Z Backlash corr" class="Bool (strict)"("Val(Sgnl)"=FALSE ("Value (Signaling)")) -> ()  [unwired: 2 in, 2 out]
                  }
                }
              }
              frame #1 {
              }
            }
          }
        }
        n321 = flat-sequence {
          tunnel: [w472] -> w395
          tunnel: [w448] -> w394
          tunnel: [w461] -> w393
          tunnel: [w439] -> w392
          tunnel: w380 -> [w438]
          tunnel: w379 -> [w437]
          tunnel: w395 -> [w478]
          tunnel: [w478] -> w391
          tunnel: w394 -> [w477]
          tunnel: [w477] -> w390
          tunnel: w393 -> [w476]
          tunnel: [w476] -> w389
          tunnel: w392 -> [w473]
          tunnel: [w473] -> w388
          tunnel: w391 -> [w485]
          tunnel: [w486] -> w387
          tunnel: w390 -> [w488]
          tunnel: [w487] -> w386
          tunnel: w389 -> [w484]
          tunnel: [w483] -> w385
          tunnel: w388 -> [w483]
          tunnel: w387 -> [w498]
          tunnel: w386 -> [w499]
          tunnel: w385 -> [w501]
          tunnel: [w497] -> w377
          tunnel: [w496] -> w378
          frame #0 {
            w443 = 0.05 ("Delay Time (s)")
            n322 = property on="R Step SP" class="DigNum (strict)"() -> ("Maximum"=w463:dbl)  [unwired: 2 in, 2 out]
            n323 = property on="R Step SP" class="DigNum (strict)"() -> ("Minimum"=w465:dbl)  [unwired: 2 in, 2 out]
            n324 = property on="R steps/rev" class="DigNum (strict)"() -> ("Value"=w459:u32)  [unwired: 2 in, 2 out]
            n325 = property on="R offset deg" class="DigNum (strict)"() -> ("Value"=w455:dbl)  [unwired: 2 in, 2 out]
            n326 = To Long Integer(number=w463) -> (32bit integer=w462:i32)
            n327 = To Long Integer(number=w465) -> (32bit integer=w464:i32)
            n328 = To Double Precision Float(number=w459) -> (double precision float=w460:dbl)
            n329 = call "mDrive Send Command.vi"("error in (no error)"=w437, "Extra"="P", "Command"=T2."Print Parameter", "VISA resource name"=w438) -> ("error out"=w467:errorcluster, "read buffer"=w471:string, "VISA resource name out"=w469:refnum<visa-resource-name>)  [unwired: 3 in]
            n330 = call "Time Delay21"("error in (no error)"=w467, "Delay Time (s)"=w443) -> ("error out"=w466:errorcluster)  [unwired: 9 in]
            n331 = Decimal String To Number(string=w471, offset=0) -> (number=w451:i32)  [unwired: 1 in, 1 out]
            n332 = To Long Integer(number=w451) -> (32bit integer=w453:i32)
            n333 = property on="R Step PV" class="DigNum (strict)"("Val(Sgnl)"=w453) -> ()  [unwired: 2 in, 2 out]
            n334 = call "mDrive Send Command.vi"("error in (no error)"=w466, "Extra"="MV", "Command"=T2."Print Parameter", "VISA resource name"=w469) -> ("error out"=w468:errorcluster, "read buffer"=w449:string, "VISA resource name out"=w472:refnum<visa-resource-name>)  [unwired: 3 in]
            n335 = call "Time Delay20"("error in (no error)"=w468, "Delay Time (s)"=w443) -> ("error out"=w448:errorcluster)  [unwired: 9 in]
            n336 = In Range and Coerce(upper limit=w462, x=w453, lower limit=w464) -> (In Range?=w461:bool)  [unwired: 1 out]
            n337 = To Double Precision Float(number=w453) -> (double precision float=w454:dbl)
            n338 = Decimal String To Number(string=w449, offset=0 ("offset (0)")) -> (number=w442:i32)  [unwired: 1 in, 1 out]
            n339 = property on="R in Range" class="Bool (strict)"("Val(Sgnl)"=w461) -> ()  [unwired: 2 in, 2 out]
            n340 = Divide(x=w454, y=w460) -> (x/y=w458:dbl)
            n341 = Number To Boolean Array(number=w442) -> (Boolean array=w441:bool[])
            n342 = property on="R deg/rev" class="DigNum (strict)"() -> ("Value"=w457:dbl)  [unwired: 2 in, 2 out]
            n343 = Index Array(array=w441, index=0) -> (element=w439:bool)
            n344 = property on="R in Motion" class="Bool (strict)"("Val(Sgnl)"=w439) -> ()  [unwired: 2 in, 2 out]
            n345 = Multiply(x=w458, y=w457) -> (x*y=w456:dbl)
            n346 = Add(x=w456, y=w455) -> (x+y=w452:dbl)
            n347 = property on="R Position deg PV" class="DigNum (strict)"("Val(Sgnl)"=w452) -> ()  [unwired: 2 in, 2 out]
          }
          frame #1 {
            n348 = property on="R Scan" class="Bool (strict)"() -> ("Value"=w474:bool)  [unwired: 2 in, 2 out]
            n349 = Or(x=w473, y=w474) -> (x .or. y?=w475:bool)
            n350 = case shown="True" w475 {
              frame #0 {
                n351 = property on="R Go" class="Bool"("DisabledEnum"=T1."Enabled" ("Disabled")) -> ()  [unwired: 2 in, 2 out]
                n352 = property on="R Scan OK" class="Bool"("DisabledEnum"=T1."Enabled" ("Disabled")) -> ()  [unwired: 2 in, 2 out]
              }
              frame #1 {
                n353 = property on="R Go" class="Bool"("DisabledEnum"=T1."Disabled and Grayed Out" ("Disabled")) -> ()  [unwired: 2 in, 2 out]
                n354 = property on="R Scan OK" class="Bool"("DisabledEnum"=T1."Disabled and Grayed Out" ("Disabled")) -> ()  [unwired: 2 in, 2 out]
              }
            }
          }
          frame #2 {
            n355 = case shown="False" w484 {
              tunnel: w485 -> [w491 w495]
              tunnel: [w492 w495] -> w486
              tunnel: [w493 w494] -> w487
              tunnel: w488 -> [w490 w494]
              frame #0 {
                n356 = call "mDrive Send Command.vi"("error in (no error)"=w490, "Command"=T2."Stop", "VISA resource name"=w491) -> ("error out"=w493:errorcluster, "VISA resource name out"=w492:refnum<visa-resource-name>)  [unwired: 4 in, 1 out]
              }
              frame #1 {
              }
            }
          }
          frame #3 {
            n357 = property on="R Backlash corr" class="Bool (strict)"() -> ("Value"=w502:bool)  [unwired: 2 in, 2 out]
            n358 = Implies(1:w501, 2:w502) -> (0:w500:bool)
            n359 = case shown="False" w500 {
              tunnel: w499 -> [w509 w562]
              tunnel: w498 -> [w508 w563]
              tunnel: [w507 w562] -> w497
              tunnel: [w506 w563] -> w496
              frame #0 {
                # "Backlash"
                n360 = flat-sequence {
                  tunnel: [w524] -> w521
                  tunnel: [w526] -> w520
                  tunnel: [w525] -> w519
                  tunnel: w509 -> [w523]
                  tunnel: w508 -> [w522]
                  tunnel: w521 -> [w534]
                  tunnel: [w534] -> w518
                  tunnel: w520 -> [w533]
                  tunnel: w519 -> [w532]
                  tunnel: [w531] -> w517
                  tunnel: [w530] -> w516
                  tunnel: [w529] -> w505
                  tunnel: w518 -> [w544]
                  tunnel: w517 -> [w543]
                  tunnel: w516 -> [w541]
                  tunnel: [w542] -> w515
                  tunnel: [w541] -> w514
                  tunnel: [w540] -> w511
                  tunnel: [w539] -> w510
                  tunnel: w505 -> [w539]
                  tunnel: w515 -> [w555]
                  tunnel: w514 -> [w548]
                  tunnel: [w555] -> w513
                  tunnel: [w554] -> w512
                  tunnel: w511 -> [w554]
                  tunnel: w510 -> [w550]
                  tunnel: [w549] -> w503
                  tunnel: w513 -> [w559]
                  tunnel: w512 -> [w558]
                  tunnel: [w557] -> w507
                  tunnel: [w556] -> w504
                  tunnel: w503 -> [w556]
                  tunnel: [w561] -> w506
                  tunnel: w504 -> [w561]
                  frame #0 {
                    n361 = property on="R Backlash steps/sec" class="DigNum (strict)"() -> ("Value"=w524:i32)  [unwired: 2 in, 2 out]
                    n362 = Number To Decimal String(number=w524) -> (decimal integer string=w527:string)  [unwired: 1 in]
                    n363 = call "mDrive Send Command.vi"("error in (no error)"=w523, "Extra"=w527, "Command"=T2."Max Velocity", "VISA resource name"=w522) -> ("error out"=w525:errorcluster, "VISA resource name out"=w526:refnum<visa-resource-name>)  [unwired: 3 in, 1 out]
                  }
                  frame #1 {
                    n364 = property on="R Backlash" class="DigNum (strict)"() -> ("Value"=w529:i32)  [unwired: 2 in, 2 out]
                    n365 = Number To Decimal String(number=w529) -> (decimal integer string=w535:string)  [unwired: 1 in]
                    n366 = call "mDrive Send Command.vi"("error in (no error)"=w532, "Extra"=w535, "Command"=T2."Move to Relative Position", "VISA resource name"=w533) -> ("error out"=w531:errorcluster, "VISA resource name out"=w530:refnum<visa-resource-name>)  [unwired: 3 in, 1 out]
                  }
                  frame #2 {
                    n367 = To Double Precision Float(number=w539) -> (double precision float=w537:dbl)
                    n368 = To Double Precision Float(number=w544) -> (double precision float=w546:dbl)
                    n369 = Absolute Value(x=w537) -> (abs(x)=w538:dbl)
                    n370 = Divide(x=w538, y=w546) -> (x/y=w547:dbl)
                    n371 = Add(x=w547, y=0.3) -> (x+y=w540:dbl)
                    n372 = call "Time Delay22"("error in (no error)"=w543, "Delay Time (s)"=w540) -> ("error out"=w542:errorcluster)  [unwired: 9 in]
                  }
                  frame #3 {
                    n373 = Negate(x=w550) -> (-x=w551:i32)
                    n374 = Number To Decimal String(number=w551) -> (decimal integer string=w552:string)  [unwired: 1 in]
                    n375 = call "mDrive Send Command.vi"("Extra"=w552, "Command"=T2."Move to Relative Position", "VISA resource name"=w548) -> ("VISA resource name out"=w549:refnum<visa-resource-name>)  [unwired: 4 in, 2 out]
                  }
                  frame #4 {
                    n376 = call "Time Delay23"("error in (no error)"=w559, "Delay Time (s)"=w558) -> ("error out"=w557:errorcluster)  [unwired: 9 in]
                  }
                  frame #5 {
                    n377 = property on="R Backlash corr" class="Bool (strict)"("Val(Sgnl)"=FALSE ("Value (Signaling)")) -> ()  [unwired: 2 in, 2 out]
                  }
                }
              }
              frame #1 {
              }
            }
          }
        }
      }
      event #1 {
        n378 = event-data() -> ()  [unwired: 1 in, 5 out]
        n379 = property on="Z steps/rev" class="DigNum (strict)"() -> ("Value"=w956:u32)  [unwired: 2 in, 2 out]
        n380 = property on="X steps/rev" class="DigNum (strict)"() -> ("Value"=w965:u32)  [unwired: 2 in, 2 out]
        n381 = property on="Y steps/rev" class="DigNum (strict)"() -> ("Value"=w974:u32)  [unwired: 2 in, 2 out]
        n382 = property on="R steps/rev" class="DigNum (strict)"() -> ("Value"=w947:u32)  [unwired: 2 in, 2 out]
        n383 = property on="R offset deg" class="DigNum (strict)"() -> ("Value"=w945:dbl)  [unwired: 2 in, 2 out]
        n384 = property on="Z offset mm" class="DigNum (strict)"() -> ("Value"=w954:dbl)  [unwired: 2 in, 2 out]
        n385 = property on="X offset mm" class="DigNum (strict)"() -> ("Value"=w963:dbl)  [unwired: 2 in, 2 out]
        n386 = property on="Y offset mm" class="DigNum (strict)"() -> ("Value"=w972:dbl)  [unwired: 2 in, 2 out]
        n387 = To Double Precision Float(number=w974) -> (double precision float=w977:dbl)
        n388 = property on="Reset Z Position mm" class="DigNum (strict)"() -> ("Value"=w962:dbl)  [unwired: 2 in, 2 out]
        n389 = property on="Reset X Position mm" class="DigNum (strict)"() -> ("Value"=w971:dbl)  [unwired: 2 in, 2 out]
        n390 = property on="Reset Y Position mm" class="DigNum (strict)"() -> ("Value"=w980:dbl)  [unwired: 2 in, 2 out]
        n391 = property on="Reset R Position deg" class="DigNum (strict)"() -> ("Value"=w953:dbl)  [unwired: 2 in, 2 out]
        n392 = Subtract(x=w962, y=w954) -> (x-y=w961:dbl)
        n393 = Subtract(x=w953, y=w945) -> (x-y=w952:dbl)
        n394 = Subtract(x=w971, y=w963) -> (x-y=w970:dbl)
        n395 = Subtract(x=w980, y=w972) -> (x-y=w979:dbl)
        n396 = property on="Z mm/rev" class="DigNum (strict)"() -> ("Value"=w955:dbl)  [unwired: 2 in, 2 out]
        n397 = property on="X mm/rev" class="DigNum (strict)"() -> ("Value"=w964:dbl)  [unwired: 2 in, 2 out]
        n398 = property on="Y mm/rev" class="DigNum (strict)"() -> ("Value"=w973:dbl)  [unwired: 2 in, 2 out]
        n399 = property on="R deg/rev" class="DigNum (strict)"() -> ("Value"=w946:dbl)  [unwired: 2 in, 2 out]
        n400 = Divide(x=w979, y=w973) -> (x/y=w978:dbl)
        n401 = Divide(x=w961, y=w955) -> (x/y=w960:dbl)
        n402 = Divide(x=w952, y=w946) -> (x/y=w951:dbl)
        n403 = Divide(x=w970, y=w964) -> (x/y=w969:dbl)
        n404 = To Double Precision Float(number=w956) -> (double precision float=w959:dbl)
        n405 = To Double Precision Float(number=w947) -> (double precision float=w950:dbl)
        n406 = To Double Precision Float(number=w965) -> (double precision float=w968:dbl)
        n407 = Multiply(x=w960, y=w959) -> (x*y=w958:dbl)
        n408 = Multiply(x=w951, y=w950) -> (x*y=w949:dbl)
        n409 = Multiply(x=w969, y=w968) -> (x*y=w967:dbl)
        n410 = Multiply(x=w978, y=w977) -> (x*y=w976:dbl)
        n411 = To Long Integer(number=w958) -> (32bit integer=w957:i32)
        n412 = To Long Integer(number=w949) -> (32bit integer=w948:i32)
        n413 = To Long Integer(number=w967) -> (32bit integer=w966:i32)
        n414 = To Long Integer(number=w976) -> (32bit integer=w975:i32)
        n415 = property on="Reset Z Motor Steps" class="DigNum (strict)"("Val(Sgnl)"=w957) -> ()  [unwired: 2 in, 2 out]
        n416 = property on="Reset R Motor Steps" class="DigNum (strict)"("Val(Sgnl)"=w948) -> ()  [unwired: 2 in, 2 out]
        n417 = property on="Reset X Motor Steps" class="DigNum (strict)"("Val(Sgnl)"=w966) -> ()  [unwired: 2 in, 2 out]
        n418 = property on="Reset Y Motor Steps" class="DigNum (strict)"("Val(Sgnl)"=w975) -> ()  [unwired: 2 in, 2 out]
      }
      event #2 {
        n419 = event-data() -> ()  [unwired: 1 in, 5 out]
        n420 = property on="Z Step SP" class="DigNum (strict)"() -> ("Value"=w996:i32)  [unwired: 2 in, 2 out]
        n421 = property on="Y Step SP" class="DigNum (strict)"() -> ("Value"=w1012:i32)  [unwired: 2 in, 2 out]
        n422 = property on="R Step SP" class="DigNum (strict)"() -> ("Value"=w988:i32)  [unwired: 2 in, 2 out]
        n423 = property on="X steps/rev" class="DigNum (strict)"() -> ("Value"=w1002:u32)  [unwired: 2 in, 2 out]
        n424 = property on="X steps/rev" class="DigNum (strict)"() -> ("Value"=w1029:u32)  [unwired: 2 in, 2 out]
        n425 = property on="X mm/rev" class="DigNum (strict)"() -> ("Value"=w982:dbl)  [unwired: 2 in, 2 out]
        n426 = property on="Z steps/rev" class="DigNum (strict)"() -> ("Value"=w994:u32)  [unwired: 2 in, 2 out]
        n427 = property on="Z steps/rev" class="DigNum (strict)"() -> ("Value"=w1023:u32)  [unwired: 2 in, 2 out]
        n428 = property on="Z mm/rev" class="DigNum (strict)"() -> ("Value"=w983:dbl)  [unwired: 2 in, 2 out]
        n429 = property on="Y steps/rev" class="DigNum (strict)"() -> ("Value"=w1010:u32)  [unwired: 2 in, 2 out]
        n430 = property on="Y steps/rev" class="DigNum (strict)"() -> ("Value"=w1035:u32)  [unwired: 2 in, 2 out]
        n431 = property on="Y mm/rev" class="DigNum (strict)"() -> ("Value"=w981:dbl)  [unwired: 2 in, 2 out]
        n432 = property on="R steps/rev" class="DigNum (strict)"() -> ("Value"=w986:u32)  [unwired: 2 in, 2 out]
        n433 = property on="R steps/rev" class="DigNum (strict)"() -> ("Value"=w1017:u32)  [unwired: 2 in, 2 out]
        n434 = property on="R deg/rev" class="DigNum (strict)"() -> ("Value"=w984:dbl)  [unwired: 2 in, 2 out]
        n435 = property on="X Step SP" class="DigNum (strict)"() -> ("Value"=w1004:i32)  [unwired: 2 in, 2 out]
        n436 = To Double Precision Float(number=w996) -> (double precision float=w997:dbl)
        n437 = To Double Precision Float(number=w994) -> (double precision float=w1000:dbl)
        n438 = To Double Precision Float(number=w1023) -> (double precision float=w1028:dbl)
        n439 = To Double Precision Float(number=w1012) -> (double precision float=w1013:dbl)
        n440 = To Double Precision Float(number=w1010) -> (double precision float=w1016:dbl)
        n441 = To Double Precision Float(number=w1035) -> (double precision float=w1040:dbl)
        n442 = To Double Precision Float(number=w988) -> (double precision float=w989:dbl)
        n443 = To Double Precision Float(number=w986) -> (double precision float=w992:dbl)
        n444 = To Double Precision Float(number=w1017) -> (double precision float=w1022:dbl)
        n445 = To Double Precision Float(number=w1004) -> (double precision float=w1005:dbl)
        n446 = To Double Precision Float(number=w1002) -> (double precision float=w1008:dbl)
        n447 = To Double Precision Float(number=w1029) -> (double precision float=w1034:dbl)
        n448 = property on="R Velocity SP step/sec" class="DigNum (strict)"() -> ("Value"=w1019:i32)  [unwired: 2 in, 2 out]
        n449 = property on="Z Velocity SP step/sec" class="DigNum (strict)"() -> ("Value"=w1025:i32)  [unwired: 2 in, 2 out]
        n450 = property on="Y Velocity SP step/sec" class="DigNum (strict)"() -> ("Value"=w1037:i32)  [unwired: 2 in, 2 out]
        n451 = property on="X Velocity SP step/sec" class="DigNum (strict)"() -> ("Value"=w1031:i32)  [unwired: 2 in, 2 out]
        n452 = Divide(x=w997, y=w1000) -> (x/y=w999:dbl)
        n453 = Divide(x=w1013, y=w1016) -> (x/y=w1015:dbl)
        n454 = Divide(x=w989, y=w992) -> (x/y=w991:dbl)
        n455 = Divide(x=w1005, y=w1008) -> (x/y=w1007:dbl)
        n456 = property on="R offset deg" class="DigNum (strict)"() -> ("Value"=w985:dbl)  [unwired: 2 in, 2 out]
        n457 = property on="Z offset mm" class="DigNum (strict)"() -> ("Value"=w993:dbl)  [unwired: 2 in, 2 out]
        n458 = property on="Y offset mm" class="DigNum (strict)"() -> ("Value"=w1009:dbl)  [unwired: 2 in, 2 out]
        n459 = property on="X offset mm" class="DigNum (strict)"() -> ("Value"=w1001:dbl)  [unwired: 2 in, 2 out]
        n460 = Multiply(x=w999, y=w983) -> (x*y=w998:dbl)
        n461 = Multiply(x=w1015, y=w981) -> (x*y=w1014:dbl)
        n462 = Multiply(x=w991, y=w984) -> (x*y=w990:dbl)
        n463 = Multiply(x=w1007, y=w982) -> (x*y=w1006:dbl)
        n464 = To Double Precision Float(number=w1025) -> (double precision float=w1026:dbl)
        n465 = To Double Precision Float(number=w1037) -> (double precision float=w1038:dbl)
        n466 = To Double Precision Float(number=w1019) -> (double precision float=w1020:dbl)
        n467 = To Double Precision Float(number=w1031) -> (double precision float=w1032:dbl)
        n468 = Add(x=w998, y=w993) -> (x+y=w995:dbl)
        n469 = Divide(x=w1026, y=w1028) -> (x/y=w1027:dbl)
        n470 = Add(x=w1014, y=w1009) -> (x+y=w1011:dbl)
        n471 = Divide(x=w1038, y=w1040) -> (x/y=w1039:dbl)
        n472 = Add(x=w990, y=w985) -> (x+y=w987:dbl)
        n473 = Divide(x=w1020, y=w1022) -> (x/y=w1021:dbl)
        n474 = Add(x=w1006, y=w1001) -> (x+y=w1003:dbl)
        n475 = Divide(x=w1032, y=w1034) -> (x/y=w1033:dbl)
        n476 = Multiply(x=w1027, y=w983) -> (x*y=w1024:dbl)
        n477 = Multiply(x=w1039, y=w981) -> (x*y=w1036:dbl)
        n478 = Multiply(x=w1021, y=w984) -> (x*y=w1018:dbl)
        n479 = Multiply(x=w1033, y=w982) -> (x*y=w1030:dbl)
        n480 = property on="Z Position MV mm" class="DigNum (strict)"("Val(Sgnl)"=w995) -> ()  [unwired: 2 in, 2 out]
        n481 = property on="Y Position MV mm" class="DigNum (strict)"("Val(Sgnl)"=w1011) -> ()  [unwired: 2 in, 2 out]
        n482 = property on="R Position MV deg" class="DigNum (strict)"("Val(Sgnl)"=w987) -> ()  [unwired: 2 in, 2 out]
        n483 = property on="X Position MV mm" class="DigNum (strict)"("Val(Sgnl)"=w1003) -> ()  [unwired: 2 in, 2 out]
        n484 = property on="Z Velocity MV mm/sec" class="DigNum (strict)"("Val(Sgnl)"=w1024) -> ()  [unwired: 2 in, 2 out]
        n485 = property on="Y Velocity MV mm/sec" class="DigNum (strict)"("Val(Sgnl)"=w1036) -> ()  [unwired: 2 in, 2 out]
        n486 = property on="R Velocity MVdeg/sec" class="DigNum (strict)"("Val(Sgnl)"=w1018) -> ()  [unwired: 2 in, 2 out]
        n487 = property on="X Velocity MV mm/sec" class="DigNum (strict)"("Val(Sgnl)"=w1030) -> ()  [unwired: 2 in, 2 out]
      }
      event #3 {
        n488 = event-data() -> ()  [unwired: 1 in, 5 out]
        n489 = property on="X Step SP" class="DigNum (strict)"() -> ("Maximum"=w1110:dbl)  [unwired: 2 in, 2 out]
        n490 = property on="X Step SP" class="DigNum (strict)"() -> ("Minimum"=w1111:dbl)  [unwired: 2 in, 2 out]
        n491 = property on="X Step PV" class="DigNum (strict)"() -> ("Value"=w1104:i32)  [unwired: 2 in, 2 out]
        n492 = property on="X steps/rev" class="DigNum (strict)"() -> ("Value"=w1106:u32)  [unwired: 2 in, 2 out]
        n493 = property on="X mm/rev" class="DigNum (strict)"() -> ("Value"=w1105:dbl)  [unwired: 2 in, 2 out]
        n494 = To Double Precision Float(number=w1104) -> (double precision float=w1057:dbl)
        n495 = property on="Y Step SP" class="DigNum (strict)"() -> ("Maximum"=w1096:dbl)  [unwired: 2 in, 2 out]
        n496 = property on="Y Step SP" class="DigNum (strict)"() -> ("Minimum"=w1097:dbl)  [unwired: 2 in, 2 out]
        n497 = property on="Y Step PV" class="DigNum (strict)"() -> ("Value"=w1090:i32)  [unwired: 2 in, 2 out]
        n498 = property on="Y mm/rev" class="DigNum (strict)"() -> ("Value"=w1091:dbl)  [unwired: 2 in, 2 out]
        n499 = property on="Y steps/rev" class="DigNum (strict)"() -> ("Value"=w1092:u32)  [unwired: 2 in, 2 out]
        n500 = Subtract(x=w1111, y=w1057) -> (x-y=w1112:dbl)
        n501 = Subtract(x=w1110, y=w1057) -> (x-y=w1109:dbl)
        n502 = property on="X Scan Length SP steps" class="DigNum (strict)"() -> ("Value"=w1102:i32)  [unwired: 2 in, 2 out]
        n503 = To Double Precision Float(number=w1090) -> (double precision float=w1056:dbl)
        n504 = property on="X Scan Velocity SP steps/sec" class="DigNum (strict)"() -> ("Value"=w1107:i32)  [unwired: 2 in, 2 out]
        n505 = To Double Precision Float(number=w1106) -> (double precision float=w1103:dbl)
        n506 = To Double Precision Float(number=w1102) -> (double precision float=w1042:dbl)
        n507 = property on="X Scan Length SP steps" class="DigNum (strict)"("Minimum"=w1112) -> ()  [unwired: 2 in, 2 out]
        n508 = property on="X Scan Length SP steps" class="DigNum (strict)"("Maximum"=w1109) -> ()  [unwired: 2 in, 2 out]
        n509 = property on="R Step SP" class="DigNum (strict)"() -> ("Minimum"=w1068:dbl)  [unwired: 2 in, 2 out]
        n510 = property on="Z Step SP" class="DigNum (strict)"() -> ("Maximum"=w1083:dbl)  [unwired: 2 in, 2 out]
        n511 = property on="Z Step SP" class="DigNum (strict)"() -> ("Minimum"=w1084:dbl)  [unwired: 2 in, 2 out]
        n512 = Subtract(x=w1096, y=w1056) -> (x-y=w1095:dbl)
        n513 = Subtract(x=w1097, y=w1056) -> (x-y=w1098:dbl)
        n514 = property on="Y Scan Length SP steps" class="DigNum (strict)"() -> ("Value"=w1093:i32)  [unwired: 2 in, 2 out]
        n515 = property on="R Step PV" class="DigNum (strict)"() -> ("Value"=w1063:i32)  [unwired: 2 in, 2 out]
        n516 = property on="R deg/rev" class="DigNum (strict)"() -> ("Value"=w1064:dbl)  [unwired: 2 in, 2 out]
        n517 = property on="R steps/rev" class="DigNum (strict)"() -> ("Value"=w1065:u32)  [unwired: 2 in, 2 out]
        n518 = property on="Z Step PV" class="DigNum (strict)"() -> ("Value"=w1077:i32)  [unwired: 2 in, 2 out]
        n519 = property on="Z mm/rev" class="DigNum (strict)"() -> ("Value"=w1078:dbl)  [unwired: 2 in, 2 out]
        n520 = property on="Z steps/rev" class="DigNum (strict)"() -> ("Value"=w1079:u32)  [unwired: 2 in, 2 out]
        n521 = Divide(x=w1042, y=w1103) -> (x/y=w1101:dbl)
        n522 = To Double Precision Float(number=w1107) -> (double precision float=w1041:dbl)
        n523 = property on="Y Scan Velocity SP steps/sec" class="DigNum (strict)"() -> ("Value"=w1089:i32)  [unwired: 2 in, 2 out]
        n524 = To Double Precision Float(number=w1092) -> (double precision float=w1047:dbl)
        n525 = To Double Precision Float(number=w1093) -> (double precision float=w1046:dbl)
        n526 = property on="Y Scan Length SP steps" class="DigNum (strict)"("Maximum"=w1095) -> ()  [unwired: 2 in, 2 out]
        n527 = property on="Y Scan Length SP steps" class="DigNum (strict)"("Minimum"=w1098) -> ()  [unwired: 2 in, 2 out]
        n528 = To Double Precision Float(number=w1063) -> (double precision float=w1054:dbl)
        n529 = property on="R Step SP" class="DigNum (strict)"() -> ("Maximum"=w1071:dbl)  [unwired: 2 in, 2 out]
        n530 = To Double Precision Float(number=w1077) -> (double precision float=w1055:dbl)
        n531 = Divide(x=w1041, y=w1103) -> (x/y=w1108:dbl)
        n532 = Multiply(x=w1105, y=w1101) -> (x*y=w1099:dbl)
        n533 = Divide(x=w1046, y=w1047) -> (x/y=w1094:dbl)
        n534 = To Double Precision Float(number=w1089) -> (double precision float=w1045:dbl)
        n535 = Subtract(x=w1068, y=w1054) -> (x-y=w1069:dbl)
        n536 = property on="R Scan Length SP steps" class="DigNum (strict)"() -> ("Value"=w1066:i32)  [unwired: 2 in, 2 out]
        n537 = Subtract(x=w1083, y=w1055) -> (x-y=w1082:dbl)
        n538 = Subtract(x=w1084, y=w1055) -> (x-y=w1085:dbl)
        n539 = property on="Z Scan Length SP steps" class="DigNum (strict)"() -> ("Value"=w1080:i32)  [unwired: 2 in, 2 out]
        n540 = Multiply(x=w1108, y=w1105) -> (x*y=w1100:dbl)
        n541 = property on="X Scan length MV mm" class="DigNum (strict)"("Val(Sgnl)"=w1099) -> ()  [unwired: 2 in, 2 out]
        n542 = property on="R Scan Velocity SP steps/sec" class="DigNum (strict)"() -> ("Value"=w1061:i32)  [unwired: 2 in, 2 out]
        n543 = Divide(x=w1045, y=w1047) -> (x/y=w1088:dbl)
        n544 = Multiply(x=w1094, y=w1091) -> (x*y=w1087:dbl)
        n545 = To Double Precision Float(number=w1065) -> (double precision float=w1062:dbl)
        n546 = To Double Precision Float(number=w1066) -> (double precision float=w1051:dbl)
        n547 = property on="R Scan Length SP steps" class="DigNum (strict)"("Minimum"=w1069) -> ()  [unwired: 2 in, 2 out]
        n548 = property on="Z Scan Velocity SP steps/sec" class="DigNum (strict)"() -> ("Value"=w1075:i32)  [unwired: 2 in, 2 out]
        n549 = To Double Precision Float(number=w1079) -> (double precision float=w1076:dbl)
        n550 = To Double Precision Float(number=w1080) -> (double precision float=w1053:dbl)
        n551 = property on="Z Scan Length SP steps" class="DigNum (strict)"("Maximum"=w1082) -> ()  [unwired: 2 in, 2 out]
        n552 = property on="Z Scan Length SP steps" class="DigNum (strict)"("Minimum"=w1085) -> ()  [unwired: 2 in, 2 out]
        n553 = Subtract(x=w1071, y=w1054) -> (x-y=w1070:dbl)
        n554 = property on="X Scan velocity MV mm/sec" class="DigNum (strict)"("Value"=w1100) -> ()  [unwired: 2 in, 2 out]
        n555 = Divide(x=w1051, y=w1062) -> (x/y=w1067:dbl)
        n556 = To Double Precision Float(number=w1061) -> (double precision float=w1050:dbl)
        n557 = Multiply(x=w1091, y=w1088) -> (x*y=w1086:dbl)
        n558 = property on="Y Scan length MV mm" class="DigNum (strict)"("Value"=w1087) -> ()  [unwired: 2 in, 2 out]
        n559 = Divide(x=w1053, y=w1076) -> (x/y=w1081:dbl)
        n560 = To Double Precision Float(number=w1075) -> (double precision float=w1052:dbl)
        n561 = property on="R Scan Length SP steps" class="DigNum (strict)"("Maximum"=w1070) -> ()  [unwired: 2 in, 2 out]
        n562 = property on="Y Scan velocity MV mm/sec" class="DigNum (strict)"("Val(Sgnl)"=w1086) -> ()  [unwired: 2 in, 2 out]
        n563 = Divide(x=w1050, y=w1062) -> (x/y=w1060:dbl)
        n564 = Multiply(x=w1067, y=w1064) -> (x*y=w1059:dbl)
        n565 = Divide(x=w1052, y=w1076) -> (x/y=w1074:dbl)
        n566 = Multiply(x=w1081, y=w1078) -> (x*y=w1073:dbl)
        n567 = Multiply(x=w1064, y=w1060) -> (x*y=w1058:dbl)
        n568 = Divide(x=w1042, y=w1041) -> (x/y=→"X Scan Duration":dbl)
        n569 = property on="R Scan length MV deg" class="DigNum (strict)"("Value"=w1059) -> ()  [unwired: 2 in, 2 out]
        n570 = Multiply(x=w1078, y=w1074) -> (x*y=w1072:dbl)
        n571 = property on="Z Scan length MV mm" class="DigNum (strict)"("Value"=w1073) -> ()  [unwired: 2 in, 2 out]
        n572 = Divide(x=w1046, y=w1045) -> (x/y=→"Y Scan Duration":dbl)
        n573 = property on="R Scan Velocity SP deg/sec" class="DigNum (strict)"("Val(Sgnl)"=w1058) -> ()  [unwired: 2 in, 2 out]
        n574 = property on="Z Scan velocity MV mm/sec" class="DigNum (strict)"("Val(Sgnl)"=w1072) -> ()  [unwired: 2 in, 2 out]
        n575 = Divide(x=w1053, y=w1052) -> (x/y=→"Z Scan Duration":dbl)
        n576 = Divide(x=w1051, y=w1050) -> (x/y=→"R Scan Duration":dbl)
      }
      event #4 {
        n577 = event-data() -> ()  [unwired: 1 in, 7 out]
        n578 = property on="Y steps/rev" class="DigNum (strict)"() -> ("Value"=w1129:u32)  [unwired: 2 in, 2 out]
        n579 = property on="Y offset mm" class="DigNum (strict)"() -> ("Value"=w1127:dbl)  [unwired: 2 in, 2 out]
        n580 = property on="Y Position SP mm" class="DigNum (strict)"() -> ("Value"=w1126:dbl)  [unwired: 2 in, 2 out]
        n581 = property on="Y Velocity SP step/sec" class="DigNum (strict)"() -> ("Maximum"=w1116:dbl)  [unwired: 2 in, 2 out]
        n582 = property on="Y Velocity SP step/sec" class="DigNum (strict)"() -> ("Minimum"=w1115:dbl)  [unwired: 2 in, 2 out]
        n583 = Subtract(x=w1126, y=w1127) -> (x-y=w1130:dbl)
        n584 = property on="Y Velocity SP mm/sec" class="DigNum (strict)"() -> ("Value"=w1120:dbl)  [unwired: 2 in, 2 out]
        n585 = property on="Y mm/rev" class="DigNum (strict)"() -> ("Value"=w1113:dbl)  [unwired: 2 in, 2 out]
        n586 = Divide(x=w1130, y=w1113) -> (x/y=w1131:dbl)
        n587 = Divide(x=w1120, y=w1113) -> (x/y=w1121:dbl)
        n588 = To Double Precision Float(number=w1129) -> (double precision float=w1114:dbl)
        n589 = Multiply(x=w1131, y=w1114) -> (x*y=w1125:dbl)
        n590 = Multiply(x=w1121, y=w1114) -> (x*y=w1118:dbl)
        n591 = property on="Y Step SP" class="DigNum (strict)"() -> ("Maximum"=w1123:dbl)  [unwired: 2 in, 2 out]
        n592 = property on="Y Step SP" class="DigNum (strict)"() -> ("Minimum"=w1122:dbl)  [unwired: 2 in, 2 out]
        n593 = In Range and Coerce(upper limit=w1116, x=w1118, lower limit=w1115) -> (coerced(x)=w1117:dbl)  [unwired: 1 out]
        n594 = To Long Integer(number=w1117) -> (32bit integer=w1119:i32)
        n595 = In Range and Coerce(upper limit=w1123, x=w1125, lower limit=w1122) -> (coerced(x)=w1124:dbl)  [unwired: 1 out]
        n596 = To Long Integer(number=w1124) -> (32bit integer=w1128:i32)
        n597 = property on="Y Velocity SP step/sec" class="DigNum (strict)"("Val(Sgnl)"=w1119) -> ()  [unwired: 2 in, 2 out]
        n598 = property on="Y Step SP" class="DigNum (strict)"("Val(Sgnl)"=w1128) -> ()  [unwired: 2 in, 2 out]
      }
      event #5 {
        n599 = event-data() -> ()  [unwired: 1 in, 7 out]
        n600 = property on="X steps/rev" class="DigNum (strict)"() -> ("Value"=w1148:u32)  [unwired: 2 in, 2 out]
        n601 = property on="X offset mm" class="DigNum (strict)"() -> ("Value"=w1146:dbl)  [unwired: 2 in, 2 out]
        n602 = property on="X Position SP mm" class="DigNum (strict)"() -> ("Value"=w1145:dbl)  [unwired: 2 in, 2 out]
        n603 = property on="X Velocity SP step/sec" class="DigNum (strict)"() -> ("Maximum"=w1135:dbl)  [unwired: 2 in, 2 out]
        n604 = property on="X Velocity SP step/sec" class="DigNum (strict)"() -> ("Minimum"=w1134:dbl)  [unwired: 2 in, 2 out]
        n605 = Subtract(x=w1145, y=w1146) -> (x-y=w1149:dbl)
        n606 = property on="X Velocity SP mm/sec" class="DigNum (strict)"() -> ("Value"=w1139:dbl)  [unwired: 2 in, 2 out]
        n607 = property on="X mm/rev" class="DigNum (strict)"() -> ("Value"=w1132:dbl)  [unwired: 2 in, 2 out]
        n608 = Divide(x=w1149, y=w1132) -> (x/y=w1150:dbl)
        n609 = Divide(x=w1139, y=w1132) -> (x/y=w1140:dbl)
        n610 = To Double Precision Float(number=w1148) -> (double precision float=w1133:dbl)
        n611 = Multiply(x=w1150, y=w1133) -> (x*y=w1144:dbl)
        n612 = Multiply(x=w1140, y=w1133) -> (x*y=w1137:dbl)
        n613 = property on="X Step SP" class="DigNum (strict)"() -> ("Maximum"=w1142:dbl)  [unwired: 2 in, 2 out]
        n614 = property on="X Step SP" class="DigNum (strict)"() -> ("Minimum"=w1141:dbl)  [unwired: 2 in, 2 out]
        n615 = In Range and Coerce(upper limit=w1135, x=w1137, lower limit=w1134) -> (coerced(x)=w1136:dbl)  [unwired: 1 out]
        n616 = To Long Integer(number=w1136) -> (32bit integer=w1138:i32)
        n617 = In Range and Coerce(upper limit=w1142, x=w1144, lower limit=w1141) -> (coerced(x)=w1143:dbl)  [unwired: 1 out]
        n618 = To Long Integer(number=w1143) -> (32bit integer=w1147:i32)
        n619 = property on="X Velocity SP step/sec" class="DigNum (strict)"("Val(Sgnl)"=w1138) -> ()  [unwired: 2 in, 2 out]
        n620 = property on="X Step SP" class="DigNum (strict)"("Val(Sgnl)"=w1147) -> ()  [unwired: 2 in, 2 out]
      }
      event #6 {
        n621 = event-data() -> ()  [unwired: 1 in, 7 out]
        n622 = property on="Z steps/rev" class="DigNum (strict)"() -> ("Value"=w1165:u32)  [unwired: 2 in, 2 out]
        n623 = property on="Z offset mm" class="DigNum (strict)"() -> ("Value"=w1163:dbl)  [unwired: 2 in, 2 out]
        n624 = property on="Z Position SP mm" class="DigNum (strict)"() -> ("Value"=w1162:dbl)  [unwired: 2 in, 2 out]
        n625 = property on="Z Velocity SP step/sec" class="DigNum (strict)"() -> ("Maximum"=w1152:dbl)  [unwired: 2 in, 2 out]
        n626 = property on="Z Velocity SP step/sec" class="DigNum (strict)"() -> ("Minimum"=w1151:dbl)  [unwired: 2 in, 2 out]
        n627 = Subtract(x=w1162, y=w1163) -> (x-y=w1166:dbl)
        n628 = property on="Z Velocity SP mm/sec" class="DigNum (strict)"() -> ("Value"=w1156:dbl)  [unwired: 2 in, 2 out]
        n629 = property on="Z mm/rev" class="DigNum (strict)"() -> ("Value"=w1168:dbl)  [unwired: 2 in, 2 out]
        n630 = Divide(x=w1166, y=w1168) -> (x/y=w1167:dbl)
        n631 = Divide(x=w1156, y=w1168) -> (x/y=w1157:dbl)
        n632 = To Double Precision Float(number=w1165) -> (double precision float=w1169:dbl)
        n633 = Multiply(x=w1167, y=w1169) -> (x*y=w1161:dbl)
        n634 = Multiply(x=w1157, y=w1169) -> (x*y=w1154:dbl)
        n635 = property on="Z Step SP" class="DigNum (strict)"() -> ("Maximum"=w1159:dbl)  [unwired: 2 in, 2 out]
        n636 = property on="Z Step SP" class="DigNum (strict)"() -> ("Minimum"=w1158:dbl)  [unwired: 2 in, 2 out]
        n637 = In Range and Coerce(upper limit=w1152, x=w1154, lower limit=w1151) -> (coerced(x)=w1153:dbl)  [unwired: 1 out]
        n638 = To Long Integer(number=w1153) -> (32bit integer=w1155:i32)
        n639 = In Range and Coerce(upper limit=w1159, x=w1161, lower limit=w1158) -> (coerced(x)=w1160:dbl)  [unwired: 1 out]
        n640 = To Long Integer(number=w1160) -> (32bit integer=w1164:i32)
        n641 = property on="Z Velocity SP step/sec" class="DigNum (strict)"("Val(Sgnl)"=w1155) -> ()  [unwired: 2 in, 2 out]
        n642 = property on="Z Step SP" class="DigNum (strict)"("Val(Sgnl)"=w1164) -> ()  [unwired: 2 in, 2 out]
      }
      event #7 {
        n643 = event-data() -> ()  [unwired: 1 in, 7 out]
        n644 = property on="R steps/rev" class="DigNum (strict)"() -> ("Value"=w1186:u32)  [unwired: 2 in, 2 out]
        n645 = property on="R offset deg" class="DigNum (strict)"() -> ("Value"=w1184:dbl)  [unwired: 2 in, 2 out]
        n646 = property on="R Position SP deg" class="DigNum (strict)"() -> ("Value"=w1183:dbl)  [unwired: 2 in, 2 out]
        n647 = property on="R Velocity SP step/sec" class="DigNum (strict)"() -> ("Maximum"=w1173:dbl)  [unwired: 2 in, 2 out]
        n648 = property on="R Velocity SP step/sec" class="DigNum (strict)"() -> ("Minimum"=w1172:dbl)  [unwired: 2 in, 2 out]
        n649 = Subtract(x=w1183, y=w1184) -> (x-y=w1187:dbl)
        n650 = property on="R Velocity SP deg/sec" class="DigNum (strict)"() -> ("Value"=w1177:dbl)  [unwired: 2 in, 2 out]
        n651 = property on="R deg/rev" class="DigNum (strict)"() -> ("Value"=w1170:dbl)  [unwired: 2 in, 2 out]
        n652 = Divide(x=w1187, y=w1170) -> (x/y=w1188:dbl)
        n653 = Divide(x=w1177, y=w1170) -> (x/y=w1178:dbl)
        n654 = To Double Precision Float(number=w1186) -> (double precision float=w1171:dbl)
        n655 = Multiply(x=w1188, y=w1171) -> (x*y=w1182:dbl)
        n656 = Multiply(x=w1178, y=w1171) -> (x*y=w1175:dbl)
        n657 = property on="R Step SP" class="DigNum (strict)"() -> ("Maximum"=w1180:dbl)  [unwired: 2 in, 2 out]
        n658 = property on="R Step SP" class="DigNum (strict)"() -> ("Minimum"=w1179:dbl)  [unwired: 2 in, 2 out]
        n659 = In Range and Coerce(upper limit=w1173, x=w1175, lower limit=w1172) -> (coerced(x)=w1174:dbl)  [unwired: 1 out]
        n660 = To Long Integer(number=w1174) -> (32bit integer=w1176:i32)
        n661 = In Range and Coerce(upper limit=w1180, x=w1182, lower limit=w1179) -> (coerced(x)=w1181:dbl)  [unwired: 1 out]
        n662 = To Long Integer(number=w1181) -> (32bit integer=w1185:i32)
        n663 = property on="R Velocity SP step/sec" class="DigNum (strict)"("Val(Sgnl)"=w1176) -> ()  [unwired: 2 in, 2 out]
        n664 = property on="R Step SP" class="DigNum (strict)"("Val(Sgnl)"=w1185) -> ()  [unwired: 2 in, 2 out]
      }
      event #8 {
        n665 = event-data() -> ()  [unwired: 1 in, 7 out]
        n666 = property on="Y steps/rev" class="DigNum (strict)"() -> ("Value"=w1204:u32)  [unwired: 2 in, 2 out]
        n667 = property on="Y mm/rev" class="DigNum (strict)"() -> ("Value"=w1189:dbl)  [unwired: 2 in, 2 out]
        n668 = property on="Y Scan Length SP mm" class="DigNum (strict)"() -> ("Value"=w1202:dbl)  [unwired: 2 in, 2 out]
        n669 = property on="Y Scan Velocity SP mm/sec" class="DigNum (strict)"() -> ("Value"=w1196:dbl)  [unwired: 2 in, 2 out]
        n670 = property on="Y Scan Velocity SP steps/sec" class="DigNum (strict)"() -> ("Maximum"=w1192:dbl)  [unwired: 2 in, 2 out]
        n671 = property on="Y Scan Velocity SP steps/sec" class="DigNum (strict)"() -> ("Minimum"=w1191:dbl)  [unwired: 2 in, 2 out]
        n672 = Divide(x=w1202, y=w1189) -> (x/y=w1205:dbl)
        n673 = Divide(x=w1196, y=w1189) -> (x/y=w1197:dbl)
        n674 = To Double Precision Float(number=w1204) -> (double precision float=w1190:dbl)
        n675 = Multiply(x=w1205, y=w1190) -> (x*y=w1201:dbl)
        n676 = Multiply(x=w1197, y=w1190) -> (x*y=w1194:dbl)
        n677 = property on="Y Step SP" class="DigNum (strict)"() -> ("Maximum"=w1198:dbl)  [unwired: 2 in, 2 out]
        n678 = property on="Y Step SP" class="DigNum (strict)"() -> ("Minimum"=w1199:dbl)  [unwired: 2 in, 2 out]
        n679 = In Range and Coerce(upper limit=w1192, x=w1194, lower limit=w1191) -> (coerced(x)=w1193:dbl)  [unwired: 1 out]
        n680 = To Long Integer(number=w1193) -> (32bit integer=w1195:i32)
        n681 = In Range and Coerce(upper limit=w1198, x=w1201, lower limit=w1199) -> (coerced(x)=w1200:dbl)  [unwired: 1 out]
        n682 = To Long Integer(number=w1200) -> (32bit integer=w1203:i32)
        n683 = property on="Y Scan Velocity SP steps/sec" class="DigNum (strict)"("Val(Sgnl)"=w1195) -> ()  [unwired: 2 in, 2 out]
        n684 = property on="Y Scan Length SP steps" class="DigNum (strict)"("Val(Sgnl)"=w1203) -> ()  [unwired: 2 in, 2 out]
      }
      event #9 {
        n685 = event-data() -> ()  [unwired: 1 in, 7 out]
        n686 = property on="X steps/rev" class="DigNum (strict)"() -> ("Value"=w1221:u32)  [unwired: 2 in, 2 out]
        n687 = property on="X mm/rev" class="DigNum (strict)"() -> ("Value"=w1206:dbl)  [unwired: 2 in, 2 out]
        n688 = property on="X Scan Length SP mm" class="DigNum (strict)"() -> ("Value"=w1219:dbl)  [unwired: 2 in, 2 out]
        n689 = property on="X Scan Velocity SP mm/sec" class="DigNum (strict)"() -> ("Value"=w1213:dbl)  [unwired: 2 in, 2 out]
        n690 = property on="X Scan Velocity SP steps/sec" class="DigNum (strict)"() -> ("Maximum"=w1209:dbl)  [unwired: 2 in, 2 out]
        n691 = property on="X Scan Velocity SP steps/sec" class="DigNum (strict)"() -> ("Minimum"=w1208:dbl)  [unwired: 2 in, 2 out]
        n692 = Divide(x=w1219, y=w1206) -> (x/y=w1222:dbl)
        n693 = Divide(x=w1213, y=w1206) -> (x/y=w1214:dbl)
        n694 = To Double Precision Float(number=w1221) -> (double precision float=w1207:dbl)
        n695 = Multiply(x=w1222, y=w1207) -> (x*y=w1218:dbl)
        n696 = Multiply(x=w1214, y=w1207) -> (x*y=w1211:dbl)
        n697 = property on="X Step SP" class="DigNum (strict)"() -> ("Maximum"=w1215:dbl)  [unwired: 2 in, 2 out]
        n698 = property on="X Step SP" class="DigNum (strict)"() -> ("Minimum"=w1216:dbl)  [unwired: 2 in, 2 out]
        n699 = In Range and Coerce(upper limit=w1209, x=w1211, lower limit=w1208) -> (coerced(x)=w1210:dbl)  [unwired: 1 out]
        n700 = To Long Integer(number=w1210) -> (32bit integer=w1212:i32)
        n701 = In Range and Coerce(upper limit=w1215, x=w1218, lower limit=w1216) -> (coerced(x)=w1217:dbl)  [unwired: 1 out]
        n702 = To Long Integer(number=w1217) -> (32bit integer=w1220:i32)
        n703 = property on="X Scan Velocity SP steps/sec" class="DigNum (strict)"("Val(Sgnl)"=w1212) -> ()  [unwired: 2 in, 2 out]
        n704 = property on="X Scan Length SP steps" class="DigNum (strict)"("Val(Sgnl)"=w1220) -> ()  [unwired: 2 in, 2 out]
      }
      event #10 {
        n705 = event-data() -> ()  [unwired: 1 in, 7 out]
        n706 = property on="Z steps/rev" class="DigNum (strict)"() -> ("Value"=w1238:u32)  [unwired: 2 in, 2 out]
        n707 = property on="Z mm/rev" class="DigNum (strict)"() -> ("Value"=w1223:dbl)  [unwired: 2 in, 2 out]
        n708 = property on="Z Scan Length SP mm" class="DigNum (strict)"() -> ("Value"=w1236:dbl)  [unwired: 2 in, 2 out]
        n709 = property on="Z Scan Velocity SP mm/sec" class="DigNum (strict)"() -> ("Value"=w1230:dbl)  [unwired: 2 in, 2 out]
        n710 = property on="Z Scan Velocity SP steps/sec" class="DigNum (strict)"() -> ("Maximum"=w1226:dbl)  [unwired: 2 in, 2 out]
        n711 = property on="Z Scan Velocity SP steps/sec" class="DigNum (strict)"() -> ("Minimum"=w1225:dbl)  [unwired: 2 in, 2 out]
        n712 = Divide(x=w1236, y=w1223) -> (x/y=w1239:dbl)
        n713 = Divide(x=w1230, y=w1223) -> (x/y=w1231:dbl)
        n714 = To Double Precision Float(number=w1238) -> (double precision float=w1224:dbl)
        n715 = Multiply(x=w1239, y=w1224) -> (x*y=w1235:dbl)
        n716 = Multiply(x=w1231, y=w1224) -> (x*y=w1228:dbl)
        n717 = property on="Z Step SP" class="DigNum (strict)"() -> ("Maximum"=w1232:dbl)  [unwired: 2 in, 2 out]
        n718 = property on="Z Step SP" class="DigNum (strict)"() -> ("Minimum"=w1233:dbl)  [unwired: 2 in, 2 out]
        n719 = In Range and Coerce(upper limit=w1226, x=w1228, lower limit=w1225) -> (coerced(x)=w1227:dbl)  [unwired: 1 out]
        n720 = To Long Integer(number=w1227) -> (32bit integer=w1229:i32)
        n721 = In Range and Coerce(upper limit=w1232, x=w1235, lower limit=w1233) -> (coerced(x)=w1234:dbl)  [unwired: 1 out]
        n722 = To Long Integer(number=w1234) -> (32bit integer=w1237:i32)
        n723 = property on="Z Scan Velocity SP steps/sec" class="DigNum (strict)"("Val(Sgnl)"=w1229) -> ()  [unwired: 2 in, 2 out]
        n724 = property on="Z Scan Length SP steps" class="DigNum (strict)"("Val(Sgnl)"=w1237) -> ()  [unwired: 2 in, 2 out]
      }
      event #11 {
        n725 = event-data() -> ()  [unwired: 1 in, 7 out]
        n726 = property on="R steps/rev" class="DigNum (strict)"() -> ("Value"=w1255:u32)  [unwired: 2 in, 2 out]
        n727 = property on="R Velocity SP step/sec" class="DigNum (strict)"() -> ("Maximum"=w1243:dbl)  [unwired: 2 in, 2 out]
        n728 = property on="R Scan Length SP deg" class="DigNum (strict)"() -> ("Value"=w1253:dbl)  [unwired: 2 in, 2 out]
        n729 = property on="R deg/rev" class="DigNum (strict)"() -> ("Value"=w1240:dbl)  [unwired: 2 in, 2 out]
        n730 = property on="R Scan Velocity SP steps/sec" class="DigNum (strict)"() -> ("Minimum"=w1242:dbl)  [unwired: 2 in, 2 out]
        n731 = property on="R Scan Velocity SP deg/sec" class="DigNum (strict)"() -> ("Value"=w1247:dbl)  [unwired: 2 in, 2 out]
        n732 = Divide(x=w1253, y=w1240) -> (x/y=w1256:dbl)
        n733 = To Double Precision Float(number=w1255) -> (double precision float=w1241:dbl)
        n734 = Multiply(x=w1256, y=w1241) -> (x*y=w1252:dbl)
        n735 = Divide(x=w1247, y=w1240) -> (x/y=w1248:dbl)
        n736 = property on="R Step SP" class="DigNum (strict)"() -> ("Maximum"=w1249:dbl)  [unwired: 2 in, 2 out]
        n737 = property on="R Step SP" class="DigNum (strict)"() -> ("Minimum"=w1250:dbl)  [unwired: 2 in, 2 out]
        n738 = Multiply(x=w1248, y=w1241) -> (x*y=w1245:dbl)
        n739 = In Range and Coerce(upper limit=w1249, x=w1252, lower limit=w1250) -> (coerced(x)=w1251:dbl)  [unwired: 1 out]
        n740 = In Range and Coerce(upper limit=w1243, x=w1245, lower limit=w1242) -> (coerced(x)=w1244:dbl)  [unwired: 1 out]
        n741 = To Long Integer(number=w1251) -> (32bit integer=w1254:i32)
        n742 = To Long Integer(number=w1244) -> (32bit integer=w1246:i32)
        n743 = property on="R Scan Length SP steps" class="DigNum (strict)"("Val(Sgnl)"=w1254) -> ()  [unwired: 2 in, 2 out]
        n744 = property on="R Scan Velocity SP steps/sec" class="DigNum (strict)"("Val(Sgnl)"=w1246) -> ()  [unwired: 2 in, 2 out]
      }
      event #12 {
        n745 = event-data() -> ()  [unwired: 1 in, 7 out]
        n746 = flat-sequence {
          tunnel: w1261 -> [w1271]
          tunnel: w1262 -> [w1272]
          tunnel: [w1272] -> w1258
          tunnel: [w1271] -> w1257
          tunnel: [w1275] -> w1260
          tunnel: [w1274] -> w1259
          tunnel: w1258 -> [w1277]
          tunnel: w1257 -> [w1276]
          tunnel: [w1295] -> w1264
          tunnel: [w1294] -> w1263
          tunnel: w1260 -> [w1293]
          tunnel: w1259 -> [w1292]
          tunnel: [w1302] -> w1266
          tunnel: [w1301] -> w1265
          tunnel: w1264 -> [w1300]
          tunnel: w1263 -> [w1299]
          tunnel: [w1308] -> w1267
          tunnel: [w1309] -> w1268
          tunnel: w1266 -> [w1309]
          tunnel: w1265 -> [w1307]
          frame #0 {
            n747 = property on="Scan Go" class="Bool"("DisabledEnum"=T1."Disabled and Grayed Out" ("Disabled")) -> ()  [unwired: 2 in, 2 out]
            n748 = property on="Y Go" class="Bool"("DisabledEnum"=T1."Disabled and Grayed Out" ("Disabled")) -> ()  [unwired: 2 in, 2 out]
          }
          frame #1 {
            n749 = property on="Y Step SP" class="DigNum (strict)"() -> ("Value"=w1285:i32)  [unwired: 2 in, 2 out]
            n750 = property on="Y Step PV" class="DigNum (strict)"() -> ("Value"=w1284:i32)  [unwired: 2 in, 2 out]
            n751 = property on="Y Backlash" class="DigNum (strict)"() -> ("Value"=w1273:i32)  [unwired: 2 in, 2 out]
            n752 = Subtract(x=w1285, y=w1284) -> (x-y=w1283:i32)
            n753 = Sign(1:w1273) -> (0:w1281:i32)
            n754 = Sign(1:w1283) -> (0:w1282:i32)
            n755 = Multiply(x=w1282, y=w1281) -> (x*y=w1280:i32)
            n756 = Equal?(x=w1280, y=1) -> (x = y?=w1278:bool)
            n757 = case shown="False" w1278 {
              tunnel: w1277 -> [w1288 w1290]
              tunnel: w1276 -> [w1287 w1289]
              tunnel: [w1287 w1289] -> w1275
              tunnel: [w1288 w1290] -> w1274
              frame #0 {
                n758 = property on="Y Backlash corr" class="Bool (strict)"("Val(Sgnl)"=FALSE ("Value (Signaling)")) -> ()  [unwired: 2 in, 2 out]
              }
              frame #1 {
                n759 = property on="Y Backlash corr" class="Bool (strict)"("Val(Sgnl)"=TRUE ("Value (Signaling)")) -> ()  [unwired: 2 in, 2 out]
              }
            }
          }
          frame #2 {
            # "Velocity Setting"
            n760 = property on="Y Velocity SP step/sec" class="DigNum (strict)"() -> ("Value"=w1296:i32)  [unwired: 2 in, 2 out]
            n761 = Number To Decimal String(number=w1296) -> (decimal integer string=w1297:string)  [unwired: 1 in]
            n762 = call "mDrive Send Command.vi"("error in (no error)"=w1293, "Extra"=w1297, "Command"=T2."Max Velocity", "VISA resource name"=w1292) -> ("error out"=w1294:errorcluster, "VISA resource name out"=w1295:refnum<visa-resource-name>)  [unwired: 3 in, 1 out]
          }
          frame #3 {
            # "Move to Abs Position"
            n763 = property on="Y Step SP" class="DigNum (strict)"() -> ("Value"=w1305:i32)  [unwired: 2 in, 2 out]
            n764 = Number To Decimal String(number=w1305) -> (decimal integer string=w1304:string)  [unwired: 1 in]
            n765 = call "mDrive Send Command.vi"("error in (no error)"=w1299, "Extra"=w1304, "Command"=T2."Move to Absolute Position", "VISA resource name"=w1300) -> ("error out"=w1301:errorcluster, "VISA resource name out"=w1302:refnum<visa-resource-name>)  [unwired: 3 in, 1 out]
          }
          frame #4 {
            n766 = call "Time Delay"("error in (no error)"=w1307, "Delay Time (s)"=0.1) -> ("error out"=w1308:errorcluster)  [unwired: 9 in]
          }
        }
      }
      event #13 {
        n767 = event-data() -> ()  [unwired: 1 in, 7 out]
        n768 = flat-sequence {
          tunnel: w1312 -> [w1324]
          tunnel: w1313 -> [w1325]
          tunnel: [w1325] -> w1315
          tunnel: [w1324] -> w1314
          tunnel: [w1328] -> w1317
          tunnel: [w1327] -> w1316
          tunnel: w1315 -> [w1330]
          tunnel: w1314 -> [w1329]
          tunnel: [w1348] -> w1319
          tunnel: [w1347] -> w1318
          tunnel: w1317 -> [w1346]
          tunnel: w1316 -> [w1345]
          tunnel: [w1355] -> w1321
          tunnel: [w1354] -> w1320
          tunnel: w1319 -> [w1353]
          tunnel: w1318 -> [w1352]
          tunnel: [w1361] -> w1311
          tunnel: [w1362] -> w1310
          tunnel: w1321 -> [w1362]
          tunnel: w1320 -> [w1360]
          frame #0 {
            n769 = property on="Scan Go" class="Bool"("DisabledEnum"=T1."Disabled and Grayed Out" ("Disabled")) -> ()  [unwired: 2 in, 2 out]
            n770 = property on="Z Go" class="Bool"("DisabledEnum"=T1."Disabled and Grayed Out" ("Disabled")) -> ()  [unwired: 2 in, 2 out]
          }
          frame #1 {
            n771 = property on="Z Step SP" class="DigNum (strict)"() -> ("Value"=w1338:i32)  [unwired: 2 in, 2 out]
            n772 = property on="Z Step PV" class="DigNum (strict)"() -> ("Value"=w1337:i32)  [unwired: 2 in, 2 out]
            n773 = property on="Z Backlash" class="DigNum (strict)"() -> ("Value"=w1326:i32)  [unwired: 2 in, 2 out]
            n774 = Subtract(x=w1338, y=w1337) -> (x-y=w1336:i32)
            n775 = Sign(1:w1326) -> (0:w1334:i32)
            n776 = Sign(1:w1336) -> (0:w1335:i32)
            n777 = Multiply(x=w1335, y=w1334) -> (x*y=w1333:i32)
            n778 = Equal?(x=w1333, y=1) -> (x = y?=w1331:bool)
            n779 = case shown="True" w1331 {
              tunnel: w1330 -> [w1341 w1343]
              tunnel: w1329 -> [w1340 w1342]
              tunnel: [w1340 w1342] -> w1328
              tunnel: [w1341 w1343] -> w1327
              frame #0 {
                n780 = property on="Z Backlash corr" class="Bool (strict)"("Val(Sgnl)"=FALSE ("Value (Signaling)")) -> ()  [unwired: 2 in, 2 out]
              }
              frame #1 {
                n781 = property on="Z Backlash corr" class="Bool (strict)"("Val(Sgnl)"=TRUE ("Value (Signaling)")) -> ()  [unwired: 2 in, 2 out]
              }
            }
          }
          frame #2 {
            # "Velocity Setting"
            n782 = property on="Z Velocity SP step/sec" class="DigNum (strict)"() -> ("Value"=w1349:i32)  [unwired: 2 in, 2 out]
            n783 = Number To Decimal String(number=w1349) -> (decimal integer string=w1350:string)  [unwired: 1 in]
            n784 = call "mDrive Send Command.vi"("error in (no error)"=w1346, "Extra"=w1350, "Command"=T2."Max Velocity", "VISA resource name"=w1345) -> ("error out"=w1347:errorcluster, "VISA resource name out"=w1348:refnum<visa-resource-name>)  [unwired: 3 in, 1 out]
          }
          frame #3 {
            # "Move to Abs Position"
            n785 = property on="Z Step SP" class="DigNum (strict)"() -> ("Value"=w1358:i32)  [unwired: 2 in, 2 out]
            n786 = Number To Decimal String(number=w1358) -> (decimal integer string=w1357:string)  [unwired: 1 in]
            n787 = call "mDrive Send Command.vi"("error in (no error)"=w1352, "Extra"=w1357, "Command"=T2."Move to Absolute Position", "VISA resource name"=w1353) -> ("error out"=w1354:errorcluster, "VISA resource name out"=w1355:refnum<visa-resource-name>)  [unwired: 3 in, 1 out]
          }
          frame #4 {
            n788 = call "Time Delay28"("error in (no error)"=w1360, "Delay Time (s)"=0.1) -> ("error out"=w1361:errorcluster)  [unwired: 9 in]
          }
        }
      }
      event #14 {
        n789 = event-data() -> ()  [unwired: 1 in, 7 out]
        n790 = flat-sequence {
          tunnel: w1365 -> [w1377]
          tunnel: w1366 -> [w1378]
          tunnel: [w1378] -> w1368
          tunnel: [w1377] -> w1367
          tunnel: [w1381] -> w1370
          tunnel: [w1380] -> w1369
          tunnel: w1368 -> [w1383]
          tunnel: w1367 -> [w1382]
          tunnel: [w1401] -> w1372
          tunnel: [w1400] -> w1371
          tunnel: w1370 -> [w1399]
          tunnel: w1369 -> [w1398]
          tunnel: [w1408] -> w1374
          tunnel: [w1407] -> w1373
          tunnel: w1372 -> [w1406]
          tunnel: w1371 -> [w1405]
          tunnel: [w1414] -> w1364
          tunnel: [w1415] -> w1363
          tunnel: w1374 -> [w1415]
          tunnel: w1373 -> [w1413]
          frame #0 {
            n791 = property on="Scan Go" class="Bool"("DisabledEnum"=T1."Disabled and Grayed Out" ("Disabled")) -> ()  [unwired: 2 in, 2 out]
            n792 = property on="R Go" class="Bool"("DisabledEnum"=T1."Disabled and Grayed Out" ("Disabled")) -> ()  [unwired: 2 in, 2 out]
          }
          frame #1 {
            n793 = property on="R Step SP" class="DigNum (strict)"() -> ("Value"=w1391:i32)  [unwired: 2 in, 2 out]
            n794 = property on="R Step PV" class="DigNum (strict)"() -> ("Value"=w1390:i32)  [unwired: 2 in, 2 out]
            n795 = property on="R Backlash" class="DigNum (strict)"() -> ("Value"=w1379:i32)  [unwired: 2 in, 2 out]
            n796 = Subtract(x=w1391, y=w1390) -> (x-y=w1389:i32)
            n797 = Sign(1:w1379) -> (0:w1387:i32)
            n798 = Sign(1:w1389) -> (0:w1388:i32)
            n799 = Multiply(x=w1388, y=w1387) -> (x*y=w1386:i32)
            n800 = Equal?(x=w1386, y=1) -> (x = y?=w1384:bool)
            n801 = case shown="True" w1384 {
              tunnel: w1383 -> [w1394 w1396]
              tunnel: w1382 -> [w1393 w1395]
              tunnel: [w1393 w1395] -> w1381
              tunnel: [w1394 w1396] -> w1380
              frame #0 {
                n802 = property on="R Backlash corr" class="Bool (strict)"("Val(Sgnl)"=FALSE ("Value (Signaling)")) -> ()  [unwired: 2 in, 2 out]
              }
              frame #1 {
                n803 = property on="R Backlash corr" class="Bool (strict)"("Val(Sgnl)"=TRUE ("Value (Signaling)")) -> ()  [unwired: 2 in, 2 out]
              }
            }
          }
          frame #2 {
            # "Velocity Setting"
            n804 = property on="R Velocity SP step/sec" class="DigNum (strict)"() -> ("Value"=w1402:i32)  [unwired: 2 in, 2 out]
            n805 = Number To Decimal String(number=w1402) -> (decimal integer string=w1403:string)  [unwired: 1 in]
            n806 = call "mDrive Send Command.vi"("error in (no error)"=w1399, "Extra"=w1403, "Command"=T2."Max Velocity", "VISA resource name"=w1398) -> ("error out"=w1400:errorcluster, "VISA resource name out"=w1401:refnum<visa-resource-name>)  [unwired: 3 in, 1 out]
          }
          frame #3 {
            # "Move to Abs Position"
            n807 = property on="R Step SP" class="DigNum (strict)"() -> ("Value"=w1411:i32)  [unwired: 2 in, 2 out]
            n808 = Number To Decimal String(number=w1411) -> (decimal integer string=w1410:string)  [unwired: 1 in]
            n809 = call "mDrive Send Command.vi"("error in (no error)"=w1405, "Extra"=w1410, "Command"=T2."Move to Absolute Position", "VISA resource name"=w1406) -> ("error out"=w1407:errorcluster, "VISA resource name out"=w1408:refnum<visa-resource-name>)  [unwired: 3 in, 1 out]
          }
          frame #4 {
            n810 = call "Time Delay29"("error in (no error)"=w1413, "Delay Time (s)"=0.1) -> ("error out"=w1414:errorcluster)  [unwired: 9 in]
          }
        }
      }
      event #15 {
        n811 = event-data() -> ()  [unwired: 1 in, 7 out]
        n812 = flat-sequence {
          tunnel: [w1429] -> w1421
          tunnel: [w1428] -> w1420
          tunnel: w1419 -> [w1429]
          tunnel: w1418 -> [w1428]
          tunnel: [w1434] -> w1423
          tunnel: [w1433] -> w1422
          tunnel: w1421 -> [w1436]
          tunnel: w1420 -> [w1435]
          tunnel: [w1454] -> w1425
          tunnel: [w1453] -> w1424
          tunnel: w1423 -> [w1452]
          tunnel: w1422 -> [w1451]
          tunnel: [w1461] -> w1427
          tunnel: [w1460] -> w1426
          tunnel: w1425 -> [w1459]
          tunnel: w1424 -> [w1458]
          tunnel: [w1467] -> w1416
          tunnel: [w1468] -> w1417
          tunnel: w1427 -> [w1468]
          tunnel: w1426 -> [w1466]
          frame #0 {
            n813 = property on="Scan Go" class="Bool"("DisabledEnum"=T1."Disabled and Grayed Out" ("Disabled")) -> ()  [unwired: 2 in, 2 out]
            n814 = property on="X Go" class="Bool"("DisabledEnum"=T1."Disabled and Grayed Out" ("Disabled")) -> ()  [unwired: 2 in, 2 out]
          }
          frame #1 {
            n815 = property on="X Step SP" class="DigNum (strict)"() -> ("Value"=w1444:i32)  [unwired: 2 in, 2 out]
            n816 = property on="X Step PV" class="DigNum (strict)"() -> ("Value"=w1443:i32)  [unwired: 2 in, 2 out]
            n817 = property on="X Backlash" class="DigNum (strict)"() -> ("Value"=w1432:i32)  [unwired: 2 in, 2 out]
            n818 = Subtract(x=w1444, y=w1443) -> (x-y=w1442:i32)
            n819 = Sign(1:w1432) -> (0:w1440:i32)
            n820 = Sign(1:w1442) -> (0:w1441:i32)
            n821 = Multiply(x=w1441, y=w1440) -> (x*y=w1439:i32)
            n822 = Equal?(x=w1439, y=1) -> (x = y?=w1437:bool)
            n823 = case shown="True" w1437 {
              tunnel: w1436 -> [w1447 w1449]
              tunnel: w1435 -> [w1446 w1448]
              tunnel: [w1446 w1448] -> w1434
              tunnel: [w1447 w1449] -> w1433
              frame #0 {
                n824 = property on="X Backlash corr" class="Bool (strict)"("Val(Sgnl)"=FALSE ("Value (Signaling)")) -> ()  [unwired: 2 in, 2 out]
              }
              frame #1 {
                n825 = property on="X Backlash corr" class="Bool (strict)"("Val(Sgnl)"=TRUE ("Value (Signaling)")) -> ()  [unwired: 2 in, 2 out]
              }
            }
          }
          frame #2 {
            # "Velocity Setting"
            n826 = property on="X Velocity SP step/sec" class="DigNum (strict)"() -> ("Value"=w1455:i32)  [unwired: 2 in, 2 out]
            n827 = Number To Decimal String(number=w1455) -> (decimal integer string=w1456:string)  [unwired: 1 in]
            n828 = call "mDrive Send Command.vi"("error in (no error)"=w1452, "Extra"=w1456, "Command"=T2."Max Velocity", "VISA resource name"=w1451) -> ("error out"=w1453:errorcluster, "VISA resource name out"=w1454:refnum<visa-resource-name>)  [unwired: 3 in, 1 out]
          }
          frame #3 {
            # "Move to Abs Position"
            n829 = property on="X Step SP" class="DigNum (strict)"() -> ("Value"=w1464:i32)  [unwired: 2 in, 2 out]
            n830 = Number To Decimal String(number=w1464) -> (decimal integer string=w1463:string)  [unwired: 1 in]
            n831 = call "mDrive Send Command.vi"("error in (no error)"=w1458, "Extra"=w1463, "Command"=T2."Move to Absolute Position", "VISA resource name"=w1459) -> ("error out"=w1460:errorcluster, "VISA resource name out"=w1461:refnum<visa-resource-name>)  [unwired: 3 in, 1 out]
          }
          frame #4 {
            n832 = call "Time Delay15"("error in (no error)"=w1466, "Delay Time (s)"=0.1) -> ("error out"=w1467:errorcluster)  [unwired: 9 in]
          }
        }
      }
      event #16 {
        n833 = event-data() -> ()  [unwired: 1 in, 7 out]
        n834 = flat-sequence {
          tunnel: [w1484] -> w1476
          tunnel: [w1482] -> w1475
          tunnel: w1474 -> [w1478]
          tunnel: w1473 -> [w1477]
          tunnel: w1476 -> [w1499]
          tunnel: w1475 -> [w1498]
          tunnel: [w1499] -> w1470
          tunnel: [w1498] -> w1469
          tunnel: [w1501] -> w1471
          tunnel: [w1502] -> w1472
          tunnel: w1470 -> [w1502]
          tunnel: w1469 -> [w1501]
          frame #0 {
            # "VELOCITY"
            n835 = property on="X Scan Velocity SP steps/sec" class="DigNum (strict)"() -> ("Value"=w1485:i32)  [unwired: 2 in, 2 out]
            n836 = Number To Decimal String(number=w1485) -> (decimal integer string=w1486:string)  [unwired: 1 in]
            n837 = call "mDrive Send Command.vi"("error in (no error)"=w1477, "Extra"=w1486, "Command"=T2."Max Velocity", "VISA resource name"=w1478) -> ("error out"=w1487:errorcluster, "VISA resource name out"=w1492:refnum<visa-resource-name>)  [unwired: 3 in, 1 out]
            n838 = call "Time Delay9"("error in (no error)"=w1487) -> ("error out"=w1490:errorcluster)  [unwired: 10 in]
            n839 = call "mDrive Send Command.vi"("error in (no error)"=w1490, "Extra"="VM", "Command"=T2."Print Parameter", "VISA resource name"=w1492) -> ("error out"=w1483:errorcluster, "read buffer"=w1488:string, "VISA resource name out"=w1484:refnum<visa-resource-name>)  [unwired: 3 in]
            n840 = call "Time Delay10"("error in (no error)"=w1483) -> ("error out"=w1482:errorcluster)  [unwired: 10 in]
            n841 = Decimal String To Number(string=w1488, offset=0) -> (number=w1491:i32)  [unwired: 1 in, 1 out]
            n842 = property on="X velocity PV step/sec" class="DigNum (strict)"("Val(Sgnl)"=w1491) -> ()  [unwired: 2 in, 2 out]
          }
          frame #1 {
            n843 = property on="X Scan" class="Bool (strict)"("Val(Sgnl)"=TRUE ("Slew Ready 2")) -> ()  [unwired: 2 in, 2 out]
            n844 = property on="Scan Go" class="Bool"("DisabledEnum"=T1."Enabled" ("Disabled")) -> ()  [unwired: 2 in, 2 out]
            n845 = property on="Scan Cancel" class="Bool"("DisabledEnum"=T1."Enabled" ("Disabled")) -> ()  [unwired: 2 in, 2 out]
            n846 = property on="X Scan Length SP steps" class="DigNum (strict)"("DisabledEnum"=T1."Disabled and Grayed Out" ("Disabled")) -> ()  [unwired: 2 in, 2 out]
            n847 = property on="X Scan Velocity SP steps/sec" class="DigNum (strict)"("DisabledEnum"=T1."Disabled and Grayed Out" ("Disabled")) -> ()  [unwired: 2 in, 2 out]
          }
          frame #2 {
            n848 = property on="X Go" class="Bool"("DisabledEnum"=T1."Disabled and Grayed Out" ("Disabled")) -> ()  [unwired: 2 in, 2 out]
          }
        }
      }
      event #17 {
        n849 = event-data() -> ()  [unwired: 1 in, 7 out]
        n850 = flat-sequence {
          tunnel: w1510 -> [w1520]
          tunnel: w1509 -> [w1519]
          tunnel: [w1516] -> w1507
          tunnel: [w1514] -> w1506
          tunnel: w1507 -> [w1533]
          tunnel: w1506 -> [w1532]
          tunnel: [w1533] -> w1504
          tunnel: [w1532] -> w1503
          tunnel: [w1535] -> w1508
          tunnel: [w1536] -> w1505
          tunnel: w1504 -> [w1536]
          tunnel: w1503 -> [w1535]
          frame #0 {
            # "VELOCITY"
            n851 = property on="Y Scan Velocity SP steps/sec" class="DigNum (strict)"() -> ("Value"=w1517:i32)  [unwired: 2 in, 2 out]
            n852 = Number To Decimal String(number=w1517) -> (decimal integer string=w1518:string)  [unwired: 1 in]
            n853 = call "mDrive Send Command.vi"("error in (no error)"=w1520, "Extra"=w1518, "Command"=T2."Max Velocity", "VISA resource name"=w1519) -> ("error out"=w1521:errorcluster, "VISA resource name out"=w1526:refnum<visa-resource-name>)  [unwired: 3 in, 1 out]
            n854 = call "Time Delay5"("error in (no error)"=w1521) -> ("error out"=w1524:errorcluster)  [unwired: 10 in]
            n855 = call "mDrive Send Command.vi"("error in (no error)"=w1524, "Extra"="VM", "Command"=T2."Print Parameter", "VISA resource name"=w1526) -> ("error out"=w1515:errorcluster, "read buffer"=w1522:string, "VISA resource name out"=w1516:refnum<visa-resource-name>)  [unwired: 3 in]
            n856 = call "Time Delay6"("error in (no error)"=w1515) -> ("error out"=w1514:errorcluster)  [unwired: 10 in]
            n857 = Decimal String To Number(string=w1522, offset=0) -> (number=w1525:i32)  [unwired: 1 in, 1 out]
            n858 = property on="Y velocity PV step/sec" class="DigNum (strict)"("Val(Sgnl)"=w1525) -> ()  [unwired: 2 in, 2 out]
          }
          frame #1 {
            n859 = property on="Y Scan" class="Bool (strict)"("Val(Sgnl)"=TRUE ("Slew Ready 2")) -> ()  [unwired: 2 in, 2 out]
            n860 = property on="Scan Go" class="Bool"("DisabledEnum"=T1."Enabled" ("Disabled")) -> ()  [unwired: 2 in, 2 out]
            n861 = property on="Scan Cancel" class="Bool"("DisabledEnum"=T1."Enabled" ("Disabled")) -> ()  [unwired: 2 in, 2 out]
            n862 = property on="Y Scan Length SP steps" class="DigNum (strict)"("DisabledEnum"=T1."Disabled and Grayed Out" ("Disabled")) -> ()  [unwired: 2 in, 2 out]
            n863 = property on="Y Scan Velocity SP steps/sec" class="DigNum (strict)"("DisabledEnum"=T1."Disabled and Grayed Out" ("Disabled")) -> ()  [unwired: 2 in, 2 out]
          }
          frame #2 {
            n864 = property on="Y Go" class="Bool"("DisabledEnum"=T1."Disabled and Grayed Out" ("Disabled")) -> ()  [unwired: 2 in, 2 out]
          }
        }
      }
      event #18 {
        n865 = event-data() -> ()  [unwired: 1 in, 7 out]
        n866 = flat-sequence {
          tunnel: [w1552] -> w1544
          tunnel: [w1550] -> w1543
          tunnel: w1540 -> [w1546]
          tunnel: w1539 -> [w1545]
          tunnel: w1544 -> [w1567]
          tunnel: w1543 -> [w1566]
          tunnel: [w1567] -> w1542
          tunnel: [w1566] -> w1541
          tunnel: [w1569] -> w1538
          tunnel: [w1570] -> w1537
          tunnel: w1542 -> [w1570]
          tunnel: w1541 -> [w1569]
          frame #0 {
            # "VELOCITY"
            n867 = property on="Z Scan Velocity SP steps/sec" class="DigNum (strict)"() -> ("Value"=w1553:i32)  [unwired: 2 in, 2 out]
            n868 = Number To Decimal String(number=w1553) -> (decimal integer string=w1554:string)  [unwired: 1 in]
            n869 = call "mDrive Send Command.vi"("error in (no error)"=w1545, "Extra"=w1554, "Command"=T2."Max Velocity", "VISA resource name"=w1546) -> ("error out"=w1555:errorcluster, "VISA resource name out"=w1560:refnum<visa-resource-name>)  [unwired: 3 in, 1 out]
            n870 = call "Time Delay24"("error in (no error)"=w1555) -> ("error out"=w1558:errorcluster)  [unwired: 10 in]
            n871 = call "mDrive Send Command.vi"("error in (no error)"=w1558, "Extra"="VM", "Command"=T2."Print Parameter", "VISA resource name"=w1560) -> ("error out"=w1551:errorcluster, "read buffer"=w1556:string, "VISA resource name out"=w1552:refnum<visa-resource-name>)  [unwired: 3 in]
            n872 = call "Time Delay25"("error in (no error)"=w1551) -> ("error out"=w1550:errorcluster)  [unwired: 10 in]
            n873 = Decimal String To Number(string=w1556, offset=0) -> (number=w1559:i32)  [unwired: 1 in, 1 out]
            n874 = property on="Z  velocity PV step/sec" class="DigNum (strict)"("Val(Sgnl)"=w1559) -> ()  [unwired: 2 in, 2 out]
          }
          frame #1 {
            n875 = property on="Z Scan" class="Bool (strict)"("Val(Sgnl)"=TRUE ("Slew Ready 2")) -> ()  [unwired: 2 in, 2 out]
            n876 = property on="Scan Go" class="Bool"("DisabledEnum"=T1."Enabled" ("Disabled")) -> ()  [unwired: 2 in, 2 out]
            n877 = property on="Scan Cancel" class="Bool"("DisabledEnum"=T1."Enabled" ("Disabled")) -> ()  [unwired: 2 in, 2 out]
            n878 = property on="Z Scan Length SP steps" class="DigNum (strict)"("DisabledEnum"=T1."Disabled and Grayed Out" ("Disabled")) -> ()  [unwired: 2 in, 2 out]
            n879 = property on="Z Scan Velocity SP steps/sec" class="DigNum (strict)"("DisabledEnum"=T1."Disabled and Grayed Out" ("Disabled")) -> ()  [unwired: 2 in, 2 out]
          }
          frame #2 {
            n880 = property on="Z Go" class="Bool"("DisabledEnum"=T1."Disabled and Grayed Out" ("Disabled")) -> ()  [unwired: 2 in, 2 out]
          }
        }
      }
      event #19 {
        n881 = event-data() -> ()  [unwired: 1 in, 7 out]
        n882 = flat-sequence {
          tunnel: [w1586] -> w1578
          tunnel: [w1584] -> w1577
          tunnel: w1574 -> [w1580]
          tunnel: w1573 -> [w1579]
          tunnel: w1578 -> [w1601]
          tunnel: w1577 -> [w1600]
          tunnel: [w1601] -> w1576
          tunnel: [w1600] -> w1575
          tunnel: [w1603] -> w1571
          tunnel: [w1604] -> w1572
          tunnel: w1576 -> [w1604]
          tunnel: w1575 -> [w1603]
          frame #0 {
            # "VELOCITY"
            n883 = property on="R Scan Velocity SP steps/sec" class="DigNum (strict)"() -> ("Value"=w1587:i32)  [unwired: 2 in, 2 out]
            n884 = Number To Decimal String(number=w1587) -> (decimal integer string=w1588:string)  [unwired: 1 in]
            n885 = call "mDrive Send Command.vi"("error in (no error)"=w1579, "Extra"=w1588, "Command"=T2."Max Velocity", "VISA resource name"=w1580) -> ("error out"=w1589:errorcluster, "VISA resource name out"=w1594:refnum<visa-resource-name>)  [unwired: 3 in, 1 out]
            n886 = call "Time Delay26"("error in (no error)"=w1589) -> ("error out"=w1592:errorcluster)  [unwired: 10 in]
            n887 = call "mDrive Send Command.vi"("error in (no error)"=w1592, "Extra"="VM", "Command"=T2."Print Parameter", "VISA resource name"=w1594) -> ("error out"=w1585:errorcluster, "read buffer"=w1590:string, "VISA resource name out"=w1586:refnum<visa-resource-name>)  [unwired: 3 in]
            n888 = call "Time Delay27"("error in (no error)"=w1585) -> ("error out"=w1584:errorcluster)  [unwired: 10 in]
            n889 = Decimal String To Number(string=w1590, offset=0) -> (number=w1593:i32)  [unwired: 1 in, 1 out]
            n890 = property on="R velocity PV step/sec" class="DigNum (strict)"("Val(Sgnl)"=w1593) -> ()  [unwired: 2 in, 2 out]
          }
          frame #1 {
            n891 = property on="R Scan" class="Bool (strict)"("Val(Sgnl)"=TRUE ("Slew Ready 2")) -> ()  [unwired: 2 in, 2 out]
            n892 = property on="Scan Go" class="Bool"("DisabledEnum"=T1."Enabled" ("Disabled")) -> ()  [unwired: 2 in, 2 out]
            n893 = property on="Scan Cancel" class="Bool"("DisabledEnum"=T1."Enabled" ("Disabled")) -> ()  [unwired: 2 in, 2 out]
            n894 = property on="R Scan Length SP steps" class="DigNum (strict)"("DisabledEnum"=T1."Disabled and Grayed Out" ("Disabled")) -> ()  [unwired: 2 in, 2 out]
            n895 = property on="R Scan Velocity SP steps/sec" class="DigNum (strict)"("DisabledEnum"=T1."Disabled and Grayed Out" ("Disabled")) -> ()  [unwired: 2 in, 2 out]
          }
          frame #2 {
            n896 = property on="R Go" class="Bool"("DisabledEnum"=T1."Disabled and Grayed Out" ("Disabled")) -> ()  [unwired: 2 in, 2 out]
          }
        }
      }
      event #20 {
        n897 = event-data() -> ()  [unwired: 1 in, 4 out]
        n898 = event-data() -> ()  [unwired: 3 in, 1 out]
      }
      event #21 {
        n899 = event-data() -> ()  [unwired: 1 in, 7 out]
        n900 = flat-sequence {
          tunnel: [w1637] -> w1619
          tunnel: [w1636] -> w1618
          tunnel: w1617 -> [w1635]
          tunnel: w1616 -> [w1634]
          frame #0 {
            n901 = call "mDrive Send Command.vi"("error in (no error)"=w1634, "Command"=T2."Stop", "VISA resource name"=w1635) -> ("error out"=w1636:errorcluster, "VISA resource name out"=w1637:refnum<visa-resource-name>)  [unwired: 4 in, 1 out]
          }
        }
        n902 = flat-sequence {
          tunnel: w1623 -> [w1643]
          tunnel: w1622 -> [w1642]
          tunnel: [w1641] -> w1621
          tunnel: [w1640] -> w1620
          frame #0 {
            n903 = call "mDrive Send Command.vi"("error in (no error)"=w1642, "Command"=T2."Stop", "VISA resource name"=w1643) -> ("error out"=w1640:errorcluster, "VISA resource name out"=w1641:refnum<visa-resource-name>)  [unwired: 4 in, 1 out]
          }
        }
        n904 = flat-sequence {
          tunnel: [w1632] -> w1613
          tunnel: [w1631] -> w1612
          tunnel: w1615 -> [w1630]
          tunnel: w1614 -> [w1629]
          frame #0 {
            n905 = call "mDrive Send Command.vi"("error in (no error)"=w1629, "Command"=T2."Stop", "VISA resource name"=w1630) -> ("error out"=w1631:errorcluster, "VISA resource name out"=w1632:refnum<visa-resource-name>)  [unwired: 4 in, 1 out]
          }
        }
        n906 = flat-sequence {
          tunnel: w1611 -> [w1628]
          tunnel: w1610 -> [w1627]
          tunnel: [w1626] -> w1609
          tunnel: [w1624] -> _
          tunnel: [w1624] -> w1608
          frame #0 {
            n907 = call "mDrive Send Command.vi"("error in (no error)"=w1627, "Command"=T2."Stop", "VISA resource name"=w1628) -> ("error out"=w1624:errorcluster, "VISA resource name out"=w1626:refnum<visa-resource-name>)  [unwired: 4 in, 1 out]
          }
        }
      }
      event #22 {
        n908 = event-data() -> ()  [unwired: 1 in, 7 out]
        n909 = flat-sequence {
          tunnel: w1659 -> [w1698]
          tunnel: w1658 -> [w1697]
          tunnel: [w1700] -> w1661
          tunnel: [w1699] -> w1660
          tunnel: [w1707] -> w1656
          tunnel: [w1708] -> w1657
          tunnel: w1661 -> [w1708]
          tunnel: w1660 -> [w1707]
          frame #0 {
            n910 = call "mDrive Send Command.vi"("error in (no error)"=w1697, "Command"=T2."Stop", "VISA resource name"=w1698) -> ("error out"=w1699:errorcluster, "VISA resource name out"=w1700:refnum<visa-resource-name>)  [unwired: 4 in, 1 out]
          }
          frame #1 {
            n911 = property on="X Scan" class="Bool (strict)"("Value"=FALSE ("Slew Ready")) -> ()  [unwired: 2 in, 2 out]
            n912 = property on="X Scan set" class="Bool"("DisabledEnum"=T1."Enabled" ("Disabled")) -> ()  [unwired: 2 in, 2 out]
            n913 = property on="X Scan Velocity SP steps/sec" class="DigNum (strict)"("DisabledEnum"=T1."Enabled" ("Disabled")) -> ()  [unwired: 2 in, 2 out]
            n914 = property on="X Scan Length SP steps" class="DigNum (strict)"("DisabledEnum"=T1."Enabled" ("Disabled")) -> ()  [unwired: 2 in, 2 out]
            n915 = property on="X Go" class="Bool"("DisabledEnum"=T1."Enabled" ("Disabled")) -> ()  [unwired: 2 in, 2 out]
            n916 = property on="X Scan OK" class="Bool"("DisabledEnum"=T1."Enabled" ("Disabled")) -> ()  [unwired: 2 in, 2 out]
          }
        }
        n917 = flat-sequence {
          tunnel: w1667 -> [w1711]
          tunnel: w1666 -> [w1710]
          tunnel: [w1713] -> w1663
          tunnel: [w1712] -> w1662
          tunnel: [w1720] -> w1668
          tunnel: [w1721] -> w1669
          tunnel: w1663 -> [w1721]
          tunnel: w1662 -> [w1720]
          frame #0 {
            n918 = call "mDrive Send Command.vi"("error in (no error)"=w1710, "Command"=T2."Stop", "VISA resource name"=w1711) -> ("error out"=w1712:errorcluster, "VISA resource name out"=w1713:refnum<visa-resource-name>)  [unwired: 4 in, 1 out]
          }
          frame #1 {
            n919 = property on="Y Scan" class="Bool (strict)"("Value"=FALSE ("Slew Ready")) -> ()  [unwired: 2 in, 2 out]
            n920 = property on="Y Scan Velocity SP steps/sec" class="DigNum (strict)"("DisabledEnum"=T1."Enabled" ("Disabled")) -> ()  [unwired: 2 in, 2 out]
            n921 = property on="Y Go" class="Bool"("DisabledEnum"=T1."Enabled" ("Disabled")) -> ()  [unwired: 2 in, 2 out]
            n922 = property on="Y Scan OK" class="Bool"("DisabledEnum"=T1."Enabled" ("Disabled")) -> ()  [unwired: 2 in, 2 out]
            n923 = property on="Y Scan Length SP steps" class="DigNum (strict)"("DisabledEnum"=T1."Enabled" ("Disabled")) -> ()  [unwired: 2 in, 2 out]
            n924 = property on="Y Scan set" class="Bool"("DisabledEnum"=T1."Enabled" ("Disabled")) -> ()  [unwired: 2 in, 2 out]
          }
        }
        n925 = flat-sequence {
          tunnel: [w1687] -> w1655
          tunnel: [w1686] -> w1654
          tunnel: w1653 -> [w1684]
          tunnel: w1652 -> [w1683]
          tunnel: [w1694] -> w1650
          tunnel: [w1695] -> w1651
          tunnel: w1655 -> [w1695]
          tunnel: w1654 -> [w1694]
          frame #0 {
            n926 = call "mDrive Send Command.vi"("error in (no error)"=w1683, "Command"=T2."Stop", "VISA resource name"=w1684) -> ("error out"=w1686:errorcluster, "VISA resource name out"=w1687:refnum<visa-resource-name>)  [unwired: 4 in, 1 out]
          }
          frame #1 {
            n927 = property on="Z Scan" class="Bool (strict)"("Value"=FALSE ("Slew Ready")) -> ()  [unwired: 2 in, 2 out]
            n928 = property on="Z Scan set" class="Bool"("DisabledEnum"=T1."Enabled" ("Disabled")) -> ()  [unwired: 2 in, 2 out]
            n929 = property on="Z Scan Velocity SP steps/sec" class="DigNum (strict)"("DisabledEnum"=T1."Enabled" ("Disabled")) -> ()  [unwired: 2 in, 2 out]
            n930 = property on="Z Scan Length SP steps" class="DigNum (strict)"("DisabledEnum"=T1."Enabled" ("Disabled")) -> ()  [unwired: 2 in, 2 out]
            n931 = property on="Z Go" class="Bool"("DisabledEnum"=T1."Enabled" ("Disabled")) -> ()  [unwired: 2 in, 2 out]
            n932 = property on="Z Scan OK" class="Bool"("DisabledEnum"=T1."Enabled" ("Disabled")) -> ()  [unwired: 2 in, 2 out]
          }
        }
        n933 = flat-sequence {
          tunnel: [w1674] -> w1649
          tunnel: [w1673] -> w1648
          tunnel: w1647 -> [w1671]
          tunnel: w1646 -> [w1670]
          tunnel: [w1681] -> w1644
          tunnel: [w1682] -> w1645
          tunnel: w1649 -> [w1682]
          tunnel: w1648 -> [w1681]
          frame #0 {
            n934 = call "mDrive Send Command.vi"("error in (no error)"=w1670, "Command"=T2."Stop", "VISA resource name"=w1671) -> ("error out"=w1673:errorcluster, "VISA resource name out"=w1674:refnum<visa-resource-name>)  [unwired: 4 in, 1 out]
          }
          frame #1 {
            n935 = property on="R Scan" class="Bool (strict)"("Value"=FALSE ("Slew Ready")) -> ()  [unwired: 2 in, 2 out]
            n936 = property on="R Scan OK" class="Bool"("DisabledEnum"=T1."Enabled" ("Disabled")) -> ()  [unwired: 2 in, 2 out]
            n937 = property on="R Scan Length SP steps" class="DigNum (strict)"("DisabledEnum"=T1."Enabled" ("Disabled")) -> ()  [unwired: 2 in, 2 out]
            n938 = property on="R Scan set" class="Bool"("DisabledEnum"=T1."Enabled" ("Disabled")) -> ()  [unwired: 2 in, 2 out]
            n939 = property on="R Scan Velocity SP steps/sec" class="DigNum (strict)"("DisabledEnum"=T1."Enabled" ("Disabled")) -> ()  [unwired: 2 in, 2 out]
            n940 = property on="R Go" class="Bool"("DisabledEnum"=T1."Enabled" ("Disabled")) -> ()  [unwired: 2 in, 2 out]
          }
        }
        n941 = property on="Scan Go" class="Bool"("DisabledEnum"=T1."Disabled and Grayed Out" ("Disabled")) -> ()  [unwired: 2 in, 2 out]
        n942 = property on="Scan Cancel" class="Bool"("DisabledEnum"=T1."Disabled and Grayed Out" ("Disabled")) -> ()  [unwired: 2 in, 2 out]
      }
      event #23 {
        n943 = event-data() -> ()  [unwired: 1 in, 7 out]
        n944 = flat-sequence {
          tunnel: [w1801] -> w1785
          tunnel: [w1799] -> w1778
          tunnel: [w1800] -> w1775
          tunnel: [w1794] -> w1774
          tunnel: [w1798] -> w1773
          tunnel: [w1797] -> w1772
          tunnel: [w1796] -> w1771
          tunnel: [w1795] -> w1770
          tunnel: w1749 -> [w1793]
          tunnel: [w1793] -> w1748
          tunnel: w1747 -> [w1792]
          tunnel: [w1792] -> w1746
          tunnel: w1745 -> [w1791]
          tunnel: [w1791] -> w1744
          tunnel: w1743 -> [w1790]
          tunnel: [w1790] -> w1742
          tunnel: w1741 -> [w1789]
          tunnel: [w1789] -> w1740
          tunnel: w1739 -> [w1788]
          tunnel: [w1788] -> w1738
          tunnel: [w1787] -> w1737
          tunnel: w1736 -> [w1787]
          tunnel: [w1786] -> w1735
          tunnel: w1734 -> [w1786]
          tunnel: [w1853] -> w1782
          tunnel: [w1852] -> w1780
          tunnel: w1785 -> [w1851]
          tunnel: w1778 -> [w1850]
          tunnel: [w1850] -> w1776
          tunnel: w1775 -> [w1849]
          tunnel: w1774 -> [w1838]
          tunnel: w1773 -> [w1848]
          tunnel: w1772 -> [w1844]
          tunnel: w1771 -> [w1841]
          tunnel: w1770 -> [w1847]
          tunnel: [w1846] -> w1768
          tunnel: [w1845] -> w1766
          tunnel: [w1844] -> w1763
          tunnel: [w1843] -> w1761
          tunnel: [w1842] -> w1759
          tunnel: [w1841] -> w1757
          tunnel: [w1840] -> w1755
          tunnel: [w1839] -> w1753
          tunnel: [w1838] -> w1752
          tunnel: w1748 -> [w1837]
          tunnel: w1746 -> [w1836]
          tunnel: w1744 -> [w1835]
          tunnel: w1742 -> [w1834]
          tunnel: w1740 -> [w1833]
          tunnel: w1738 -> [w1832]
          tunnel: w1737 -> [w1831]
          tunnel: w1735 -> [w1830]
          tunnel: w1782 -> [w1894]
          tunnel: [w1894] -> w1781
          tunnel: w1780 -> [w1893]
          tunnel: [w1893] -> w1779
          tunnel: [w1891] -> w1777
          tunnel: w1776 -> [w1891]
          tunnel: [w1890] -> w1769
          tunnel: w1768 -> [w1890]
          tunnel: [w1889] -> w1767
          tunnel: w1766 -> [w1889]
          tunnel: [w1888] -> w1765
          tunnel: [w1887] -> w1764
          tunnel: w1763 -> [w1887]
          tunnel: [w1886] -> w1762
          tunnel: w1761 -> [w1886]
          tunnel: [w1885] -> w1760
          tunnel: w1759 -> [w1885]
          tunnel: [w1884] -> w1758
          tunnel: w1757 -> [w1884]
          tunnel: [w1883] -> w1756
          tunnel: w1755 -> [w1883]
          tunnel: [w1882] -> w1754
          tunnel: w1753 -> [w1882]
          tunnel: w1752 -> [w1888]
          tunnel: w1781 -> [w1914]
          tunnel: [w1912] -> w1784
          tunnel: w1779 -> [w1913]
          tunnel: [w1911] -> w1783
          tunnel: w1777 -> [w1910]
          tunnel: w1769 -> [w1909]
          tunnel: w1767 -> [w1908]
          tunnel: w1765 -> [w1907]
          tunnel: w1764 -> [w1906]
          tunnel: w1762 -> [w1905]
          tunnel: w1760 -> [w1904]
          tunnel: w1758 -> [w1903]
          tunnel: w1756 -> [w1902]
          tunnel: w1754 -> [w1901]
          tunnel: [w1900] -> w1751
          tunnel: [w1899] -> w1750
          tunnel: [w1898] -> w1729
          tunnel: [w1897] -> w1726
          tunnel: [w1896] -> w1724
          tunnel: [w1895] -> w1722
          tunnel: w1784 -> [w1972]
          tunnel: w1783 -> [w1971]
          tunnel: [w1972] -> w1733
          tunnel: [w1971] -> w1732
          tunnel: [w1965] -> w1731
          tunnel: w1751 -> [w1965]
          tunnel: [w1964] -> w1730
          tunnel: w1750 -> [w1964]
          tunnel: w1729 -> [w1954]
          tunnel: [w1954] -> w1728
          tunnel: [w1953] -> w1727
          tunnel: w1726 -> [w1953]
          tunnel: [w1952] -> w1725
          tunnel: w1724 -> [w1952]
          tunnel: [w1951] -> w1723
          tunnel: w1722 -> [w1951]
          frame #0 {
            n945 = property on="X Scan" class="Bool (strict)"() -> ("Value"=w1794:bool)  [unwired: 2 in, 2 out]
            n946 = property on="Y Scan" class="Bool (strict)"() -> ("Value"=w1799:bool)  [unwired: 2 in, 2 out]
            n947 = property on="Z Scan" class="Bool (strict)"() -> ("Value"=w1796:bool)  [unwired: 2 in, 2 out]
            n948 = property on="R Scan" class="Bool (strict)"() -> ("Value"=w1797:bool)  [unwired: 2 in, 2 out]
            n949 = case shown="True" w1794 {
              tunnel: ["" w1817] -> w1800
              frame #0 {
              }
              frame #1 {
                n950 = property on="X Scan Length SP steps" class="DigNum (strict)"() -> ("Value"=w1822:i32)  [unwired: 2 in, 2 out]
                n951 = Number To Decimal String(number=w1822) -> (decimal integer string=w1819:string)  [unwired: 1 in]
                n952 = call <vilib>:"Space Constant.vi"() -> ("String"=w1820:string)
                n953 = Concatenate Strings("MR", w1820, w1819, "\r") -> (w1817:string)
              }
            }
            n954 = case shown="True" w1799 {
              tunnel: ["" w1824] -> w1801
              frame #0 {
              }
              frame #1 {
                n955 = property on="Y Scan Length SP steps" class="DigNum (strict)"() -> ("Value"=w1829:i32)  [unwired: 2 in, 2 out]
                n956 = Number To Decimal String(number=w1829) -> (decimal integer string=w1826:string)  [unwired: 1 in]
                n957 = call <vilib>:"Space Constant.vi"() -> ("String"=w1827:string)
                n958 = Concatenate Strings("MR", w1827, w1826, "\r") -> (w1824:string)
              }
            }
            n959 = case shown="True" w1796 {
              tunnel: ["" w1810] -> w1798
              frame #0 {
              }
              frame #1 {
                n960 = property on="Z Scan Length SP steps" class="DigNum (strict)"() -> ("Value"=w1815:i32)  [unwired: 2 in, 2 out]
                n961 = Number To Decimal String(number=w1815) -> (decimal integer string=w1812:string)  [unwired: 1 in]
                n962 = call <vilib>:"Space Constant.vi"() -> ("String"=w1813:string)
                n963 = Concatenate Strings("MR", w1813, w1812, "\r") -> (w1810:string)
              }
            }
            n964 = case shown="True" w1797 {
              tunnel: ["" w1803] -> w1795
              frame #0 {
              }
              frame #1 {
                n965 = property on="R Scan Length SP steps" class="DigNum (strict)"() -> ("Value"=w1808:i32)  [unwired: 2 in, 2 out]
                n966 = Number To Decimal String(number=w1808) -> (decimal integer string=w1805:string)  [unwired: 1 in]
                n967 = call <vilib>:"Space Constant.vi"() -> ("String"=w1806:string)
                n968 = Concatenate Strings("MR", w1806, w1805, "\r") -> (w1803:string)
              }
            }
          }
          frame #1 {
            n969 = case shown="False" w1838 {
              tunnel: [w1869 w1874] -> w1846
              tunnel: [w1868 w1873] -> w1845
              tunnel: w1849 -> [_ w1872]
              tunnel: w1837 -> [w1869 w1871]
              tunnel: w1836 -> [w1868 w1870]
              frame #0 {
              }
              frame #1 {
                n970 = VISA Write(VISA resource name=w1871, write buffer=w1872, error in (no error)=w1870) -> (VISA resource name out=w1874:refnum<visa-resource-name>, error out=w1873:errorcluster)  [unwired: 1 out]
              }
            }
            n971 = case shown="False" w1850 {
              tunnel: [w1876 w1881] -> w1853
              tunnel: [w1875 w1880] -> w1852
              tunnel: w1851 -> [_ w1879]
              tunnel: w1835 -> [w1876 w1878]
              tunnel: w1834 -> [w1875 w1877]
              frame #0 {
              }
              frame #1 {
                n972 = VISA Write(VISA resource name=w1878, write buffer=w1879, error in (no error)=w1877) -> (VISA resource name out=w1881:refnum<visa-resource-name>, error out=w1880:errorcluster)  [unwired: 1 out]
              }
            }
            n973 = case shown="False" w1841 {
              tunnel: [w1862 w1867] -> w1840
              tunnel: [w1861 w1866] -> w1839
              tunnel: w1848 -> [_ w1865]
              tunnel: w1833 -> [w1862 w1864]
              tunnel: w1832 -> [w1861 w1863]
              frame #0 {
              }
              frame #1 {
                n974 = VISA Write(VISA resource name=w1864, write buffer=w1865, error in (no error)=w1863) -> (VISA resource name out=w1867:refnum<visa-resource-name>, error out=w1866:errorcluster)  [unwired: 1 out]
              }
            }
            n975 = case shown="False" w1844 {
              tunnel: [w1855 w1860] -> w1843
              tunnel: [w1854 w1859] -> w1842
              tunnel: w1847 -> [_ w1858]
              tunnel: w1831 -> [w1855 w1857]
              tunnel: w1830 -> [w1854 w1856]
              frame #0 {
              }
              frame #1 {
                n976 = VISA Write(VISA resource name=w1857, write buffer=w1858, error in (no error)=w1856) -> (VISA resource name out=w1860:refnum<visa-resource-name>, error out=w1859:errorcluster)  [unwired: 1 out]
              }
            }
          }
          frame #2 {
            n977 = call "Time Delay7"("Delay Time (s)"=0.1) -> ()  [unwired: 10 in, 1 out]
          }
          frame #3 {
            n978 = case shown="True" w1907 {
              tunnel: w1909 -> [w1934 w1938]
              tunnel: w1908 -> [w1933 w1937]
              tunnel: [w1934 w1936] -> w1896
              tunnel: [w1933 w1935] -> w1895
              frame #0 {
              }
              frame #1 {
                n979 = property class="Instr"(reference=w1938, error in=w1937) -> (reference out=w1940:refnum<visa-resource-name>, error out=w1939:errorcluster, "Serial Settings:Number of Bytes at Serial Port"=w1941:u32)
                n980 = VISA Read(VISA resource name=w1940, byte count=w1941, error in (no error)=w1939) -> (VISA resource name out=w1936:refnum<visa-resource-name>, error out=w1935:errorcluster)  [unwired: 2 out]
              }
            }
            n981 = case shown="True" w1910 {
              tunnel: w1914 -> [w1943 w1947]
              tunnel: w1913 -> [w1942 w1946]
              tunnel: [w1943 w1945] -> w1912
              tunnel: [w1942 w1944] -> w1911
              frame #0 {
              }
              frame #1 {
                n982 = property class="Instr"(reference=w1947, error in=w1946) -> (reference out=w1949:refnum<visa-resource-name>, error out=w1948:errorcluster, "Serial Settings:Number of Bytes at Serial Port"=w1950:u32)
                n983 = VISA Read(VISA resource name=w1949, byte count=w1950, error in (no error)=w1948) -> (VISA resource name out=w1945:refnum<visa-resource-name>, error out=w1944:errorcluster)  [unwired: 2 out]
              }
            }
            n984 = case shown="True" w1903 {
              tunnel: w1902 -> [w1916 w1920]
              tunnel: w1901 -> [w1915 w1919]
              tunnel: [w1916 w1918] -> w1900
              tunnel: [w1915 w1917] -> w1899
              frame #0 {
              }
              frame #1 {
                n985 = property class="Instr"(reference=w1920, error in=w1919) -> (reference out=w1922:refnum<visa-resource-name>, error out=w1921:errorcluster, "Serial Settings:Number of Bytes at Serial Port"=w1923:u32)
                n986 = VISA Read(VISA resource name=w1922, byte count=w1923, error in (no error)=w1921) -> (VISA resource name out=w1918:refnum<visa-resource-name>, error out=w1917:errorcluster)  [unwired: 2 out]
              }
            }
            n987 = case shown="True" w1906 {
              tunnel: w1905 -> [w1925 w1929]
              tunnel: w1904 -> [w1924 w1928]
              tunnel: [w1925 w1927] -> w1898
              tunnel: [w1924 w1926] -> w1897
              frame #0 {
              }
              frame #1 {
                n988 = property class="Instr"(reference=w1929, error in=w1928) -> (reference out=w1931:refnum<visa-resource-name>, error out=w1930:errorcluster, "Serial Settings:Number of Bytes at Serial Port"=w1932:u32)
                n989 = VISA Read(VISA resource name=w1931, byte count=w1932, error in (no error)=w1930) -> (VISA resource name out=w1927:refnum<visa-resource-name>, error out=w1926:errorcluster)  [unwired: 2 out]
              }
            }
          }
          frame #4 {
            n990 = property on="R Scan" class="Bool (strict)"("Val(Sgnl)"=FALSE ("Slew Ready 2")) -> ()  [unwired: 2 in, 2 out]
            n991 = property on="X Scan" class="Bool (strict)"("Val(Sgnl)"=FALSE ("Slew Ready 2")) -> ()  [unwired: 2 in, 2 out]
            n992 = property on="Z Scan" class="Bool (strict)"("Val(Sgnl)"=FALSE ("Slew Ready 2")) -> ()  [unwired: 2 in, 2 out]
            n993 = property on="Y Scan Length SP steps" class="DigNum (strict)"("DisabledEnum"=T1."Enabled" ("Disabled")) -> ()  [unwired: 2 in, 2 out]
            n994 = property on="Scan Go" class="Bool"("DisabledEnum"=T1."Disabled and Grayed Out" ("Disabled")) -> ()  [unwired: 2 in, 2 out]
            n995 = property on="Y Scan" class="Bool (strict)"("Val(Sgnl)"=FALSE ("Slew Ready 2")) -> ()  [unwired: 2 in, 2 out]
            n996 = property on="Scan Cancel" class="Bool"("DisabledEnum"=T1."Disabled and Grayed Out" ("Disabled")) -> ()  [unwired: 2 in, 2 out]
            n997 = property on="Y Scan Selocity SP steps/sec" class="DigNum (strict)"("DisabledEnum"=T1."Enabled" ("Disabled")) -> ()  [unwired: 2 in, 2 out]
            n998 = property on="R Scan Length SP steps" class="DigNum (strict)"("DisabledEnum"=T1."Enabled" ("Disabled")) -> ()  [unwired: 2 in, 2 out]
            n999 = property on="X Scan Length SP steps" class="DigNum (strict)"("DisabledEnum"=T1."Enabled" ("Disabled")) -> ()  [unwired: 2 in, 2 out]
            n1000 = property on="Z Scan Length SP steps" class="DigNum (strict)"("DisabledEnum"=T1."Enabled" ("Disabled")) -> ()  [unwired: 2 in, 2 out]
            n1001 = property on="X Scan Velocity SP steps/sec" class="DigNum (strict)"("DisabledEnum"=T1."Enabled" ("Disabled")) -> ()  [unwired: 2 in, 2 out]
            n1002 = property on="R Scan Velocity SP steps/sec" class="DigNum (strict)"("DisabledEnum"=T1."Enabled" ("Disabled")) -> ()  [unwired: 2 in, 2 out]
            n1003 = property on="Z Scan Velocity SP steps/sec" class="DigNum (strict)"("DisabledEnum"=T1."Enabled" ("Disabled")) -> ()  [unwired: 2 in, 2 out]
          }
        }
      }
      event #24 {
        n1004 = event-data() -> ()  [unwired: 1 in, 7 out]
        n1005 = flat-sequence {
          tunnel: [w2003] -> w1982
          tunnel: w1983 -> [w2006]
          tunnel: [w2005] -> w1981
          tunnel: w1984 -> [w2004]
          frame #0 {
            n1006 = property on="Reset X Motor Steps" class="DigNum (strict)"() -> ("Value"=w2007:i32)  [unwired: 2 in, 2 out]
            n1007 = Number To Decimal String(number=w2007) -> (decimal integer string=w2008:string)  [unwired: 1 in]
            n1008 = call "mDrive Send Command.vi"("error in (no error)"=w2006, "Extra"=w2008, "Command"=T2."Set Current Position", "VISA resource name"=w2004) -> ("error out"=w2005:errorcluster, "VISA resource name out"=w2003:refnum<visa-resource-name>)  [unwired: 3 in, 1 out]
          }
        }
        n1009 = flat-sequence {
          tunnel: w1988 -> [w2013]
          tunnel: w1987 -> [w2012]
          tunnel: [w2011] -> w1986
          tunnel: [w2010] -> w1985
          frame #0 {
            n1010 = property on="Reset Y Motor Steps" class="DigNum (strict)"() -> ("Value"=w2014:i32)  [unwired: 2 in, 2 out]
            n1011 = Number To Decimal String(number=w2014) -> (decimal integer string=w2015:string)  [unwired: 1 in]
            n1012 = call "mDrive Send Command.vi"("error in (no error)"=w2012, "Extra"=w2015, "Command"=T2."Set Current Position", "VISA resource name"=w2013) -> ("error out"=w2010:errorcluster, "VISA resource name out"=w2011:refnum<visa-resource-name>)  [unwired: 3 in, 1 out]
          }
        }
        n1013 = flat-sequence {
          tunnel: [w1990] -> w1976
          tunnel: [w1992] -> w1975
          tunnel: w1978 -> [w1991]
          tunnel: w1977 -> [w1989]
          frame #0 {
            n1014 = property on="Reset R Motor Steps" class="DigNum (strict)"() -> ("Value"=w1993:i32)  [unwired: 2 in, 2 out]
            n1015 = Number To Decimal String(number=w1993) -> (decimal integer string=w1994:string)  [unwired: 1 in]
            n1016 = call "mDrive Send Command.vi"("error in (no error)"=w1989, "Extra"=w1994, "Command"=T2."Set Current Position", "VISA resource name"=w1991) -> ("error out"=w1992:errorcluster, "VISA resource name out"=w1990:refnum<visa-resource-name>)  [unwired: 3 in, 1 out]
          }
        }
        n1017 = flat-sequence {
          tunnel: [w1999] -> w1974
          tunnel: [w1998] -> w1973
          tunnel: w1980 -> [w1997]
          tunnel: w1979 -> [w1996]
          frame #0 {
            n1018 = property on="Reset Z Motor Steps" class="DigNum (strict)"() -> ("Value"=w2000:i32)  [unwired: 2 in, 2 out]
            n1019 = Number To Decimal String(number=w2000) -> (decimal integer string=w2001:string)  [unwired: 1 in]
            n1020 = call "mDrive Send Command.vi"("error in (no error)"=w1996, "Extra"=w2001, "Command"=T2."Set Current Position", "VISA resource name"=w1997) -> ("error out"=w1998:errorcluster, "VISA resource name out"=w1999:refnum<visa-resource-name>)  [unwired: 3 in, 1 out]
          }
        }
      }
    }
  }
  n1021 = flat-sequence {
    tunnel: w60 -> [w2021]
    tunnel: w59 -> [w2018]
    frame #0 {
      n1022 = call "mDrive Send Command.vi"("error in (no error)"=w2018, "Command"=T2."Stop", "VISA resource name"=w2021) -> ("error out"=w2019:errorcluster, "VISA resource name out"=w2020:refnum<visa-resource-name>)  [unwired: 4 in, 1 out]
      n1023 = VISA Close(VISA resource name=w2020, error in (no error)=w2019) -> ()  [unwired: 1 out]
    }
  }
  n1024 = flat-sequence {
    tunnel: w87 -> [w2026]
    tunnel: w86 -> [w2023]
    frame #0 {
      n1025 = call "mDrive Send Command.vi"("error in (no error)"=w2023, "Command"=T2."Stop", "VISA resource name"=w2026) -> ("error out"=w2024:errorcluster, "VISA resource name out"=w2025:refnum<visa-resource-name>)  [unwired: 4 in, 1 out]
      n1026 = VISA Close(VISA resource name=w2025, error in (no error)=w2024) -> ()  [unwired: 1 out]
    }
  }
  n1027 = flat-sequence {
    tunnel: w14 -> [w2031]
    tunnel: w13 -> [w2028]
    frame #0 {
      n1028 = call "mDrive Send Command.vi"("error in (no error)"=w2028, "Command"=T2."Stop", "VISA resource name"=w2031) -> ("error out"=w2029:errorcluster, "VISA resource name out"=w2030:refnum<visa-resource-name>)  [unwired: 4 in, 1 out]
      n1029 = VISA Close(VISA resource name=w2030, error in (no error)=w2029) -> ()  [unwired: 1 out]
    }
  }
  n1030 = flat-sequence {
    tunnel: w10 -> [w2036]
    tunnel: w9 -> [w2033]
    frame #0 {
      n1031 = call "mDrive Send Command.vi"("error in (no error)"=w2033, "Command"=T2."Stop", "VISA resource name"=w2036) -> ("error out"=w2034:errorcluster, "VISA resource name out"=w2035:refnum<visa-resource-name>)  [unwired: 4 in, 1 out]
      n1032 = VISA Close(VISA resource name=w2035, error in (no error)=w2034) -> ()  [unwired: 1 out]
    }
  }
  "Y COM PORT" <- w90
  "X COM PORT" <- w65
  "Z COM PORT" <- w52
  "R COM PORT" <- w19
